vi "Lab Panel V3.5.vi"() -> ()   [LabVIEW 2013]
uses:
  <vilib>/Platform/TimedLoop/XDataNode/timing_clust.ctl
  <vilib>/Platform/TimedLoop/XDataNode/nitl_modes.ctl
  <vilib>/Platform/TimedLoop/XDataNode/wakeup.ctl
  Global 1.vi
  <vilib>/platform/TimedLoop/XDataNode/XDataNode.xnode
  <vilib>/Platform/TimedLoop/XDataNode/XDNodeRunTimeDep.lvlib
panel:
  out "TEMP update":bool
  out "AI update":bool
  in  "stop":bool
  in  "Tab Control 2":T1(tab)
  out "SIG LAB05-2":T2 {"PF" format="%.2f"; "AMPS" format="%.1f"}
  out "SIG LAB05-1":T2 {"PF" format="%.2f"; "AMPS" format="%.1f"}
  out "SIG LAB04-2":T2 {"PF" format="%.2f"; "AMPS" format="%.1f"}
  out "SIG LAB04-1":T2 {"PF" format="%.2f"; "AMPS" format="%.1f"}
  out "SIG LAB03-2":T2 {"PF" format="%.2f"; "AMPS" format="%.1f"}
  out "SIG LAB03-1":T2 {"PF" format="%.2f"; "AMPS" format="%.1f"}
  out "SIG LAB02-2":T2 {"PF" format="%.2f"; "AMPS" format="%.1f"}
  in  "RUN LAB01-1":bool
  in  "O/I  LAB05-1":bool
  in  "O/I  LAB05-2":bool
  in  "O/I  LAB04-1":bool
  in  "O/I  LAB04-2":bool
  in  "O/I  LAB02-1":bool
  in  "O/I  LAB02-2":bool
  in  "O/I  LAB01-2":bool
  in  "O/I  LAB01-1":bool
  in  "O/I  LAB03-1":bool
  in  "RUN LAB05-2":bool
  in  "RUN LAB05-1":bool
  in  "RUN LAB04-2":bool
  in  "RUN LAB04-1":bool
  in  "RUN LAB03-2":bool
  in  "RUN LAB03-1":bool
  in  "RUN LAB02-2":bool
  in  "RUN LAB02-1":bool
  in  "RUN LAB01-2":bool
  in  "SELECT LAB05-2":T3(radio)
  in  "SELECT LAB05-1":T3(radio)
  in  "SELECT LAB04-2":T3(radio)
  in  "SELECT LAB04-1":T3(radio)
  in  "SELECT LAB03-2":T3(radio)
  in  "SELECT LAB03-1":T3(radio)
  in  "SELECT LAB02-2":T3(radio)
  in  "SELECT LAB02-1":T3(radio)
  in  "SELECT LAB01-2":T3(radio)
  in  "SELECT LAB01-1":T3(radio)
  in  "O/I  LAB03-2":bool
  out "SIG LAB01-1":T2 {"PF" format="%.2f"; "AMPS" format="%.1f"}
  out "SIG LAB01-2":T2 {"PF" format="%.2f"; "AMPS" format="%.1f"}
  out "SIG LAB02-1":T2 {"PF" format="%.2f"; "AMPS" format="%.1f"}
  out "DISP LAB05-2":T4 {"MINS" format="%.2g"}
  out "DISP LAB05-1":T4 {"MINS" format="%.2g"}
  out "DISP LAB04-2":T4 {"MINS" format="%.2g"}
  out "DISP LAB04-1":T4 {"MINS" format="%.2g"}
  out "DISP LAB03-2":T4 {"MINS" format="%.2g"}
  out "DISP LAB03-1":T4 {"MINS" format="%.2g"}
  in  "SET LAB05-2":T5={"NAME"="", "DESCRIPTION"="", "CYCLES"=5.0, "T-RISE mins"=0.0, "T-RISE deg C"=0.0} {"CYCLES" min=5.0 step=1.0}
  in  "SET LAB05-1":T5={"NAME"="", "DESCRIPTION"="", "CYCLES"=5.0, "T-RISE mins"=0.0, "T-RISE deg C"=0.0} {"CYCLES" min=5.0 step=1.0}
  in  "SET LAB04-2":T5={"NAME"="", "DESCRIPTION"="", "CYCLES"=5.0, "T-RISE mins"=0.0, "T-RISE deg C"=0.0} {"CYCLES" min=5.0 step=1.0}
  in  "SET LAB04-1":T5={"NAME"="", "DESCRIPTION"="", "CYCLES"=5.0, "T-RISE mins"=0.0, "T-RISE deg C"=0.0} {"CYCLES" min=5.0 step=1.0}
  in  "SET LAB03-2":T5={"NAME"="", "DESCRIPTION"="", "CYCLES"=5.0, "T-RISE mins"=0.0, "T-RISE deg C"=0.0} {"CYCLES" min=5.0 step=1.0}
  in  "SET LAB03-1":T5={"NAME"="", "DESCRIPTION"="", "CYCLES"=5.0, "T-RISE mins"=0.0, "T-RISE deg C"=0.0} {"CYCLES" min=5.0 step=1.0}
  out "DISP LAB02-2":T4 {"MINS" format="%.2g"}
  out "DISP LAB02-1":T4 {"MINS" format="%.2g"}
  in  "SET LAB02-2":T5={"NAME"="", "DESCRIPTION"="", "CYCLES"=5.0, "T-RISE mins"=0.0, "T-RISE deg C"=0.0} {"CYCLES" min=5.0 step=1.0}
  in  "SET LAB02-1":T5={"NAME"="", "DESCRIPTION"="", "CYCLES"=5.0, "T-RISE mins"=0.0, "T-RISE deg C"=0.0} {"CYCLES" min=5.0 step=1.0}
  out "RESULT LAB05-2":bool
  out "RESULT LAB05-1":bool
  out "RESULT LAB04-2":bool
  out "RESULT LAB04-1":bool
  out "RESULT LAB03-2":bool
  out "RESULT LAB03-1":bool
  out "RESULT LAB02-2":bool
  out "RESULT LAB02-1":bool
  out "RESULT LAB01-2":bool
  out "RESULT LAB01-1":bool
  in  "SET LAB01-1":T5={"NAME"="", "DESCRIPTION"="", "CYCLES"=5.0, "T-RISE mins"=0.0, "T-RISE deg C"=0.0} {"CYCLES" min=5.0 step=1.0}
  in  "SET LAB01-2":T5={"NAME"="", "DESCRIPTION"="", "CYCLES"=5.0, "T-RISE mins"=0.0, "T-RISE deg C"=0.0} {"CYCLES" min=5.0 step=1.0}
  out "DISP LAB01-1":T4 {"MINS" format="%.2g"}
  out "DISP LAB01-2":T4 {"MINS" format="%.2f"}
  out "TEMP RISE LAB05-2":cluster{"TL":dbl, "TN":dbl}
  out "TEMP RISE LAB05-1":cluster{"TL":dbl, "TN":dbl}
  out "TEMP RISE LAB04-2":cluster{"TL":dbl, "TN":dbl}
  out "TEMP RISE LAB04-1":cluster{"TL":dbl, "TN":dbl}
  out "TEMP RISE LAB03-2":cluster{"TL":dbl, "TN":dbl}
  out "TEMP RISE LAB03-1":cluster{"TL":dbl, "TN":dbl}
  out "TEMP RISE LAB02-2":cluster{"TL":dbl, "TN":dbl}
  out "TEMP RISE LAB02-1":cluster{"TL":dbl, "TN":dbl}
  out "TEMP RISE LAB01-2":cluster{"TL":dbl, "TN":dbl}
  out "TEMP RISE LAB01-1":cluster{"TL":dbl, "TN":dbl}
  in  "JIG OFF TIME (S)":dbl=2.0 min=2.0 max=10.0 step=0.5 format="%.1g"
  in  "JIG ON TIME (S)":dbl=1.0 min=1.0 max=10.0 step=0.5 format="%.1g"
  out "JIG LAB05-2":bool
  out "JIG LAB05-1":bool
  out "JIG LAB04-2":bool
  out "JIG LAB04-1":bool
  out "JIG LAB03-2":bool
  out "JIG LAB03-1":bool
  out "JIG LAB02-2":bool
  out "JIG LAB02-1":bool
  out "JIG LAB01-2":bool
  out "JIG LAB01-1":bool
  out "TEMP START LAB01-1":cluster{"TL":dbl, "TN":dbl}
  out "TEMP START LAB02-1":cluster{"TL":dbl, "TN":dbl}
  out "TEMP START LAB03-1":cluster{"TL":dbl, "TN":dbl}
  out "TEMP START LAB04-1":cluster{"TL":dbl, "TN":dbl}
  out "TEMP START LAB01-2":cluster{"TL":dbl, "TN":dbl}
  out "TEMP START LAB02-2":cluster{"TL":dbl, "TN":dbl}
  out "TEMP START LAB03-2":cluster{"TL":dbl, "TN":dbl}
  out "TEMP START LAB04-2":cluster{"TL":dbl, "TN":dbl}
  out "TEMP START LAB05-2":cluster{"TL":dbl, "TN":dbl}
  out "TEMP START LAB05-1":cluster{"TL":dbl, "TN":dbl}
  in  "MAIL SETTINGS":T6
  out "MAIL REPORT":string
  in  "TO (string):":string
  in  "Send Mail Now":bool
  in  "Auto Mail Send":bool
  in  "Network Directory":path
  out "CAL LAB01":T7 {"2 (TN) cal" min=0.0 step=0.01 format="%.2f"; "2 (TL) cal" min=0.0 step=0.01 format="%.2f"; "2 (PF) cal" min=0.0 step=0.01 format="%.2f"; "2 (V) cal" min=0.0 step=0.01 format="%.2f"; "2 (A) cal" min=0.0 step=0.01 format="%.2f"; "1 (TN) cal" min=0.0 step=0.01 format="%.2f"; "1 (TL) cal" min=0.0 step=0.01 format="%.2f"; "1 (PF) cal" min=0.0 step=0.01 format="%.2f"; "1 (V) cal" min=0.0 step=0.01 format="%.2f"; "1  (A) cal" min=0.0 step=0.01 format="%.2f"}
  out "CAL LAB03":T7 {"2 (TN) cal" min=0.0 step=0.01 format="%.2f"; "2 (TL) cal" min=0.0 step=0.01 format="%.2f"; "2 (PF) cal" min=0.0 step=0.01 format="%.2f"; "2 (V) cal" min=0.0 step=0.01 format="%.2f"; "2 (A) cal" min=0.0 step=0.01 format="%.2f"; "1 (TN) cal" min=0.0 step=0.01 format="%.2f"; "1 (TL) cal" min=0.0 step=0.01 format="%.2f"; "1 (PF) cal" min=0.0 step=0.01 format="%.2f"; "1 (V) cal" min=0.0 step=0.01 format="%.2f"; "1  (A) cal" min=0.0 step=0.01 format="%.2f"}
  out "CAL LAB02":T8 {"2 (TN) cal" min=0.0 step=0.01 format="%.2f"; "2 (TL) cal" min=0.0 step=0.01 format="%.2f"; "2 (PF) cal" min=0.0 step=0.01 format="%.2f"; "2 (V) cal" min=0.0 step=0.01 format="%.2f"; "2 (A) cal" min=0.0 step=0.01 format="%.2f"; "1 (TN) cal" min=0.0 step=0.01 format="%.2f"; "1 (TL) cal" min=0.0 step=0.01 format="%.2f"; "1 (PF) cal" min=0.0 step=0.01 format="%.2f"; "1 (V) cal" min=0.0 step=0.01 format="%.2f"; "1 (A) cal" min=0.0 step=0.01 format="%.2f"}
  out "CAL LAB05":T7 {"2 (TN) cal" min=0.0 step=0.01 format="%.2f"; "2 (TL) cal" min=0.0 step=0.01 format="%.2f"; "2 (PF) cal" min=0.0 step=0.01 format="%.2f"; "2 (V) cal" min=0.0 step=0.01 format="%.2f"; "2 (A) cal" min=0.0 step=0.01 format="%.2f"; "1 (TN) cal" min=0.0 step=0.01 format="%.2f"; "1 (TL) cal" min=0.0 step=0.01 format="%.2f"; "1 (PF) cal" min=0.0 step=0.01 format="%.2f"; "1 (V) cal" min=0.0 step=0.01 format="%.2f"; "1  (A) cal" min=0.0 step=0.01 format="%.2f"}
  out "CAL LAB04":T7 {"2 (TN) cal" min=0.0 step=0.01 format="%.2f"; "2 (TL) cal" min=0.0 step=0.01 format="%.2f"; "2 (PF) cal" min=0.0 step=0.01 format="%.2f"; "2 (V) cal" min=0.0 step=0.01 format="%.2f"; "2 (A) cal" min=0.0 step=0.01 format="%.2f"; "1 (TN) cal" min=0.0 step=0.01 format="%.2f"; "1 (TL) cal" min=0.0 step=0.01 format="%.2f"; "1 (PF) cal" min=0.0 step=0.01 format="%.2f"; "1 (V) cal" min=0.0 step=0.01 format="%.2f"; "1  (A) cal" min=0.0 step=0.01 format="%.2f"}
  out "calibration file error out":errorcluster
  in  "CALIBRATE":bool
  in  "SHOW ADMIN PAGE":bool
  out "FAIL LAB05-2":cluster{"LO":dbl, "HI":dbl}
  out "FAIL LAB05-1":cluster{"LO":dbl, "HI":dbl}
  out "FAIL LAB04-2":cluster{"LO":dbl, "HI":dbl}
  out "FAIL LAB04-1":cluster{"LO":dbl, "HI":dbl}
  out "FAIL LAB03-2":cluster{"LO":dbl, "HI":dbl}
  out "FAIL LAB03-1":cluster{"LO":dbl, "HI":dbl}
  out "FAIL LAB02-2":cluster{"LO":dbl, "HI":dbl}
  out "FAIL LAB02-1":cluster{"LO":dbl, "HI":dbl}
  out "FAIL LAB01-2":cluster{"LO":dbl, "HI":dbl}
  out "FAIL LAB01-1":cluster{"LO":dbl, "HI":dbl}
  in  "C drive data root dir":path
  out "run lab05-2":bool
  out "run lab05-1":bool
  out "run lab04-2":bool
  out "run lab04-1":bool
  out "run lab03-2":bool
  out "run lab03-1":bool
  out "run lab02-2":bool
  out "run lab02-1":bool
  out "run lab01-2":bool
  out "run lab01-1":bool
  out "stop2":bool
  in  "Tab Control":T9(tab)
  out "LAB01-2 (GRAPH)":dynamicdata(graph)
  out "LAB01-1 (GRAPH)":dynamicdata(graph)
  out "LAB02-2 (GRAPH)":dynamicdata(graph)
  out "LAB02-1 (GRAPH)":dynamicdata(graph)
  out "LAB03-2 (GRAPH)":dynamicdata(graph)
  out "LAB03-1 (GRAPH)":dynamicdata(graph)
  out "LAB04-2 (GRAPH)":dynamicdata(graph)
  out "LAB04-1 (GRAPH)":dynamicdata(graph)
  out "LAB05-2 (GRAPH)":dynamicdata(graph)
  out "LAB05-1 (GRAPH)":dynamicdata(graph)
  out "LAB05 TEMP":T10
  out "LAB04 TEMP":T10
  out "LAB02 TEMP":T10
  out "LAB01 TEMP":T10
  out "LAB03 TEMP":T10
  out "Analog Error Array":errorcluster[](array[cluster])
  out "AI loop time":dbl format="%.6g"
  out "loops":dbl
  in  "loop  delay(mS)":dbl
  out "on loops":dbl
  out "off loops":dbl
  out "jig cycle":dbl
  out "TDMS LAB01-1":refnum<k34>
  out "data file error":errorcluster
  out "TDMS LAB02-1":refnum<k34>
  out "TDMS LAB01-2":refnum<k34>
  out "TDMS LAB02-2":refnum<k34>
  out "TDMS LAB03-1":refnum<k34>
  out "TDMS LAB03-2":refnum<k34>
  out "TDMS LAB04-1":refnum<k34>
  out "TDMS LAB04-2":refnum<k34>
  out "TDMS LAB05-1":refnum<k34>
  out "TDMS LAB05-2":refnum<k34>
  out "mail control":string
  # "LAB01"
  # "LAB02"
  # "LAB05"
  # "LAB03"
  # "LAB04"
  # "LAB01"
  # "LAB02"
  # "LAB03"
  # "LAB04"
  # "LAB05"
  # "JIG SET"
  # "(Enter recipients address seperated by comma)"
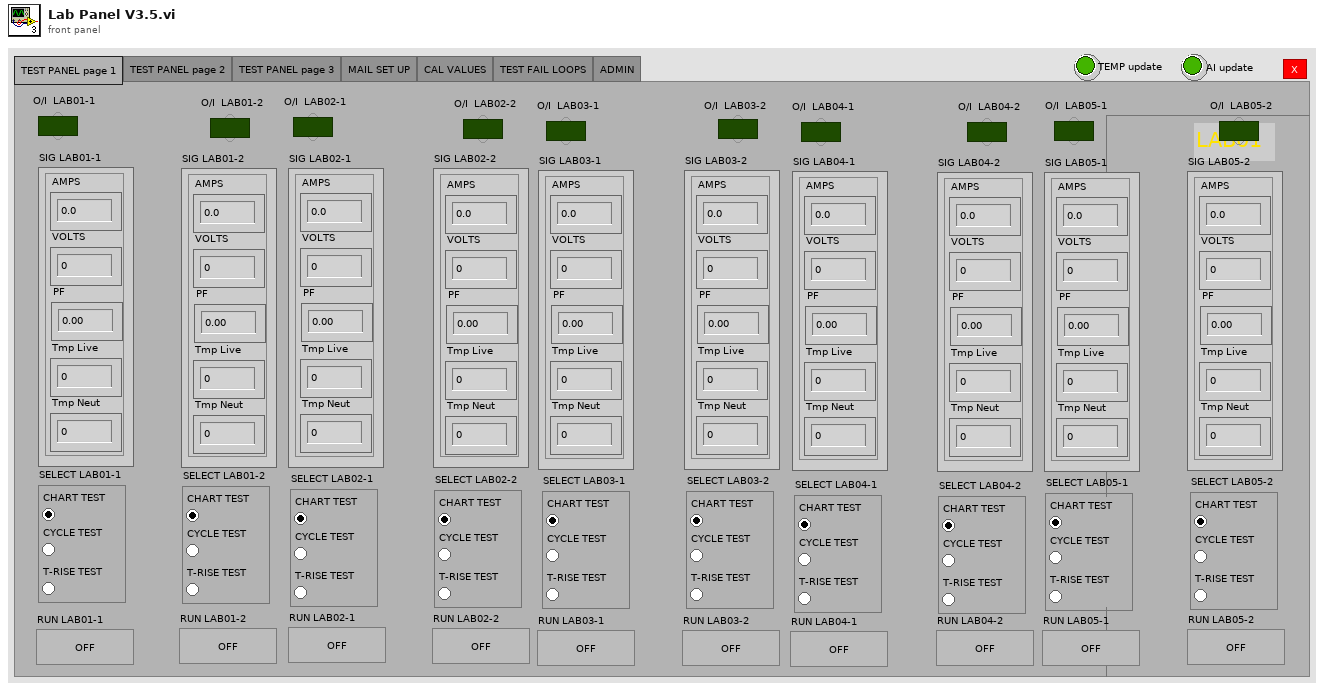
[diagram p1: front panel]
types:
  T1 = enum32{"TEST PANEL page 1", "TEST PANEL page 2", "TEST PANEL page 3", "MAIL SET UP", "CAL VALUES", "TEST FAIL LOOPS", "ADMIN"}
  T2 = cluster{"AMPS":dbl, "VOLTS":dbl, "PF":dbl, "Tmp Live":dbl, "Tmp Neut":dbl}
  T3 = enum32{"CHART TEST", "CYCLE TEST", "T-RISE TEST"}
  T4 = cluster{"CYCLE":dbl, "MINS":dbl, "STATUS":string}
  T5 = cluster{"NAME":string, "DESCRIPTION":string, "CYCLES":dbl, "T-RISE mins":dbl, "T-RISE deg C":dbl}
  T6 = cluster{"OUT SERVER ADDRESS":string, "FROM ACCOUNT":string, "USER NAME":string, "PASSWORD":string, "TEST MAIL":bool, "TEST MAIL STATUS":string, "mail error":errorcluster}
  T7 = cluster{"1  (A) cal":dbl, "1 (V) cal":dbl, "1 (PF) cal":dbl, "1 (TL) cal":dbl, "1 (TN) cal":dbl, "2 (A) cal":dbl, "2 (V) cal":dbl, "2 (PF) cal":dbl, "2 (TL) cal":dbl, "2 (TN) cal":dbl}
  T8 = cluster{"1 (A) cal":dbl, "1 (V) cal":dbl, "1 (PF) cal":dbl, "1 (TL) cal":dbl, "1 (TN) cal":dbl, "2 (A) cal":dbl, "2 (V) cal":dbl, "2 (PF) cal":dbl, "2 (TL) cal":dbl, "2 (TN) cal":dbl}
  T9 = enum32{"LAB01", "LAB02", "LAB03", "LAB04", "LAB05", "TEMPERATURE", "ERROR"}
  T10 = cluster{"T1 Live":dbl, "T1 Neut":dbl, "T2 Live":dbl, "T2 Neut":dbl, "ID":dbl, "ER":dbl}
  T11 = enum8{"Enabled", "Disabled", "Disabled and Grayed Out"}
  T12 = typedef "XDNodeRunTimeDep.lvlib/timing_clust.ctl" = cluster{"Expected End [f-1]":u64, "Actual End [f-1]":u64, "Finished Late? [f-1]":bool, "Expected End [i-1]":u64, "Actual End [i-1]":u64, "Finished Late? [i-1]":bool, "Expected Start [i]":u64, "Actual Start [i]":u64, "Expected Start [f]":u64, "Actual Start [f]":u64, "Source Name":string, "Structure Name":string, "Period":i64, "Deadline":i64, "Offset":i64, "Start":i64, "Priority":i32, "Timeout":i32, "Mode":T13, "Wakeup Reason":T14, "Error":errorcluster, "Source Type":string, "Secondary Source Type":string, "Global End Time":u64, "Global Start Time":u64, "Frame Duration":u64, "Iteration Duration":u64, "Assigned CPU":i32, "I/O Scan Engine Mode":u32}
  T13 = typedef "XDNodeRunTimeDep.lvlib/nitl_modes.ctl" = enum32{"No Change", "Process missed periods, maintain original phase", "Discard missed periods, maintain original phase", "Process missed periods, ignore original phase", "Discard missed periods, ignore original phase"}
  T14 = typedef "XDNodeRunTimeDep.lvlib/wakeup.ctl" = enum32{"Normal", "Aborted", "Asynchronous wakeup", "Timing source error", "Timed loop error", "Timeout"}
  T15 = enum16{"open", "open or create", "create or replace", "create", "open (read-only)"}
  T16 = enum16{"open", "replace", "create", "open or create", "replace or create", "replace or create with confirmation"}
  T17 = cluster{"SET LAB01-1":cluster{"NAME":string, "DESCRIPTION":string, "CYCLES":dbl, "T-RISE mins":dbl, "T-RISE deg C":dbl}, "SET LAB01-2":cluster{"NAME":string, "DESCRIPTION":string, "CYCLES":dbl, "T-RISE mins":dbl, "T-RISE deg C":dbl}, "SET LAB02-1":cluster{"NAME":string, "DESCRIPTION":string, "CYCLES":dbl, "T-RISE mins":dbl, "T-RISE deg C":dbl}, "SET LAB02-2":cluster{"NAME":string, "DESCRIPTION":string, "CYCLES":dbl, "T-RISE mins":dbl, "T-RISE deg C":dbl}, "SET LAB03-1":cluster{"NAME":string, "DESCRIPTION":string, "CYCLES":dbl, "T-RISE mins":dbl, "T-RISE deg C":dbl}, "SET LAB03-2":cluster{"NAME":string, "DESCRIPTION":string, "CYCLES":dbl, "T-RISE mins":dbl, "T-RISE deg C":dbl}, "SET LAB04-1":cluster{"NAME":string, "DESCRIPTION":string, "CYCLES":dbl, "T-RISE mins":dbl, "T-RISE deg C":dbl}, "SET LAB04-2":cluster{"NAME":string, "DESCRIPTION":string, "CYCLES":dbl, "T-RISE mins":dbl, "T-RISE deg C":dbl}, "SET LAB05-1":cluster{"NAME":string, "DESCRIPTION":string, "CYCLES":dbl, "T-RISE mins":dbl, "T-RISE deg C":dbl}, "SET LAB05-2":cluster{"NAME":string, "DESCRIPTION":string, "CYCLES":dbl, "T-RISE mins":dbl, "T-RISE deg C":dbl}, "Network Directory":path, "C drive data root dir":path}
  T18 = cluster{"MAIL SETTINGS":cluster{"OUT SERVER ADDRESS":string, "FROM ACCOUNT":string, "USER NAME":string, "PASSWORD":string, "TEST MAIL":bool, "TEST MAIL STATUS":string, "mail error":errorcluster}, "Auto Mail Send":bool, string}
  T19 = cluster{"T1":dbl, "T2":dbl, "T3":dbl, "T4":dbl, "ID":dbl, "ER":dbl}
  T20 = cluster{"LAB01-1 (A)":dbl, "LAB01-1 (V)":dbl, "LAB01-1 (PF)":dbl, "LAB01-2 (A)":dbl, "LAB01-2 (V)":dbl, "LAB01-2 (PF)":dbl}
  T21 = cluster{"LAB02-1 (A)":dbl, "LAB02-1 (V)":dbl, "LAB02-1 (PF)":dbl, "LAB02-2 (A)":dbl, "LAB02-2 (V)":dbl, "LAB02-2 (PF)":dbl}
  T22 = cluster{"LAB03-1 (A)":dbl, "LAB03-1 (V)":dbl, "LAB03-1 (PF)":dbl, "LAB03-2 (A)":dbl, "LAB03-2 (V)":dbl, "LAB03-2 (PF)":dbl}
  T23 = cluster{"LAB04-1 (A)":dbl, "LAB04-1 (V)":dbl, "LAB04-1 (PF)":dbl, "LAB04-2 (A)":dbl, "LAB04-2 (V)":dbl, "LAB04-2 (PF)":dbl}
  T24 = cluster{"LAB05-1 (A)":dbl, "LAB05-1 (V)":dbl, "LAB05-1 (PF)":dbl, "LAB05-2 (A)":dbl, "LAB05-2 (V)":dbl, "LAB05-2 (PF)":dbl}
  T25 = cluster{"FAIL LAB01-1":cluster{"LO":dbl, "HI":dbl}, "SIG LAB01-1":cluster{"AMPS":dbl, "VOLTS":dbl, "PF":dbl, "Tmp Live":dbl, "Tmp Neut":dbl}, "TEMP START LAB01-1":cluster{"TL":dbl, "TN":dbl}, "DISP LAB01-1":cluster{"CYCLE":dbl, "MINS":dbl, "STATUS":string}, "SET LAB01-1":cluster{"NAME":string, "DESCRIPTION":string, "CYCLES":dbl, "T-RISE mins":dbl, "T-RISE deg C":dbl}, "TDMS LAB01-1":refnum<k34>}
  T26 = cluster{"FAIL LAB01-2":cluster{"LO":dbl, "HI":dbl}, "SIG LAB01-2":cluster{"AMPS":dbl, "VOLTS":dbl, "PF":dbl, "Tmp Live":dbl, "Tmp Neut":dbl}, "TEMP START LAB01-2":cluster{"TL":dbl, "TN":dbl}, "DISP LAB01-2":cluster{"CYCLE":dbl, "MINS":dbl, "STATUS":string}, "SET LAB01-2":cluster{"NAME":string, "DESCRIPTION":string, "CYCLES":dbl, "T-RISE mins":dbl, "T-RISE deg C":dbl}, "TDMS LAB01-2":refnum<k34>}
  T27 = cluster{"FAIL LAB02-1":cluster{"LO":dbl, "HI":dbl}, "SIG LAB02-1":cluster{"AMPS":dbl, "VOLTS":dbl, "PF":dbl, "Tmp Live":dbl, "Tmp Neut":dbl}, "TEMP START LAB02-1":cluster{"TL":dbl, "TN":dbl}, "DISP LAB02-1":cluster{"CYCLE":dbl, "MINS":dbl, "STATUS":string}, "SET LAB02-1":cluster{"NAME":string, "DESCRIPTION":string, "CYCLES":dbl, "T-RISE mins":dbl, "T-RISE deg C":dbl}, "TDMS LAB02-1":refnum<k34>}
  T28 = cluster{"FAIL LAB02-2":cluster{"LO":dbl, "HI":dbl}, "SIG LAB02-2":cluster{"AMPS":dbl, "VOLTS":dbl, "PF":dbl, "Tmp Live":dbl, "Tmp Neut":dbl}, "TEMP START LAB02-2":cluster{"TL":dbl, "TN":dbl}, "DISP LAB02-2":cluster{"CYCLE":dbl, "MINS":dbl, "STATUS":string}, "SET LAB02-2":cluster{"NAME":string, "DESCRIPTION":string, "CYCLES":dbl, "T-RISE mins":dbl, "T-RISE deg C":dbl}, "TDMS LAB02-2":refnum<k34>}
  T29 = cluster{"FAIL LAB03-1":cluster{"LO":dbl, "HI":dbl}, "SIG LAB03-1":cluster{"AMPS":dbl, "VOLTS":dbl, "PF":dbl, "Tmp Live":dbl, "Tmp Neut":dbl}, "TEMP START LAB03-1":cluster{"TL":dbl, "TN":dbl}, "DISP LAB03-1":cluster{"CYCLE":dbl, "MINS":dbl, "STATUS":string}, "SET LAB03-1":cluster{"NAME":string, "DESCRIPTION":string, "CYCLES":dbl, "T-RISE mins":dbl, "T-RISE deg C":dbl}, "TDMS LAB03-1":refnum<k34>}
  T30 = cluster{"FAIL LAB03-2":cluster{"LO":dbl, "HI":dbl}, "SIG LAB03-2":cluster{"AMPS":dbl, "VOLTS":dbl, "PF":dbl, "Tmp Live":dbl, "Tmp Neut":dbl}, "TEMP START LAB03-2":cluster{"TL":dbl, "TN":dbl}, "DISP LAB03-2":cluster{"CYCLE":dbl, "MINS":dbl, "STATUS":string}, "SET LAB03-2":cluster{"NAME":string, "DESCRIPTION":string, "CYCLES":dbl, "T-RISE mins":dbl, "T-RISE deg C":dbl}, "TDMS LAB03-2":refnum<k34>}
  T31 = cluster{"FAIL LAB04-1":cluster{"LO":dbl, "HI":dbl}, "SIG LAB04-1":cluster{"AMPS":dbl, "VOLTS":dbl, "PF":dbl, "Tmp Live":dbl, "Tmp Neut":dbl}, "TEMP START LAB04-1":cluster{"TL":dbl, "TN":dbl}, "DISP LAB04-1":cluster{"CYCLE":dbl, "MINS":dbl, "STATUS":string}, "SET LAB04-1":cluster{"NAME":string, "DESCRIPTION":string, "CYCLES":dbl, "T-RISE mins":dbl, "T-RISE deg C":dbl}, "TDMS LAB04-1":refnum<k34>}
  T32 = cluster{"FAIL LAB04-2":cluster{"LO":dbl, "HI":dbl}, "SIG LAB04-2":cluster{"AMPS":dbl, "VOLTS":dbl, "PF":dbl, "Tmp Live":dbl, "Tmp Neut":dbl}, "TEMP START LAB04-2":cluster{"TL":dbl, "TN":dbl}, "DISP LAB04-2":cluster{"CYCLE":dbl, "MINS":dbl, "STATUS":string}, "SET LAB04-2":cluster{"NAME":string, "DESCRIPTION":string, "CYCLES":dbl, "T-RISE mins":dbl, "T-RISE deg C":dbl}, "TDMS LAB04-2":refnum<k34>}
  T33 = cluster{"FAIL LAB05-1":cluster{"LO":dbl, "HI":dbl}, "SIG LAB05-1":cluster{"AMPS":dbl, "VOLTS":dbl, "PF":dbl, "Tmp Live":dbl, "Tmp Neut":dbl}, "TEMP START LAB05-1":cluster{"TL":dbl, "TN":dbl}, "DISP LAB05-1":cluster{"CYCLE":dbl, "MINS":dbl, "STATUS":string}, "SET LAB05-1":cluster{"NAME":string, "DESCRIPTION":string, "CYCLES":dbl, "T-RISE mins":dbl, "T-RISE deg C":dbl}, "TDMS LAB05-1":refnum<k34>}
  T34 = cluster{"FAIL LAB05-2":cluster{"LO":dbl, "HI":dbl}, "SIG LAB05-2":cluster{"AMPS":dbl, "VOLTS":dbl, "PF":dbl, "Tmp Live":dbl, "Tmp Neut":dbl}, "TEMP START LAB05-2":cluster{"TL":dbl, "TN":dbl}, "DISP LAB05-2":cluster{"CYCLE":dbl, "MINS":dbl, "STATUS":string}, "SET LAB05-2":cluster{"NAME":string, "DESCRIPTION":string, "CYCLES":dbl, "T-RISE mins":dbl, "T-RISE deg C":dbl}, "TDMS LAB05-2":refnum<k34>}
  T35 = cluster{"MAIL SETTINGS":cluster{"OUT SERVER ADDRESS":string, "FROM ACCOUNT":string, "USER NAME":string, "PASSWORD":string, "TEST MAIL":bool, "TEST MAIL STATUS":string, "mail error":errorcluster}, "Auto Mail Send":bool, "TO (string):":string}
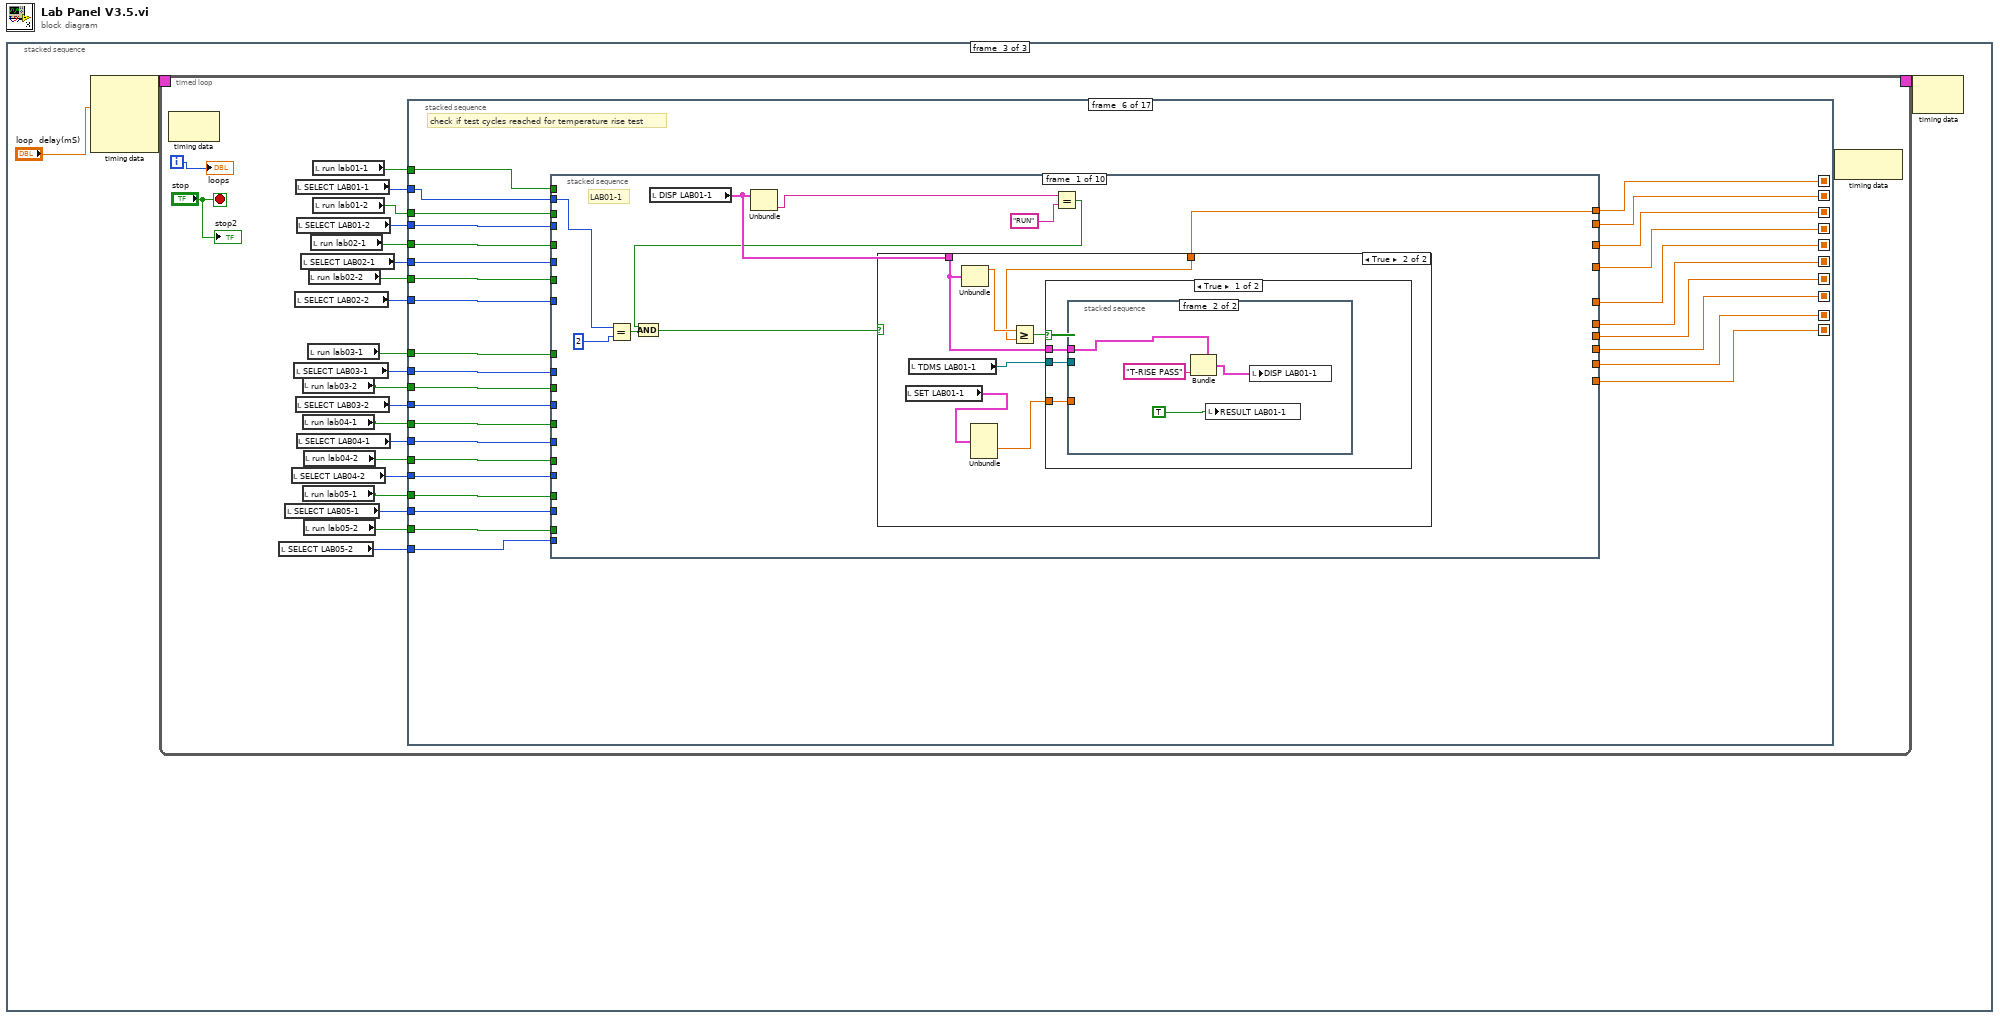
[diagram p0: block diagram]
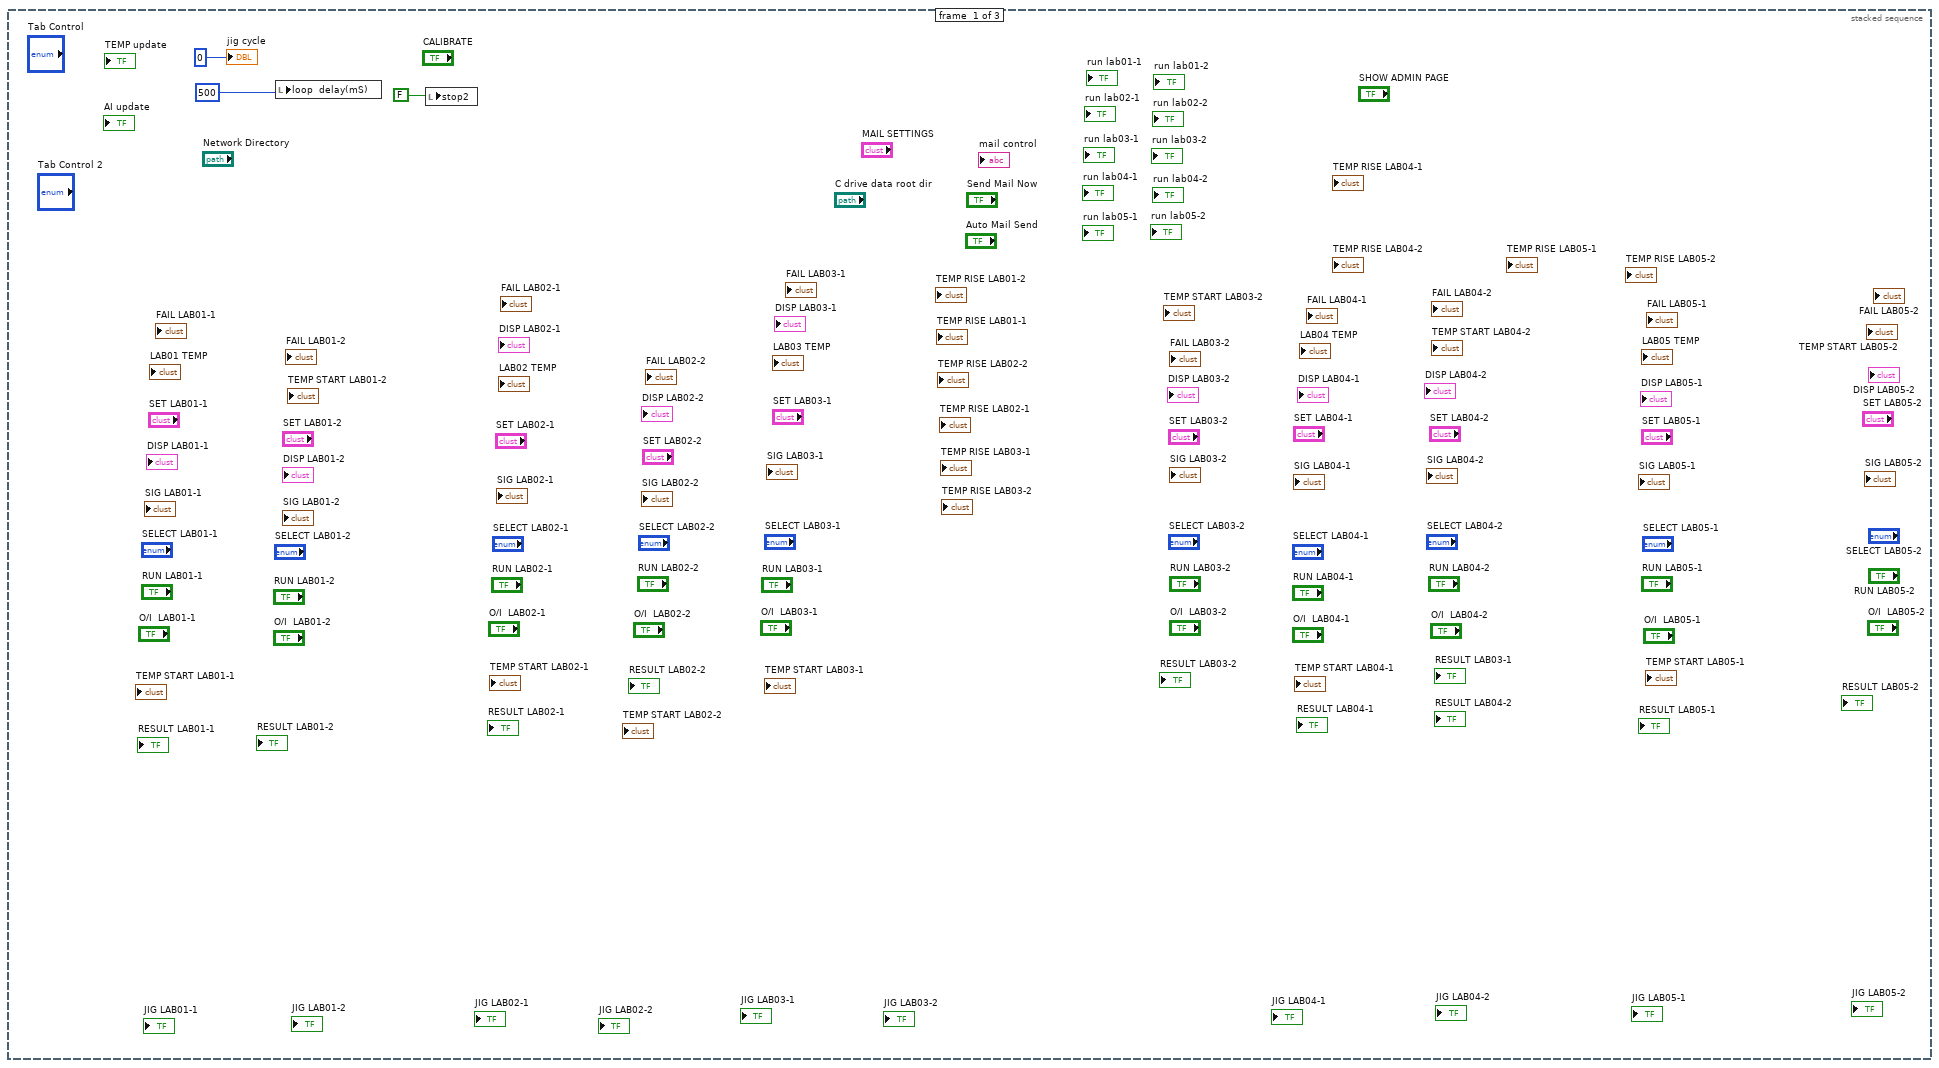
[diagram p2: hidden frame]
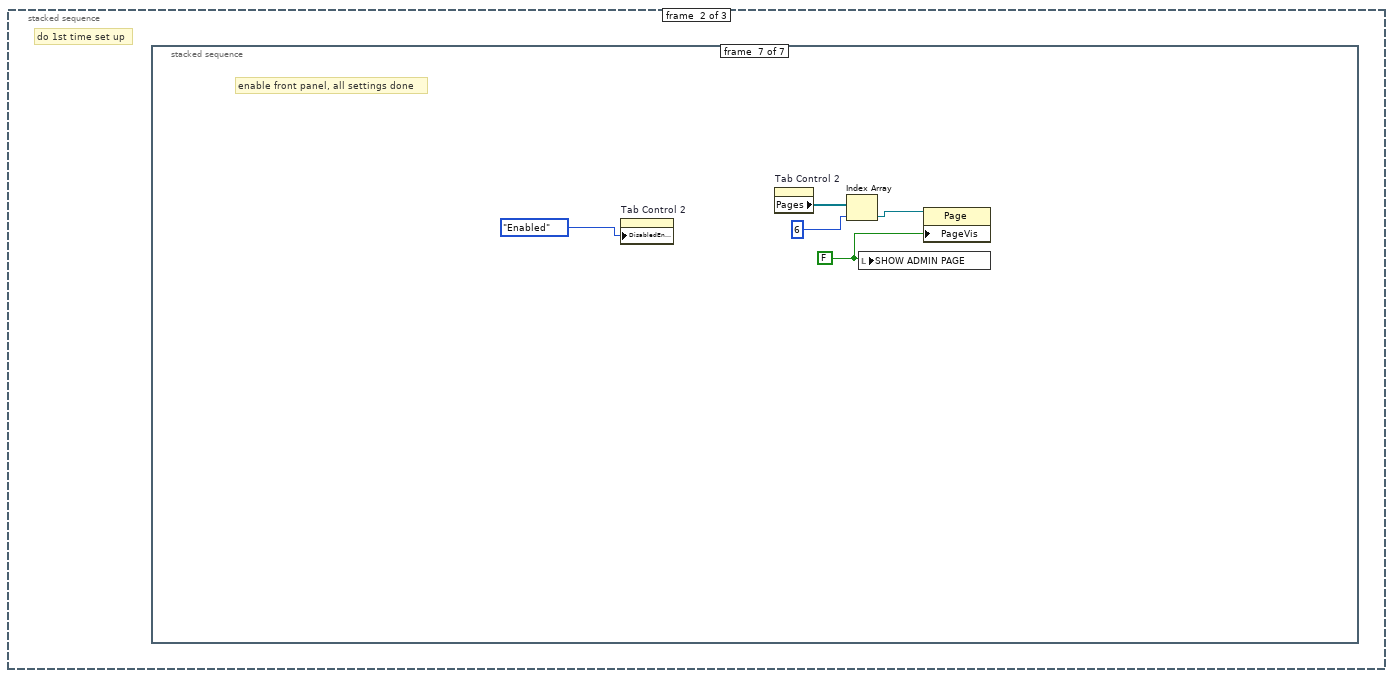
[diagram p3: hidden frame]
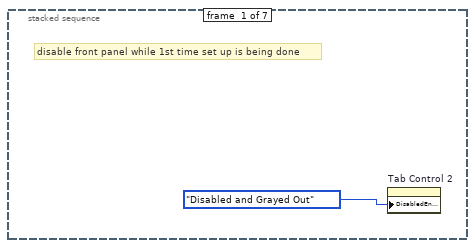
[diagram p4: hidden frame]
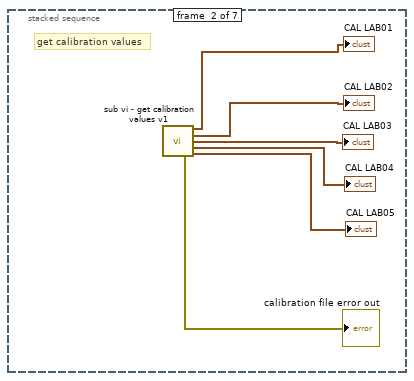
[diagram p5: hidden frame]
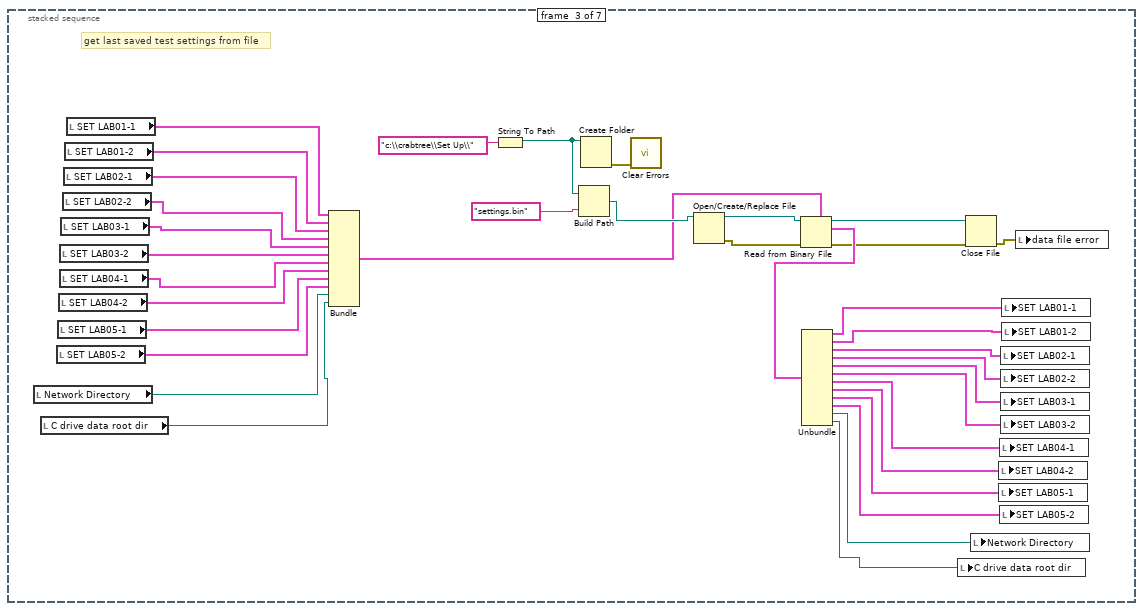
[diagram p6: hidden frame]
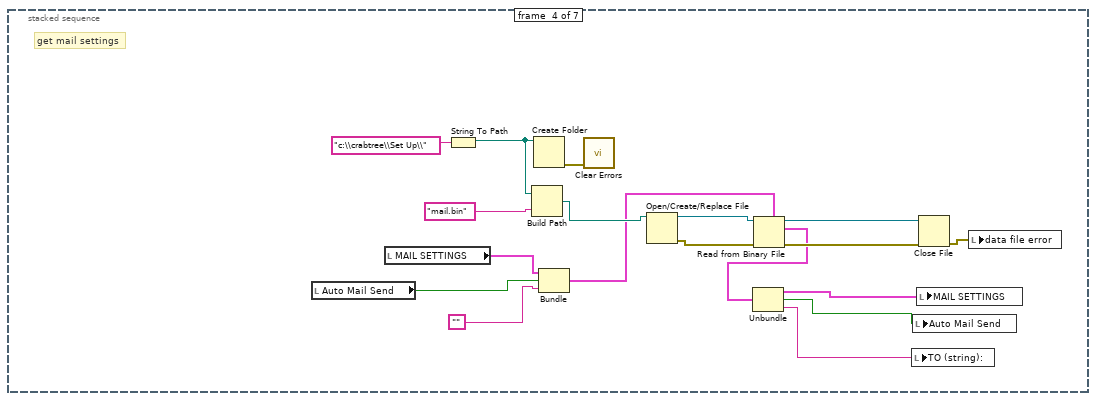
[diagram p7: hidden frame]
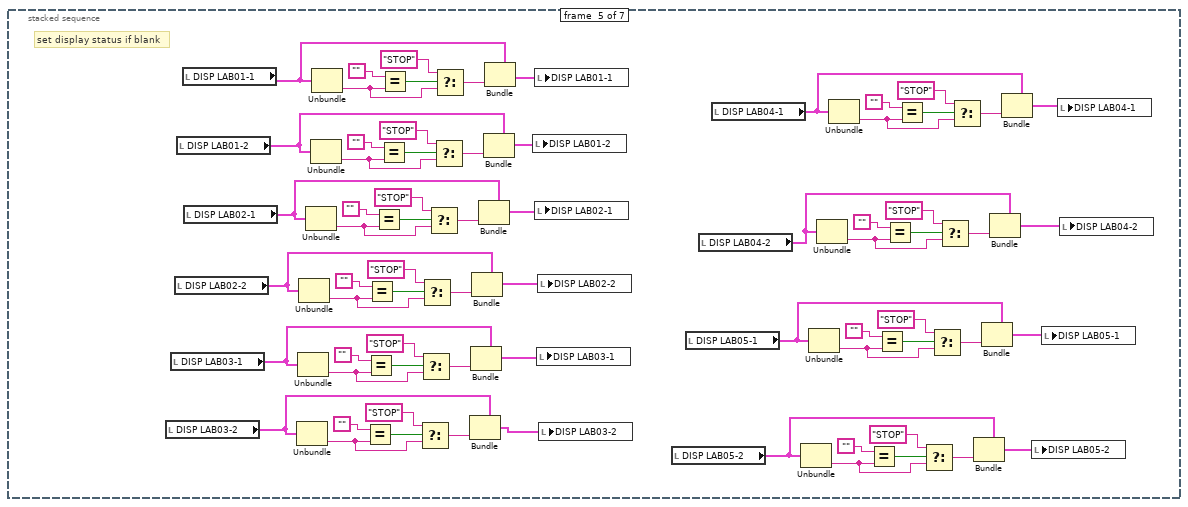
[diagram p8: hidden frame]
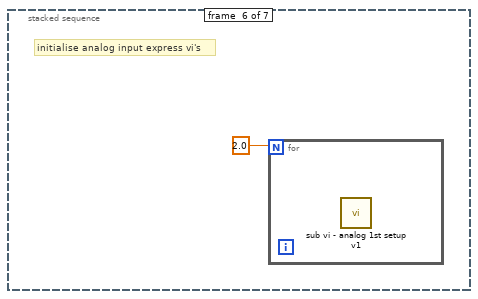
[diagram p9: hidden frame]
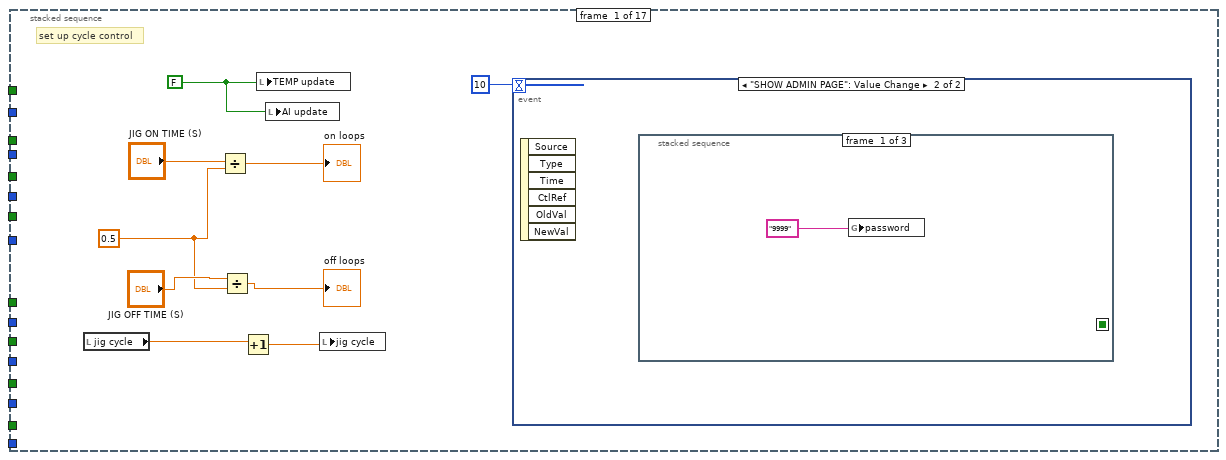
[diagram p10: hidden frame]
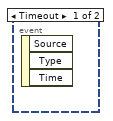
[diagram p11: hidden frame]
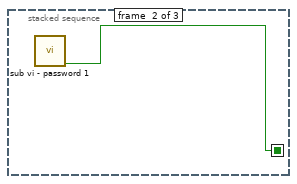
[diagram p12: hidden frame]
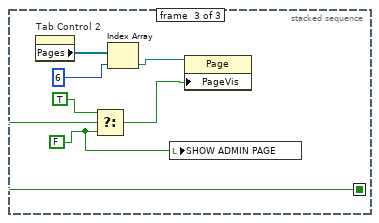
[diagram p13: hidden frame]
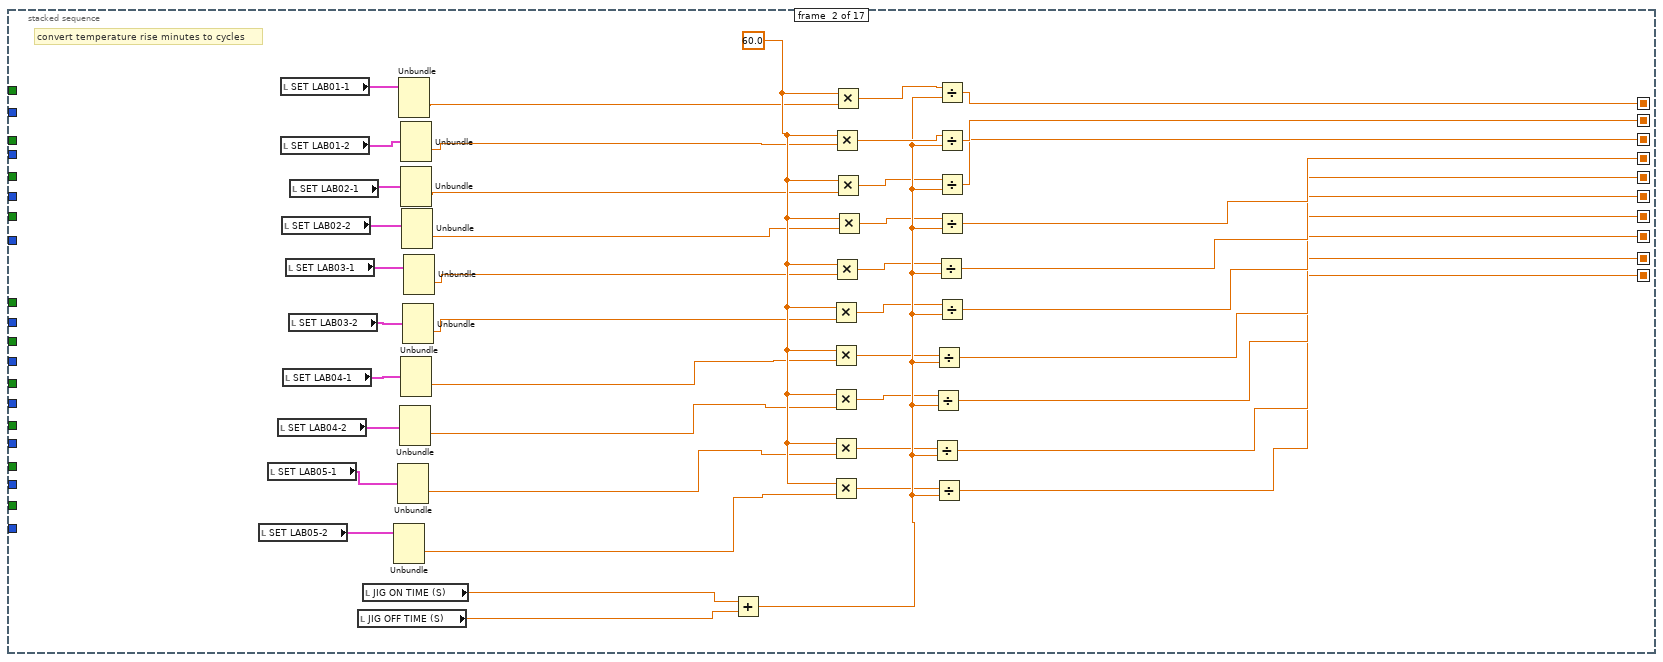
[diagram p14: hidden frame]
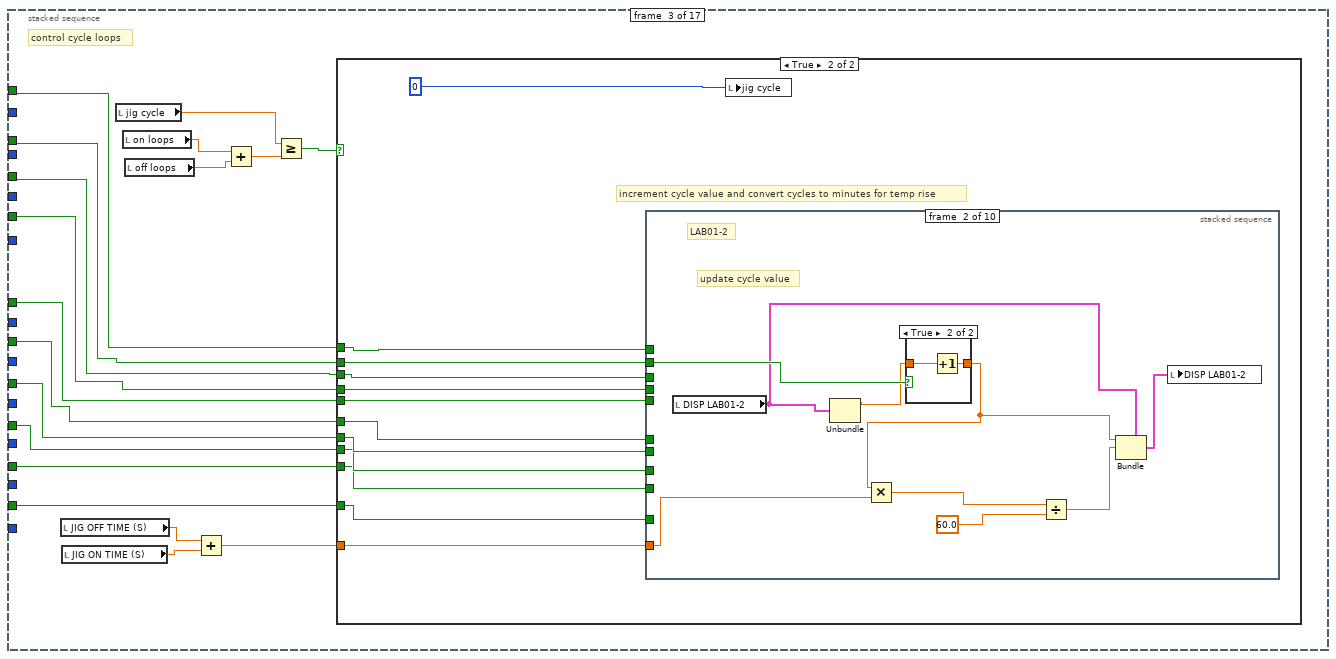
[diagram p15: hidden frame]
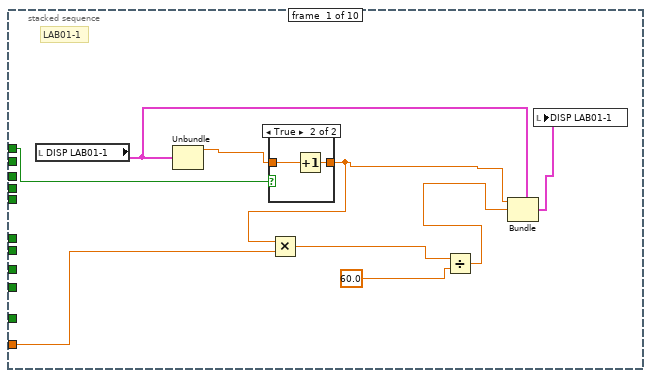
[diagram p17: hidden frame]
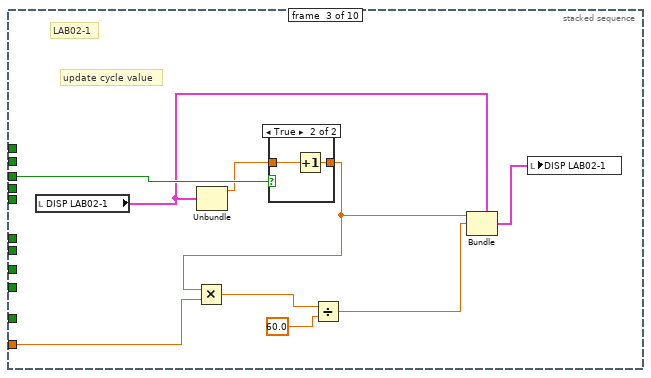
[diagram p20: hidden frame]
diagram:
  n1 = stacked-sequence {
    frame #0 {
      n2 = local write "loop  delay(mS)"(500) -> ()
      n3 = local write "stop2"(FALSE) -> ()
      "jig cycle" <- 0
    }
    frame #1 {
      # "do 1st time set up"
      n4 = stacked-sequence {
        frame #0 {
          # "disable front panel while 1st time set up is being done"
          n5 = property on="Tab Control 2" class="TabCtl (strict)"("DisabledEnum"=T11."Disabled and Grayed Out" ("Disabled")) -> ()  [unwired: 2 in, 2 out]
        }
        frame #1 {
          # "get calibration values"
          n6 = call "sub vi - get calibration values v1.vi"() -> ("LAB01 (CAL)"=→"CAL LAB01":T7, "LAB02 (CAL)"=→"CAL LAB02":T8, "LAB03 (CAL)"=→"CAL LAB03":T7, "LAB04 (CAL)"=→"CAL LAB04":T7, "calibration file error out"=→"calibration file error out":errorcluster, "LAB05 (CAL)"=→"CAL LAB05":T7)  [unwired: 10 in]
        }
        frame #2 {
          # "get last saved test settings from file"
          n7 = local read "Network Directory"() -> (w13:path)
          n8 = local read "C drive data root dir"() -> (w11:path)
          n9 = local read "SET LAB05-2"() -> (w43:T5)
          n10 = local read "SET LAB05-1"() -> (w44:T5)
          n11 = local read "SET LAB04-2"() -> (w45:T5)
          n12 = local read "SET LAB03-2"() -> (w42:T5)
          n13 = local read "SET LAB04-1"() -> (w46:T5)
          n14 = local read "SET LAB03-1"() -> (w41:T5)
          n15 = local read "SET LAB02-2"() -> (w40:T5)
          n16 = local read "SET LAB02-1"() -> (w39:T5)
          n17 = local read "SET LAB01-2"() -> (w38:T5)
          n18 = local read "SET LAB01-1"() -> (w37:T5)
          n19 = Bundle("SET LAB01-1"=w37, "SET LAB01-2"=w38, "SET LAB02-1"=w39, "SET LAB02-2"=w40, "SET LAB03-1"=w41, "SET LAB03-2"=w42, "SET LAB04-1"=w46, "SET LAB04-2"=w45, "SET LAB05-1"=w44, "SET LAB05-2"=w43, "Network Directory"=w13, "C drive data root dir"=w11) -> (w30:T17)  [unwired: 1 in]
          n20 = String To Path(string="c:\\crabtree\\Set Up\\") -> (path=w34:path)
          n21 = Build Path(base path=w34, name or relative path="settings.bin") -> (appended path=w32:path)
          n22 = Create Folder(path (use dialog)=w34) -> (error out=w36:errorcluster)  [unwired: 2 in, 2 out]
          n23 = call <vilib>:"Clear Errors.vi"("error in (no error)"=w36) -> ()  [unwired: 6 in, 1 out]
          n24 = Open/Create/Replace File(file path (use dialog)=w32) -> (refnum out=w29:refnum<file>, error out=w31:errorcluster)  [unwired: 5 in, 1 out]
          n25 = Read from Binary File(5:w30, 8:w31, 11:w29) -> (0:w26:errorcluster, 2:w28:T17, 3:w27:refnum<file>)  [unwired: 3 in, 1 out]
          n26 = Unbundle(w28) -> ("SET LAB01-1"=w24:T5, "SET LAB01-2"=w23:T5, "SET LAB02-1"=w22:T5, "SET LAB02-2"=w21:T5, "SET LAB03-1"=w20:T5, "SET LAB03-2"=w19:T5, "SET LAB04-1"=w18:T5, "SET LAB04-2"=w17:T5, "SET LAB05-1"=w16:T5, "SET LAB05-2"=w15:T5, "Network Directory"=w14:path, "C drive data root dir"=w12:path)
          n27 = local write "C drive data root dir"(w12) -> ()
          n28 = Close File(refnum=w27, error in=w26) -> (error out=w25:errorcluster)  [unwired: 1 out]
          n29 = local write "Network Directory"(w14) -> ()
          n30 = local write "SET LAB04-2"(w17) -> ()
          n31 = local write "SET LAB05-1"(w16) -> ()
          n32 = local write "SET LAB04-1"(w18) -> ()
          n33 = local write "SET LAB05-2"(w15) -> ()
          n34 = local write "SET LAB02-1"(w22) -> ()
          n35 = local write "SET LAB02-2"(w21) -> ()
          n36 = local write "SET LAB03-1"(w20) -> ()
          n37 = local write "SET LAB03-2"(w19) -> ()
          n38 = local write "SET LAB01-1"(w24) -> ()
          n39 = local write "SET LAB01-2"(w23) -> ()
          n40 = local write "data file error"(w25) -> ()
        }
        frame #3 {
          # "get mail settings"
          n41 = local read "Auto Mail Send"() -> (w50:bool)
          n42 = local read "MAIL SETTINGS"() -> (w54:T6)
          n43 = String To Path(string="c:\\crabtree\\Set Up\\") -> (path=w62:path)
          n44 = Build Path(base path=w62, name or relative path="mail.bin") -> (appended path=w60:path)
          n45 = Create Folder(path (use dialog)=w62) -> (error out=w64:errorcluster)  [unwired: 2 in, 2 out]
          n46 = Bundle("MAIL SETTINGS"=w54, "Auto Mail Send"=w50, "") -> (w53:T18)  [unwired: 1 in]
          n47 = call <vilib>:"Clear Errors.vi"("error in (no error)"=w64) -> ()  [unwired: 6 in, 1 out]
          n48 = Open/Create/Replace File(file path (use dialog)=w60) -> (refnum out=w58:refnum<file>, error out=w59:errorcluster)  [unwired: 5 in, 1 out]
          n49 = Read from Binary File(5:w53, 8:w59, 11:w58) -> (0:w56:errorcluster, 2:w52:T18, 3:w57:refnum<file>)  [unwired: 3 in, 1 out]
          n50 = Unbundle(w52) -> ("MAIL SETTINGS"=w51:T6, "Auto Mail Send"=w49:bool, w48:string)
          n51 = local write "TO (string):"(w48) -> ()
          n52 = local write "Auto Mail Send"(w49) -> ()
          n53 = local write "MAIL SETTINGS"(w51) -> ()
          n54 = Close File(refnum=w57, error in=w56) -> (error out=w55:errorcluster)  [unwired: 1 out]
          n55 = local write "data file error"(w55) -> ()
        }
        frame #4 {
          # "set display status if blank"
          n56 = local read "DISP LAB03-2"() -> (w94:T4)
          n57 = local read "DISP LAB03-1"() -> (w101:T4)
          n58 = local read "DISP LAB02-2"() -> (w108:T4)
          n59 = local read "DISP LAB01-2"() -> (w121:T4)
          n60 = local read "DISP LAB01-1"() -> (w130:T4)
          n61 = local read "DISP LAB02-1"() -> (w115:T4)
          n62 = Unbundle(w94) -> ("STATUS"=w96:string)  [unwired: 2 out]
          n63 = Unbundle(w101) -> ("STATUS"=w103:string)  [unwired: 2 out]
          n64 = Unbundle(w108) -> ("STATUS"=w110:string)  [unwired: 2 out]
          n65 = Unbundle(w115) -> ("STATUS"=w117:string)  [unwired: 2 out]
          n66 = Unbundle(w121) -> ("STATUS"=w124:string)  [unwired: 2 out]
          n67 = Unbundle(w130) -> ("STATUS"=w131:string)  [unwired: 2 out]
          n68 = Equal?(x="", y=w96) -> (x = y?=w98:bool)
          n69 = Equal?(x="", y=w103) -> (x = y?=w105:bool)
          n70 = Equal?(x="", y=w110) -> (x = y?=w112:bool)
          n71 = Equal?(x="", y=w117) -> (x = y?=w119:bool)
          n72 = Equal?(x="", y=w124) -> (x = y?=w126:bool)
          n73 = Equal?(x="", y=w131) -> (x = y?=w133:bool)
          n74 = Select(t="STOP", s=w98, f=w96) -> (s? t:f=w95:string)
          n75 = Select(t="STOP", s=w105, f=w103) -> (s? t:f=w102:string)
          n76 = Select(t="STOP", s=w112, f=w110) -> (s? t:f=w109:string)
          n77 = Select(t="STOP", s=w119, f=w117) -> (s? t:f=w116:string)
          n78 = Select(t="STOP", s=w126, f=w124) -> (s? t:f=w123:string)
          n79 = Select(t="STOP", s=w133, f=w131) -> (s? t:f=w129:string)
          n80 = Bundle(cluster=w94, "STATUS"=w95) -> (w93:T4)  [unwired: 2 in]
          n81 = Bundle(cluster=w101, "STATUS"=w102) -> (w100:T4)  [unwired: 2 in]
          n82 = Bundle(cluster=w108, "STATUS"=w109) -> (w107:T4)  [unwired: 2 in]
          n83 = Bundle(cluster=w115, "STATUS"=w116) -> (w114:T4)  [unwired: 2 in]
          n84 = Bundle(cluster=w121, "STATUS"=w123) -> (w122:T4)  [unwired: 2 in]
          n85 = Bundle(cluster=w130, "STATUS"=w129) -> (w128:T4)  [unwired: 2 in]
          n86 = local write "DISP LAB01-2"(w122) -> ()
          n87 = local write "DISP LAB01-1"(w128) -> ()
          n88 = local write "DISP LAB02-1"(w114) -> ()
          n89 = local write "DISP LAB03-1"(w100) -> ()
          n90 = local write "DISP LAB02-2"(w107) -> ()
          n91 = local write "DISP LAB03-2"(w93) -> ()
          n92 = local read "DISP LAB05-2"() -> (w66:T4)
          n93 = local read "DISP LAB05-1"() -> (w73:T4)
          n94 = local read "DISP LAB04-2"() -> (w75:T4)
          n95 = local read "DISP LAB04-1"() -> (w77:T4)
          n96 = Unbundle(w66) -> ("STATUS"=w68:string)  [unwired: 2 out]
          n97 = Unbundle(w73) -> ("STATUS"=w79:string)  [unwired: 2 out]
          n98 = Unbundle(w75) -> ("STATUS"=w84:string)  [unwired: 2 out]
          n99 = Unbundle(w77) -> ("STATUS"=w89:string)  [unwired: 2 out]
          n100 = Equal?(x="", y=w68) -> (x = y?=w70:bool)
          n101 = Equal?(x="", y=w79) -> (x = y?=w81:bool)
          n102 = Equal?(x="", y=w84) -> (x = y?=w86:bool)
          n103 = Equal?(x="", y=w89) -> (x = y?=w91:bool)
          n104 = Select(t="STOP", s=w70, f=w68) -> (s? t:f=w67:string)
          n105 = Select(t="STOP", s=w81, f=w79) -> (s? t:f=w78:string)
          n106 = Select(t="STOP", s=w86, f=w84) -> (s? t:f=w83:string)
          n107 = Select(t="STOP", s=w91, f=w89) -> (s? t:f=w88:string)
          n108 = Bundle(cluster=w66, "STATUS"=w67) -> (w65:T4)  [unwired: 2 in]
          n109 = Bundle(cluster=w73, "STATUS"=w78) -> (w72:T4)  [unwired: 2 in]
          n110 = Bundle(cluster=w75, "STATUS"=w83) -> (w74:T4)  [unwired: 2 in]
          n111 = Bundle(cluster=w77, "STATUS"=w88) -> (w76:T4)  [unwired: 2 in]
          n112 = local write "DISP LAB05-2"(w65) -> ()
          n113 = local write "DISP LAB05-1"(w72) -> ()
          n114 = local write "DISP LAB04-1"(w76) -> ()
          n115 = local write "DISP LAB04-2"(w74) -> ()
        }
        frame #5 {
          # "initialise analog input express vi's"
          n116 = for {
            N: 2.0 -> [_]
            n117 = call "sub vi - analog 1st setup v1.vi"() -> ()  [unwired: 11 in, 5 out]
          }
        }
        frame #6 {
          w136 = FALSE
          # "enable front panel, all settings done"
          n118 = property on="Tab Control 2" class="TabCtl (strict)"("DisabledEnum"=T11."Enabled" ("Disabled")) -> ()  [unwired: 2 in, 2 out]
          n119 = property on="Tab Control 2" class="TabCtl (strict)"() -> ("Pages"=w137:refnum<vi>[])  [unwired: 2 in, 2 out]
          n120 = Index Array(array=w137, index=6) -> (element=w139:refnum<vi>)
          n121 = local write "SHOW ADMIN PAGE"(w136) -> ()
          n122 = property class="Page"(reference=w139, "PageVis"=w136) -> ()  [unwired: 1 in, 2 out]
        }
      }
    }
    frame #2 {
      n123 = node-c288("loop  delay(mS)") -> (w143:T12)  [unwired: 3 in]
      n124 = timed-loop {
        timing: w143 -> [_]
        timing-out: [_] -> w142
        i -> [w165]
        stop <- "stop" stop-if-true
        n125 = node-c288() -> ()  [unwired: 1 in, 1 out]
        n126 = local read "SELECT LAB05-2"() -> (w145:T3)
        n127 = local read "SELECT LAB05-1"() -> (w146:T3)
        n128 = local read "SELECT LAB04-2"() -> (w147:T3)
        n129 = local read "SELECT LAB03-1"() -> (w150:T3)
        n130 = local read "SELECT LAB02-2"() -> (w151:T3)
        n131 = local read "SELECT LAB01-1"() -> (w154:T3)
        n132 = local read "SELECT LAB03-2"() -> (w149:T3)
        n133 = local read "SELECT LAB01-2"() -> (w153:T3)
        n134 = local read "SELECT LAB04-1"() -> (w148:T3)
        n135 = local read "SELECT LAB02-1"() -> (w152:T3)
        n136 = local read "run lab03-2"() -> (w159:bool)
        n137 = local read "run lab04-1"() -> (w158:bool)
        n138 = local read "run lab05-1"() -> (w156:bool)
        n139 = local read "run lab04-2"() -> (w157:bool)
        n140 = local read "run lab05-2"() -> (w155:bool)
        n141 = local read "run lab03-1"() -> (w160:bool)
        n142 = local read "run lab02-2"() -> (w161:bool)
        n143 = local read "run lab02-1"() -> (w162:bool)
        n144 = local read "run lab01-1"() -> (w164:bool)
        n145 = local read "run lab01-2"() -> (w163:bool)
        n146 = stacked-sequence {
          seq-local: [_ w227 _ _ _ _ _ _ _ _ _ _ _ _ _ _ _] -> [_ _ _ _ _ w1752 _ _ _ _ _ _ _ _ _ _ _]
          seq-local: [_ w226 _ _ _ _ _ _ _ _ _ _ _ _ _ _ _] -> [_ _ _ _ _ w1751 _ _ _ _ _ _ _ _ _ _ _]
          seq-local: [_ w213 _ _ _ _ _ _ _ _ _ _ _ _ _ _ _] -> [_ _ _ _ _ w1750 _ _ _ _ _ _ _ _ _ _ _]
          seq-local: [_ w212 _ _ _ _ _ _ _ _ _ _ _ _ _ _ _] -> [_ _ _ _ _ w1749 _ _ _ _ _ _ _ _ _ _ _]
          seq-local: [_ w211 _ _ _ _ _ _ _ _ _ _ _ _ _ _ _] -> [_ _ _ _ _ w1748 _ _ _ _ _ _ _ _ _ _ _]
          seq-local: [_ w210 _ _ _ _ _ _ _ _ _ _ _ _ _ _ _] -> [_ _ _ _ _ w1747 _ _ _ _ _ _ _ _ _ _ _]
          seq-local: [_ w209 _ _ _ _ _ _ _ _ _ _ _ _ _ _ _] -> [_ _ _ _ _ w1746 _ _ _ _ _ _ _ _ _ _ _]
          seq-local: [_ w208 _ _ _ _ _ _ _ _ _ _ _ _ _ _ _] -> [_ _ _ _ _ w1745 _ _ _ _ _ _ _ _ _ _ _]
          seq-local: [_ w207 _ _ _ _ _ _ _ _ _ _ _ _ _ _ _] -> [_ _ _ _ _ w1744 _ _ _ _ _ _ _ _ _ _ _]
          seq-local: [_ w206 _ _ _ _ _ _ _ _ _ _ _ _ _ _ _] -> [_ _ _ _ _ w1743 _ _ _ _ _ _ _ _ _ _ _]
          tunnel: w164 -> [_ _ w243 w408 w1352 w1772 w2082 w2327 _ _ _ _ w2772 w3260 _ _ w3535]
          tunnel: w163 -> [_ _ w242 w406 w1351 w1771 w2083 w2326 _ _ _ _ w2771 w3258 _ _ w3534]
          tunnel: w162 -> [_ _ w241 w404 w1350 w1770 w2081 w2325 _ _ _ _ w2770 w3256 _ _ w3533]
          tunnel: w161 -> [_ _ w240 w402 w1349 w1769 w2080 w2324 _ _ _ _ w2769 w3254 _ _ w3532]
          tunnel: w160 -> [_ _ w239 w400 w1348 w1768 w2079 w2323 _ _ _ _ w2768 w3252 _ _ w3531]
          tunnel: w159 -> [_ _ w238 w398 w1347 w1767 w2078 w2322 _ _ _ _ w2767 w3250 _ _ w3530]
          tunnel: w158 -> [_ _ w237 w396 w1346 w1766 w2077 w2321 _ _ _ _ w2766 w3248 _ _ w3529]
          tunnel: w157 -> [_ _ w236 w394 w1345 w1765 w2076 w2320 _ _ _ _ w2765 w3246 _ _ w3528]
          tunnel: w156 -> [_ _ w235 w392 w1344 w1764 w2075 w2319 _ _ _ _ w2764 w3244 _ _ w3527]
          tunnel: w155 -> [_ _ w234 w390 w1343 w1763 w2074 w2318 _ _ _ _ w2763 w3242 _ _ w3526]
          tunnel: w154 -> [_ _ _ w407 w1342 w1762 _ _ _ _ _ _ _ w3262 _ _ _]
          tunnel: w153 -> [_ _ _ w405 w1341 w1761 _ _ _ _ _ _ _ w3257 _ _ _]
          tunnel: w152 -> [_ _ _ w403 w1340 w1760 _ _ _ _ _ _ _ w3255 _ _ _]
          tunnel: w151 -> [_ _ _ w401 w1339 w1759 _ _ _ _ _ _ _ w3253 _ _ _]
          tunnel: w150 -> [_ _ _ w399 w1338 w1758 _ _ _ _ _ _ _ w3251 _ _ _]
          tunnel: w149 -> [_ _ _ w397 w1337 w1757 _ _ _ _ _ _ _ w3249 _ _ _]
          tunnel: w148 -> [_ _ _ w395 w1336 w1756 _ _ _ _ _ _ _ w3247 _ _ _]
          tunnel: w147 -> [_ _ _ w393 w1335 w1755 _ _ _ _ _ _ _ w3245 _ _ _]
          tunnel: w146 -> [_ _ _ w391 w1334 w1754 _ _ _ _ _ _ _ w3243 _ _ _]
          tunnel: w145 -> [_ _ _ w389 w1333 w1753 _ _ _ _ _ _ _ w3241 _ _ _]
          frame #0 {
            w169 = FALSE
            w174 = 0.5
            # "set up cycle control"
            n147 = local read "jig cycle"() -> (w173:dbl)
            n148 = Divide(x="JIG ON TIME (S)", y=w174) -> (x/y=→"on loops":dbl)
            n149 = Divide(x="JIG OFF TIME (S)", y=w174) -> (x/y=→"off loops":dbl)
            n150 = Increment(x=w173) -> (x+1=w172:dbl)
            n151 = local write "TEMP update"(w169) -> ()
            n152 = local write "AI update"(w169) -> ()
            n153 = local write "jig cycle"(w172) -> ()
            n154 = event shown="[1] \"SHOW ADMIN PAGE\": Value Change" {
              selector: _ -> [_ _]
              dyn-events: _ -> [_ _]
              timeout: 10 -> [_ _]
              event Timeout {
                n155 = event-data() -> ()  [unwired: 1 in, 3 out]
              }
              event "SHOW ADMIN PAGE": Value Change {
                n156 = event-data() -> ()  [unwired: 1 in, 6 out]
                n157 = stacked-sequence {
                  seq-local: [_ w178 _] -> [_ _ w179]
                  frame #0 {
                    n158 = global write "Global 1.vi" "password"("9999") -> ()
                  }
                  frame #1 {
                    n159 = call "sub vi - password 1.vi"() -> ("RESULT"=w178:bool)  [unwired: 11 in]
                  }
                  frame #2 {
                    w181 = FALSE
                    n160 = property on="Tab Control 2" class="TabCtl (strict)"() -> ("Pages"=w185:refnum<vi>[])  [unwired: 2 in, 2 out]
                    n161 = Select(t=TRUE, s=w179, f=w181) -> (s? t:f=w180:bool)
                    n162 = Index Array(array=w185, index=6) -> (element=w183:refnum<vi>)
                    n163 = local write "SHOW ADMIN PAGE"(w181) -> ()
                    n164 = property class="Page"(reference=w183, "PageVis"=w180) -> ()  [unwired: 1 in, 2 out]
                  }
                }
              }
            }
          }
          frame #1 {
            w223 = 60.0
            # "convert temperature rise minutes to cycles"
            n165 = local read "SET LAB05-2"() -> (w187:T5)
            n166 = local read "SET LAB05-1"() -> (w189:T5)
            n167 = local read "SET LAB04-2"() -> (w191:T5)
            n168 = local read "SET LAB01-1"() -> (w205:T5)
            n169 = local read "SET LAB01-2"() -> (w203:T5)
            n170 = local read "SET LAB02-2"() -> (w199:T5)
            n171 = local read "SET LAB04-1"() -> (w193:T5)
            n172 = local read "SET LAB03-1"() -> (w197:T5)
            n173 = local read "SET LAB03-2"() -> (w195:T5)
            n174 = local read "SET LAB02-1"() -> (w201:T5)
            n175 = local read "JIG OFF TIME (S)"() -> (w228:dbl)
            n176 = local read "JIG ON TIME (S)"() -> (w229:dbl)
            n177 = Unbundle(w187) -> ("T-RISE mins"=w186:dbl)  [unwired: 4 out]
            n178 = Unbundle(w189) -> ("T-RISE mins"=w188:dbl)  [unwired: 4 out]
            n179 = Unbundle(w205) -> ("T-RISE mins"=w204:dbl)  [unwired: 4 out]
            n180 = Unbundle(w191) -> ("T-RISE mins"=w190:dbl)  [unwired: 4 out]
            n181 = Unbundle(w203) -> ("T-RISE mins"=w202:dbl)  [unwired: 4 out]
            n182 = Unbundle(w201) -> ("T-RISE mins"=w200:dbl)  [unwired: 4 out]
            n183 = Unbundle(w193) -> ("T-RISE mins"=w192:dbl)  [unwired: 4 out]
            n184 = Unbundle(w199) -> ("T-RISE mins"=w198:dbl)  [unwired: 4 out]
            n185 = Unbundle(w195) -> ("T-RISE mins"=w194:dbl)  [unwired: 4 out]
            n186 = Unbundle(w197) -> ("T-RISE mins"=w196:dbl)  [unwired: 4 out]
            n187 = Add(x=w229, y=w228) -> (x+y=w222:dbl)
            n188 = Multiply(x=w223, y=w194) -> (x*y=w218:dbl)
            n189 = Multiply(x=w223, y=w192) -> (x*y=w217:dbl)
            n190 = Multiply(x=w223, y=w190) -> (x*y=w216:dbl)
            n191 = Multiply(x=w223, y=w188) -> (x*y=w215:dbl)
            n192 = Multiply(x=w223, y=w186) -> (x*y=w214:dbl)
            n193 = Multiply(x=w223, y=w202) -> (x*y=w224:dbl)
            n194 = Multiply(x=w223, y=w196) -> (x*y=w219:dbl)
            n195 = Multiply(x=w223, y=w204) -> (x*y=w225:dbl)
            n196 = Multiply(x=w223, y=w200) -> (x*y=w221:dbl)
            n197 = Multiply(x=w223, y=w198) -> (x*y=w220:dbl)
            n198 = Divide(x=w215, y=w222) -> (x/y=w207:dbl)
            n199 = Divide(x=w216, y=w222) -> (x/y=w208:dbl)
            n200 = Divide(x=w217, y=w222) -> (x/y=w209:dbl)
            n201 = Divide(x=w214, y=w222) -> (x/y=w206:dbl)
            n202 = Divide(x=w219, y=w222) -> (x/y=w211:dbl)
            n203 = Divide(x=w225, y=w222) -> (x/y=w227:dbl)
            n204 = Divide(x=w224, y=w222) -> (x/y=w226:dbl)
            n205 = Divide(x=w221, y=w222) -> (x/y=w213:dbl)
            n206 = Divide(x=w220, y=w222) -> (x/y=w212:dbl)
            n207 = Divide(x=w218, y=w222) -> (x/y=w210:dbl)
          }
          frame #2 {
            # "control cycle loops"
            n208 = local read "JIG OFF TIME (S)"() -> (w232:dbl)
            n209 = local read "JIG ON TIME (S)"() -> (w231:dbl)
            n210 = local read "jig cycle"() -> (w245:dbl)
            n211 = local read "on loops"() -> (w247:dbl)
            n212 = local read "off loops"() -> (w246:dbl)
            n213 = Add(x=w232, y=w231) -> (x+y=w230:dbl)
            n214 = Add(x=w247, y=w246) -> (x+y=w233:dbl)
            n215 = Greater Or Equal?(x=w245, y=w233) -> (x >= y?=w244:bool)
            n216 = case shown="True" w244 {
              tunnel: w243 -> [_ w258]
              tunnel: w242 -> [_ w257]
              tunnel: w241 -> [_ w256]
              tunnel: w240 -> [_ w255]
              tunnel: w239 -> [_ w254]
              tunnel: w238 -> [_ w253]
              tunnel: w237 -> [_ w252]
              tunnel: w236 -> [_ w251]
              tunnel: w235 -> [_ w250]
              tunnel: w234 -> [_ w249]
              tunnel: w230 -> [_ w248]
              frame False {
              }
              frame True {
                # "increment cycle value and convert cycles to minutes for temp rise"
                n217 = stacked-sequence {
                  tunnel: w258 -> [w268 _ _ _ _ _ _ _ _ _]
                  tunnel: w257 -> [_ w280 _ _ _ _ _ _ _ _]
                  tunnel: w256 -> [_ _ w292 _ _ _ _ _ _ _]
                  tunnel: w255 -> [_ _ _ w304 _ _ _ _ _ _]
                  tunnel: w254 -> [_ _ _ _ w316 _ _ _ _ _]
                  tunnel: w253 -> [_ _ _ _ _ w328 _ _ _ _]
                  tunnel: w252 -> [_ _ _ _ _ _ w340 _ _ _]
                  tunnel: w251 -> [_ _ _ _ _ _ _ w352 _ _]
                  tunnel: w250 -> [_ _ _ _ _ _ _ _ w364 _]
                  tunnel: w249 -> [_ _ _ _ _ _ _ _ _ w376]
                  tunnel: w248 -> [w265 w277 w289 w301 w313 w325 w337 w349 w361 w373]
                  frame #0 {
                    # "LAB01-1"
                    n218 = local read "DISP LAB01-1"() -> (w263:T4)
                    n219 = Unbundle(w263) -> ("CYCLE"=w264:dbl)  [unwired: 2 out]
                    n220 = case shown="True" w268 {
                      tunnel: w264 -> [w269 w271]
                      tunnel: [w269 w270] -> w262
                      frame False {
                      }
                      frame True {
                        n221 = Increment(x=w271) -> (x+1=w270:dbl)
                      }
                    }
                    n222 = Multiply(x=w262, y=w265) -> (x*y=w266:dbl)
                    n223 = Divide(x=w266, y=60.0) -> (x/y=w261:dbl)
                    n224 = Bundle(cluster=w263, "CYCLE"=w262, "MINS"=w261) -> (w260:T4)  [unwired: 1 in]
                    n225 = local write "DISP LAB01-1"(w260) -> ()
                  }
                  frame #1 {
                    # "update cycle value"
                    # "LAB01-2"
                    n226 = local read "DISP LAB01-2"() -> (w275:T4)
                    n227 = Unbundle(w275) -> ("CYCLE"=w276:dbl)  [unwired: 2 out]
                    n228 = case shown="True" w280 {
                      tunnel: w276 -> [w281 w283]
                      tunnel: [w281 w282] -> w273
                      frame False {
                      }
                      frame True {
                        n229 = Increment(x=w283) -> (x+1=w282:dbl)
                      }
                    }
                    n230 = Multiply(x=w273, y=w277) -> (x*y=w278:dbl)
                    n231 = Divide(x=w278, y=60.0) -> (x/y=w272:dbl)
                    n232 = Bundle(cluster=w275, "CYCLE"=w273, "MINS"=w272) -> (w274:T4)  [unwired: 1 in]
                    n233 = local write "DISP LAB01-2"(w274) -> ()
                  }
                  frame #2 {
                    # "update cycle value"
                    # "LAB02-1"
                    n234 = local read "DISP LAB02-1"() -> (w287:T4)
                    n235 = Unbundle(w287) -> ("CYCLE"=w288:dbl)  [unwired: 2 out]
                    n236 = case shown="True" w292 {
                      tunnel: [w293 w295] -> w285
                      tunnel: w288 -> [w293 w294]
                      frame False {
                      }
                      frame True {
                        n237 = Increment(x=w294) -> (x+1=w295:dbl)
                      }
                    }
                    n238 = Multiply(x=w285, y=w289) -> (x*y=w290:dbl)
                    n239 = Divide(x=w290, y=60.0) -> (x/y=w284:dbl)
                    n240 = Bundle(cluster=w287, "CYCLE"=w285, "MINS"=w284) -> (w286:T4)  [unwired: 1 in]
                    n241 = local write "DISP LAB02-1"(w286) -> ()
                  }
                  frame #3 {
                    # "update cycle value"
                    # "LAB02-2"
                    n242 = local read "DISP LAB02-2"() -> (w299:T4)
                    n243 = Unbundle(w299) -> ("CYCLE"=w300:dbl)  [unwired: 2 out]
                    n244 = case shown="True" w304 {
                      tunnel: [w305 w307] -> w298
                      tunnel: w300 -> [w305 w306]
                      frame False {
                      }
                      frame True {
                        n245 = Increment(x=w306) -> (x+1=w307:dbl)
                      }
                    }
                    n246 = Multiply(x=w298, y=w301) -> (x*y=w302:dbl)
                    n247 = Divide(x=w302, y=60.0) -> (x/y=w297:dbl)
                    n248 = Bundle(cluster=w299, "CYCLE"=w298, "MINS"=w297) -> (w296:T4)  [unwired: 1 in]
                    n249 = local write "DISP LAB02-2"(w296) -> ()
                  }
                  frame #4 {
                    # "update cycle value"
                    # "LAB03-1"
                    n250 = local read "DISP LAB03-1"() -> (w311:T4)
                    n251 = Unbundle(w311) -> ("CYCLE"=w312:dbl)  [unwired: 2 out]
                    n252 = case shown="True" w316 {
                      tunnel: [w317 w319] -> w308
                      tunnel: w312 -> [w317 w318]
                      frame False {
                      }
                      frame True {
                        n253 = Increment(x=w318) -> (x+1=w319:dbl)
                      }
                    }
                    n254 = Multiply(x=w308, y=w313) -> (x*y=w314:dbl)
                    n255 = Divide(x=w314, y=60.0) -> (x/y=w309:dbl)
                    n256 = Bundle(cluster=w311, "CYCLE"=w308, "MINS"=w309) -> (w310:T4)  [unwired: 1 in]
                    n257 = local write "DISP LAB03-1"(w310) -> ()
                  }
                  frame #5 {
                    # "update cycle value"
                    # "LAB03-2"
                    n258 = local read "DISP LAB03-2"() -> (w323:T4)
                    n259 = Unbundle(w323) -> ("CYCLE"=w324:dbl)  [unwired: 2 out]
                    n260 = case shown="False" w328 {
                      tunnel: [w329 w331] -> w322
                      tunnel: w324 -> [w329 w330]
                      frame False {
                      }
                      frame True {
                        n261 = Increment(x=w330) -> (x+1=w331:dbl)
                      }
                    }
                    n262 = Multiply(x=w322, y=w325) -> (x*y=w326:dbl)
                    n263 = Divide(x=w326, y=60.0) -> (x/y=w321:dbl)
                    n264 = Bundle(cluster=w323, "CYCLE"=w322, "MINS"=w321) -> (w320:T4)  [unwired: 1 in]
                    n265 = local write "DISP LAB03-2"(w320) -> ()
                  }
                  frame #6 {
                    # "update cycle value"
                    # "LAB04-1"
                    n266 = local read "DISP LAB04-1"() -> (w335:T4)
                    n267 = Unbundle(w335) -> ("CYCLE"=w336:dbl)  [unwired: 2 out]
                    n268 = case shown="True" w340 {
                      tunnel: [w341 w343] -> w333
                      tunnel: w336 -> [w341 w342]
                      frame False {
                      }
                      frame True {
                        n269 = Increment(x=w342) -> (x+1=w343:dbl)
                      }
                    }
                    n270 = Multiply(x=w333, y=w337) -> (x*y=w338:dbl)
                    n271 = Divide(x=w338, y=60.0) -> (x/y=w332:dbl)
                    n272 = Bundle(cluster=w335, "CYCLE"=w333, "MINS"=w332) -> (w334:T4)  [unwired: 1 in]
                    n273 = local write "DISP LAB04-1"(w334) -> ()
                  }
                  frame #7 {
                    # "update cycle value"
                    # "LAB04-2"
                    n274 = local read "DISP LAB04-2"() -> (w347:T4)
                    n275 = Unbundle(w347) -> ("CYCLE"=w348:dbl)  [unwired: 2 out]
                    n276 = case shown="True" w352 {
                      tunnel: [w353 w355] -> w345
                      tunnel: w348 -> [w353 w354]
                      frame False {
                      }
                      frame True {
                        n277 = Increment(x=w354) -> (x+1=w355:dbl)
                      }
                    }
                    n278 = Multiply(x=w345, y=w349) -> (x*y=w351:dbl)
                    n279 = Divide(x=w351, y=60.0) -> (x/y=w344:dbl)
                    n280 = Bundle(cluster=w347, "CYCLE"=w345, "MINS"=w344) -> (w346:T4)  [unwired: 1 in]
                    n281 = local write "DISP LAB04-2"(w346) -> ()
                  }
                  frame #8 {
                    # "update cycle value"
                    # "LAB05-1"
                    n282 = local read "DISP LAB05-1"() -> (w359:T4)
                    n283 = Unbundle(w359) -> ("CYCLE"=w360:dbl)  [unwired: 2 out]
                    n284 = case shown="True" w364 {
                      tunnel: [w365 w367] -> w357
                      tunnel: w360 -> [w365 w366]
                      frame False {
                      }
                      frame True {
                        n285 = Increment(x=w366) -> (x+1=w367:dbl)
                      }
                    }
                    n286 = Multiply(x=w357, y=w361) -> (x*y=w362:dbl)
                    n287 = Divide(x=w362, y=60.0) -> (x/y=w356:dbl)
                    n288 = Bundle(cluster=w359, "CYCLE"=w357, "MINS"=w356) -> (w358:T4)  [unwired: 1 in]
                    n289 = local write "DISP LAB05-1"(w358) -> ()
                  }
                  frame #9 {
                    # "update cycle value"
                    # "LAB05-2"
                    n290 = local read "DISP LAB05-2"() -> (w372:T4)
                    n291 = Unbundle(w372) -> ("CYCLE"=w371:dbl)  [unwired: 2 out]
                    n292 = case shown="True" w376 {
                      tunnel: [w377 w379] -> w370
                      tunnel: w371 -> [w377 w378]
                      frame False {
                      }
                      frame True {
                        n293 = Increment(x=w378) -> (x+1=w379:dbl)
                      }
                    }
                    n294 = Multiply(x=w370, y=w373) -> (x*y=w374:dbl)
                    n295 = Divide(x=w374, y=60.0) -> (x/y=w369:dbl)
                    n296 = Bundle(cluster=w372, "CYCLE"=w370, "MINS"=w369) -> (w368:T4)  [unwired: 1 in]
                    n297 = local write "DISP LAB05-2"(w368) -> ()
                  }
                }
                n298 = local write "jig cycle"(0) -> ()
              }
            }
          }
          frame #3 {
            (unwired) "c:\\BAT\\labdatav2\\"
            # "START & STOP test RUN switch change, start test if true and stop test if false"
            n299 = Get Date/Time In Seconds() -> (seconds since 1Jan1904=w387:timestamp)
            n300 = local read "C drive data root dir"() -> (w380:path)
            n301 = Format Date/Time String(time format string (%c)="%b%d", seconds (now)=w387) -> (date/time string=w411:string)  [unwired: 1 in]
            n302 = Format Date/Time String(time format string (%c)="%H%M", seconds (now)=w387) -> (date/time string=w409:string)  [unwired: 1 in]
            n303 = Format Date/Time String(time format string (%c)="%Y", seconds (now)=w387) -> (date/time string=w386:string)  [unwired: 1 in]
            n304 = Path To String(path=w380) -> (string=w383:string)
            n305 = global write "Global 1.vi" "C drive root path"(w380) -> ()
            n306 = Concatenate Strings(w383, "\\") -> (w381:string)
            n307 = event shown="[1] \"RUN LAB01-1\": Value Change" {
              selector: _ -> [_ _ _ _ _ _ _ _ _ _ _]
              dyn-events: _ -> [_ _ _ _ _ _ _ _ _ _ _]
              timeout: 10 -> [_ _ _ _ _ _ _ _ _ _ _]
              tunnel: w381 -> [_ w419 w511 w603 w695 w787 w879 w971 w1063 w1155 w1247]
              tunnel: w411 -> [_ w418 w510 w602 w694 w786 w878 w970 w1062 w1154 w1246]
              tunnel: w409 -> [_ w416 w509 w601 w693 w785 w877 w969 w1061 w1153 w1245]
              tunnel: w407 -> [_ w417 _ _ _ _ _ _ _ _ _]
              tunnel: w408 -> [_ _ _ _ _ _ _ _ _ _ _]
              tunnel: w406 -> [_ _ _ _ _ _ _ _ _ _ _]
              tunnel: w405 -> [_ _ w508 _ _ _ _ _ _ _ _]
              tunnel: w404 -> [_ _ _ _ _ _ _ _ _ _ _]
              tunnel: w403 -> [_ _ _ w600 _ _ _ _ _ _ _]
              tunnel: w402 -> [_ _ _ _ _ _ _ _ _ _ _]
              tunnel: w401 -> [_ _ _ _ w692 _ _ _ _ _ _]
              tunnel: w400 -> [_ _ _ _ _ _ _ _ _ _ _]
              tunnel: w399 -> [_ _ _ _ _ w784 _ _ _ _ _]
              tunnel: w398 -> [_ _ _ _ _ _ _ _ _ _ _]
              tunnel: w397 -> [_ _ _ _ _ _ w876 _ _ _ _]
              tunnel: w396 -> [_ _ _ _ _ _ _ _ _ _ _]
              tunnel: w395 -> [_ _ _ _ _ _ _ w968 _ _ _]
              tunnel: w394 -> [_ _ _ _ _ _ _ _ _ _ _]
              tunnel: w393 -> [_ _ _ _ _ _ _ _ w1060 _ _]
              tunnel: w392 -> [_ _ _ _ _ _ _ _ _ _ _]
              tunnel: w391 -> [_ _ _ _ _ _ _ _ _ w1152 _]
              tunnel: w390 -> [_ _ _ _ _ _ _ _ _ _ _]
              tunnel: w389 -> [_ _ _ _ _ _ _ _ _ _ w1244]
              tunnel: w386 -> [_ w415 w507 w599 w691 w783 w875 w967 w1059 w1151 w1243]
              tunnel: [_ w414 w506 w598 w690 w782 w874 w966 w1058 w1150 w1242] -> w384
              event Timeout {
                n308 = event-data() -> ()  [unwired: 1 in, 3 out]
              }
              event "RUN LAB01-1": Value Change {
                n309 = event-data() -> ("NewVal"=w413:bool)  [unwired: 1 in, 5 out]
                n310 = local write "run lab01-1"(w413) -> ()
                n311 = case shown="False" w413 {
                  tunnel: w419 -> [_ w452]
                  tunnel: w418 -> [_ w451]
                  tunnel: w417 -> [w421 w450]
                  tunnel: w416 -> [_ w449]
                  tunnel: w415 -> [_ w448]
                  tunnel: [w420 w447] -> w414
                  frame False {
                    # "stop test"
                    n312 = stacked-sequence {
                      tunnel: w421 -> [_ w433 _ _]
                      tunnel: [_ w425 _ _] -> w420
                      frame #0 {
                        n313 = local read "DISP LAB01-1"() -> (w424:T4)
                        n314 = Bundle(cluster=w424, "STATUS"="STOP") -> (w422:T4)  [unwired: 2 in]
                        n315 = local write "DISP LAB01-1"(w422) -> ()
                      }
                      frame #1 {
                        n316 = local read "DISP LAB01-1"() -> (w432:T4)
                        n317 = Unbundle(w432) -> ("CYCLE"=w430:dbl, "MINS"=w431:dbl)  [unwired: 1 out]
                        n318 = case shown="\"CYCLE TEST\"" w433 {
                          tunnel: w431 -> [_ _ w440]
                          tunnel: w430 -> [w438 w439 _]
                          tunnel: [w438 w439 w440] -> w429
                          frame "CHART TEST", Default {
                          }
                          frame "CYCLE TEST" {
                          }
                          frame "T-RISE TEST" {
                          }
                        }
                        n319 = local read "TDMS LAB01-1"() -> (w437:refnum<k34>)
                        n320 = Build Array("STOPPED") -> (w434:string[])
                        n321 = Build Array(w429) -> (w428:dbl[])
                        n322 = TDMS Write(0:w437, 5:"TEST RESULT", 7:w434, 9:w428) -> (4:w426:refnum<k34>, 15:w427:errorcluster)  [unwired: 2 in, 2 out]
                        n323 = TDMS Close(8:w427, 11:w426) -> (0:w425:errorcluster)  [unwired: 1 out]
                      }
                      frame #2 {
                        n324 = stacked-sequence {
                          tunnel: "LAB01-1" -> [w443 w446]
                          frame #0 {
                            n325 = call "Save data file to network drive v1.vi"("panel id"=w443) -> ("network file save error"=w442:errorcluster)  [unwired: 9 in, 1 out]
                            n326 = local write "RESULT LAB01-1"(FALSE) -> ()
                            n327 = local write "data file error"(w442) -> ()
                          }
                          frame #1 {
                            n328 = call "sub vi - defrag tdms v1.vi"("panel id"=w446) -> ("error out"=w445:errorcluster)  [unwired: 10 in]
                            n329 = local write "data file error"(w445) -> ()
                          }
                        }
                      }
                      frame #3 {
                      }
                    }
                  }
                  frame True {
                    # "start new test and create test file"
                    n330 = stacked-sequence {
                      seq-local: [w453 _ _ _ _] -> [_ w474 _ _ _]
                      tunnel: w452 -> [w458 _ _ _ _]
                      tunnel: w451 -> [w454 _ _ _ _]
                      tunnel: w450 -> [w468 _ _ _ _]
                      tunnel: w449 -> [w461 _ _ _ _]
                      tunnel: w448 -> [w456 _ _ _ _]
                      tunnel: [_ w475 _ _ _] -> w447
                      frame #0 {
                        w455 = "\\"
                        n331 = local read "SET LAB01-1"() -> (w463:T5)
                        n332 = case shown="\"CHART TEST\", Default" w468 {
                          tunnel: ["CHART TEST-" "CYCLE TEST-" "T-RISE TEST-"] -> w464
                          frame "CHART TEST", Default {
                          }
                          frame "CYCLE TEST" {
                          }
                          frame "T-RISE TEST" {
                          }
                        }
                        n333 = Unbundle(w463) -> ("DESCRIPTION"=w462:string)  [unwired: 4 out]
                        n334 = Concatenate Strings(w458, "LAB01-1\\", w456, w455, w454, w455) -> (w465:string)
                        n335 = String To Path(string=w465) -> (path=w467:path)
                        n336 = Concatenate Strings(w465, w464, w462, "-", w461, ".tdms") -> (w453:string)
                        n337 = Create Folder(path (use dialog)=w467) -> (error out=w466:errorcluster)  [unwired: 2 in, 2 out]
                        n338 = call <vilib>:"Clear Errors.vi"("error in (no error)"=w466) -> ()  [unwired: 6 in, 1 out]
                        n339 = global write "Global 1.vi" "LAB01-1 FILE"(w453) -> ()
                      }
                      frame #1 {
                        n340 = String To Path(string=w474) -> (path=w472:path)
                        n341 = TDMS Open(5:FALSE, 6:FALSE, 10:T15."create or replace" ("operation (0:open)"), 11:w472) -> (0:w475:errorcluster, 3:→"TDMS LAB01-1":refnum<k34>)  [unwired: 3 in]
                      }
                      frame #2 {
                        n342 = local read "SET LAB01-1"() -> (w484:T5)
                        n343 = local read "TDMS LAB01-1"() -> (w495:refnum<k34>)
                        n344 = Build Array("Testers Name", "Description", "Set Test Cycles", "T-Rise minutes", "T-Rise Deg C") -> (w485:string[])
                        n345 = Unbundle(w484) -> ("NAME"=w483:string, "DESCRIPTION"=w482:string, "CYCLES"=w481:dbl, "T-RISE mins"=w480:dbl, "T-RISE deg C"=w479:dbl)
                        n346 = Number To Decimal String(number=w481) -> (decimal integer string=w494:string)  [unwired: 1 in]
                        n347 = Number To Decimal String(number=w480) -> (decimal integer string=w493:string)  [unwired: 1 in]
                        n348 = Number To Decimal String(number=w479) -> (decimal integer string=w492:string)  [unwired: 1 in]
                        n349 = Build Array(w483, w482, w494, w493, w492) -> (w491:string[])
                        n350 = TDMS Set Properties(5:w491, 7:w485, 11:w495) -> ()  [unwired: 3 in, 4 out]
                      }
                      frame #3 {
                        w496 = 0.0
                        n351 = local read "DISP LAB01-1"() -> (w499:T4)
                        n352 = Bundle(cluster=w499, "CYCLE"=w496, "MINS"=w496, "STATUS"="RUN") -> (w498:T4)
                        n353 = local write "DISP LAB01-1"(w498) -> ()
                      }
                      frame #4 {
                        n354 = local read "SIG LAB01-1"() -> (w502:T2)
                        n355 = local read "TEMP START LAB01-1"() -> (w504:cluster{"TL":dbl, "TN":dbl})
                        n356 = Unbundle(w502) -> ("Tmp Live"=w501:dbl, "Tmp Neut"=w500:dbl)  [unwired: 3 out]
                        n357 = Bundle(cluster=w504, "TL"=w501, "TN"=w500) -> (w503:cluster{"TL":dbl, "TN":dbl})
                        n358 = local write "TEMP START LAB01-1"(w503) -> ()
                      }
                    }
                  }
                }
              }
              event "RUN LAB01-2": Value Change {
                n359 = event-data() -> ("NewVal"=w505:bool)  [unwired: 1 in, 5 out]
                n360 = local write "run lab01-2"(w505) -> ()
                n361 = case shown="False" w505 {
                  tunnel: w511 -> [_ w544]
                  tunnel: w510 -> [_ w543]
                  tunnel: w508 -> [w513 w542]
                  tunnel: w509 -> [_ w541]
                  tunnel: w507 -> [_ w540]
                  tunnel: [w512 w539] -> w506
                  frame False {
                    # "stop test"
                    n362 = stacked-sequence {
                      tunnel: w513 -> [w522 _]
                      tunnel: [w514 _] -> w512
                      frame #0 {
                        n363 = local read "DISP LAB01-2"() -> (w521:T4)
                        n364 = Unbundle(w521) -> ("CYCLE"=w519:dbl, "MINS"=w520:dbl)  [unwired: 1 out]
                        n365 = case shown="\"CHART TEST\", Default" w522 {
                          tunnel: w520 -> [_ _ w529]
                          tunnel: w519 -> [w527 w528 _]
                          tunnel: [w527 w528 w529] -> w518
                          frame "CHART TEST", Default {
                          }
                          frame "CYCLE TEST" {
                          }
                          frame "T-RISE TEST" {
                          }
                        }
                        n366 = local read "TDMS LAB01-2"() -> (w526:refnum<k34>)
                        n367 = Build Array("STOPPED") -> (w523:string[])
                        n368 = Build Array(w518) -> (w517:dbl[])
                        n369 = TDMS Write(0:w526, 5:"TEST RESULT", 7:w523, 9:w517) -> (4:w515:refnum<k34>, 15:w516:errorcluster)  [unwired: 2 in, 2 out]
                        n370 = TDMS Close(8:w516, 11:w515) -> (0:w514:errorcluster)  [unwired: 1 out]
                      }
                      frame #1 {
                        n371 = local read "DISP LAB01-2"() -> (w533:T4)
                        n372 = stacked-sequence {
                          tunnel: "LAB01-2" -> [w535 w538]
                          frame #0 {
                            n373 = call "Save data file to network drive v1.vi"("panel id"=w535) -> ("network file save error"=w534:errorcluster)  [unwired: 9 in, 1 out]
                            n374 = local write "RESULT LAB01-2"(FALSE) -> ()
                            n375 = local write "data file error"(w534) -> ()
                          }
                          frame #1 {
                            n376 = call "sub vi - defrag tdms v1.vi"("panel id"=w538) -> ("error out"=w537:errorcluster)  [unwired: 10 in]
                            n377 = local write "data file error"(w537) -> ()
                          }
                        }
                        n378 = Bundle(cluster=w533, "STATUS"="STOP") -> (w531:T4)  [unwired: 2 in]
                        n379 = local write "DISP LAB01-2"(w531) -> ()
                      }
                    }
                  }
                  frame True {
                    # "start new test and create test file"
                    n380 = stacked-sequence {
                      seq-local: [w545 _ _ _ _] -> [_ w570 _ _ _]
                      tunnel: w544 -> [w550 _ _ _ _]
                      tunnel: w543 -> [w547 _ _ _ _]
                      tunnel: w542 -> [w560 _ _ _ _]
                      tunnel: w541 -> [w553 _ _ _ _]
                      tunnel: w540 -> [w548 _ _ _ _]
                      tunnel: [_ w564 _ _ _] -> w539
                      frame #0 {
                        w546 = "\\"
                        n381 = local read "SET LAB01-2"() -> (w555:T5)
                        n382 = case shown="\"CHART TEST\", Default" w560 {
                          tunnel: ["CHART TEST-" "CYCLE TEST-" "T-RISE TEST-"] -> w556
                          frame "CHART TEST", Default {
                          }
                          frame "CYCLE TEST" {
                          }
                          frame "T-RISE TEST" {
                          }
                        }
                        n383 = Unbundle(w555) -> ("DESCRIPTION"=w554:string)  [unwired: 4 out]
                        n384 = Concatenate Strings(w550, "LAB01-2\\", w548, w546, w547, w546) -> (w557:string)
                        n385 = String To Path(string=w557) -> (path=w559:path)
                        n386 = Concatenate Strings(w557, w556, w554, "-", w553, ".tdms") -> (w545:string)
                        n387 = Create Folder(path (use dialog)=w559) -> (error out=w558:errorcluster)  [unwired: 2 in, 2 out]
                        n388 = global write "Global 1.vi" "LAB01-2 FILE"(w545) -> ()
                        n389 = call <vilib>:"Clear Errors.vi"("error in (no error)"=w558) -> ()  [unwired: 6 in, 1 out]
                      }
                      frame #1 {
                        n390 = String To Path(string=w570) -> (path=w565:path)
                        n391 = TDMS Open(5:FALSE, 6:FALSE, 10:T15."create or replace" ("operation (0:open)"), 11:w565) -> (0:w564:errorcluster, 3:→"TDMS LAB01-2":refnum<k34>)  [unwired: 3 in]
                      }
                      frame #2 {
                        n392 = local read "SET LAB01-2"() -> (w576:T5)
                        n393 = local read "TDMS LAB01-2"() -> (w587:refnum<k34>)
                        n394 = Build Array("Testers Name", "Description", "Set Test Cycles", "T-Rise minutes", "T-Rise Deg C") -> (w577:string[])
                        n395 = Unbundle(w576) -> ("NAME"=w575:string, "DESCRIPTION"=w574:string, "CYCLES"=w573:dbl, "T-RISE mins"=w572:dbl, "T-RISE deg C"=w571:dbl)
                        n396 = Number To Decimal String(number=w573) -> (decimal integer string=w586:string)  [unwired: 1 in]
                        n397 = Number To Decimal String(number=w572) -> (decimal integer string=w585:string)  [unwired: 1 in]
                        n398 = Number To Decimal String(number=w571) -> (decimal integer string=w584:string)  [unwired: 1 in]
                        n399 = Build Array(w575, w574, w586, w585, w584) -> (w583:string[])
                        n400 = TDMS Set Properties(5:w583, 7:w577, 11:w587) -> ()  [unwired: 3 in, 4 out]
                      }
                      frame #3 {
                        w589 = 0.0
                        n401 = local read "DISP LAB01-2"() -> (w591:T4)
                        n402 = Bundle(cluster=w591, "CYCLE"=w589, "MINS"=w589, "STATUS"="RUN") -> (w590:T4)
                        n403 = local write "DISP LAB01-2"(w590) -> ()
                      }
                      frame #4 {
                        n404 = local read "SIG LAB01-2"() -> (w594:T2)
                        n405 = local read "TEMP START LAB01-2"() -> (w596:cluster{"TL":dbl, "TN":dbl})
                        n406 = Unbundle(w594) -> ("Tmp Live"=w593:dbl, "Tmp Neut"=w592:dbl)  [unwired: 3 out]
                        n407 = Bundle(cluster=w596, "TL"=w593, "TN"=w592) -> (w595:cluster{"TL":dbl, "TN":dbl})
                        n408 = local write "TEMP START LAB01-2"(w595) -> ()
                      }
                    }
                  }
                }
              }
              event "RUN LAB02-1": Value Change {
                n409 = event-data() -> ("NewVal"=w597:bool)  [unwired: 1 in, 5 out]
                n410 = local write "run lab02-1"(w597) -> ()
                n411 = case shown="False" w597 {
                  tunnel: w603 -> [_ w636]
                  tunnel: w602 -> [_ w635]
                  tunnel: w600 -> [w605 w634]
                  tunnel: w601 -> [_ w633]
                  tunnel: w599 -> [_ w632]
                  tunnel: [w604 w631] -> w598
                  frame False {
                    # "stop test"
                    n412 = stacked-sequence {
                      tunnel: w605 -> [w614 _]
                      tunnel: [w606 _] -> w604
                      frame #0 {
                        n413 = local read "DISP LAB02-1"() -> (w613:T4)
                        n414 = Unbundle(w613) -> ("CYCLE"=w611:dbl, "MINS"=w612:dbl)  [unwired: 1 out]
                        n415 = case shown="\"CYCLE TEST\"" w614 {
                          tunnel: w612 -> [_ _ w621]
                          tunnel: w611 -> [w619 w620 _]
                          tunnel: [w619 w620 w621] -> w610
                          frame "CHART TEST", Default {
                          }
                          frame "CYCLE TEST" {
                          }
                          frame "T-RISE TEST" {
                          }
                        }
                        n416 = local read "TDMS LAB02-1"() -> (w618:refnum<k34>)
                        n417 = Build Array("STOPPED") -> (w615:string[])
                        n418 = Build Array(w610) -> (w609:dbl[])
                        n419 = TDMS Write(0:w618, 5:"TEST RESULT", 7:w615, 9:w609) -> (4:w607:refnum<k34>, 15:w608:errorcluster)  [unwired: 2 in, 2 out]
                        n420 = TDMS Close(8:w608, 11:w607) -> (0:w606:errorcluster)  [unwired: 1 out]
                      }
                      frame #1 {
                        n421 = local read "DISP LAB02-1"() -> (w625:T4)
                        n422 = stacked-sequence {
                          tunnel: "LAB02-1" -> [w627 w629]
                          frame #0 {
                            n423 = call "sub vi - defrag tdms v1.vi"("panel id"=w627) -> ("error out"=w626:errorcluster)  [unwired: 10 in]
                            n424 = local write "data file error"(w626) -> ()
                          }
                          frame #1 {
                            n425 = local write "RESULT LAB02-1"(FALSE) -> ()
                            n426 = call "Save data file to network drive v1.vi"("panel id"=w629) -> ("network file save error"=w628:errorcluster)  [unwired: 9 in, 1 out]
                            n427 = local write "data file error"(w628) -> ()
                          }
                        }
                        n428 = Bundle(cluster=w625, "STATUS"="STOP") -> (w623:T4)  [unwired: 2 in]
                        n429 = local write "DISP LAB02-1"(w623) -> ()
                      }
                    }
                  }
                  frame True {
                    # "start new test and create test file"
                    n430 = stacked-sequence {
                      seq-local: [w637 _ _ _ _] -> [_ w662 _ _ _]
                      tunnel: w636 -> [w642 _ _ _ _]
                      tunnel: w635 -> [w639 _ _ _ _]
                      tunnel: w634 -> [w652 _ _ _ _]
                      tunnel: w633 -> [w645 _ _ _ _]
                      tunnel: w632 -> [w640 _ _ _ _]
                      tunnel: [_ w656 _ _ _] -> w631
                      frame #0 {
                        w638 = "\\"
                        n431 = local read "SET LAB02-1"() -> (w647:T5)
                        n432 = case shown="\"CHART TEST\", Default" w652 {
                          tunnel: ["CHART TEST-" "CYCLE TEST-" "T-RISE TEST-"] -> w648
                          frame "CHART TEST", Default {
                          }
                          frame "CYCLE TEST" {
                          }
                          frame "T-RISE TEST" {
                          }
                        }
                        n433 = Unbundle(w647) -> ("DESCRIPTION"=w646:string)  [unwired: 4 out]
                        n434 = Concatenate Strings(w642, "LAB02-1\\", w640, w638, w639, w638) -> (w649:string)
                        n435 = String To Path(string=w649) -> (path=w651:path)
                        n436 = Concatenate Strings(w649, w648, w646, "-", w645, ".tdms") -> (w637:string)
                        n437 = Create Folder(path (use dialog)=w651) -> (error out=w650:errorcluster)  [unwired: 2 in, 2 out]
                        n438 = global write "Global 1.vi" "LAB02-1 FILE"(w637) -> ()
                        n439 = call <vilib>:"Clear Errors.vi"("error in (no error)"=w650) -> ()  [unwired: 6 in, 1 out]
                      }
                      frame #1 {
                        n440 = String To Path(string=w662) -> (path=w657:path)
                        n441 = TDMS Open(5:FALSE, 6:FALSE, 10:T15."create or replace" ("operation (0:open)"), 11:w657) -> (0:w656:errorcluster, 3:→"TDMS LAB02-1":refnum<k34>)  [unwired: 3 in]
                      }
                      frame #2 {
                        n442 = local read "SET LAB02-1"() -> (w668:T5)
                        n443 = local read "TDMS LAB02-1"() -> (w679:refnum<k34>)
                        n444 = Build Array("Testers Name", "Description", "Set Test Cycles", "T-Rise minutes", "T-Rise Deg C") -> (w669:string[])
                        n445 = Unbundle(w668) -> ("NAME"=w667:string, "DESCRIPTION"=w666:string, "CYCLES"=w665:dbl, "T-RISE mins"=w664:dbl, "T-RISE deg C"=w663:dbl)
                        n446 = Number To Decimal String(number=w665) -> (decimal integer string=w678:string)  [unwired: 1 in]
                        n447 = Number To Decimal String(number=w664) -> (decimal integer string=w677:string)  [unwired: 1 in]
                        n448 = Number To Decimal String(number=w663) -> (decimal integer string=w676:string)  [unwired: 1 in]
                        n449 = Build Array(w667, w666, w678, w677, w676) -> (w675:string[])
                        n450 = TDMS Set Properties(5:w675, 7:w669, 11:w679) -> ()  [unwired: 3 in, 4 out]
                      }
                      frame #3 {
                        w681 = 0.0
                        n451 = local read "DISP LAB02-1"() -> (w683:T4)
                        n452 = Bundle(cluster=w683, "CYCLE"=w681, "MINS"=w681, "STATUS"="RUN") -> (w682:T4)
                        n453 = local write "DISP LAB02-1"(w682) -> ()
                      }
                      frame #4 {
                        n454 = local read "SIG LAB02-1"() -> (w686:T2)
                        n455 = local read "TEMP START LAB02-1"() -> (w688:cluster{"TL":dbl, "TN":dbl})
                        n456 = Unbundle(w686) -> ("Tmp Live"=w685:dbl, "Tmp Neut"=w684:dbl)  [unwired: 3 out]
                        n457 = Bundle(cluster=w688, "TL"=w685, "TN"=w684) -> (w687:cluster{"TL":dbl, "TN":dbl})
                        n458 = local write "TEMP START LAB02-1"(w687) -> ()
                      }
                    }
                  }
                }
              }
              event "RUN LAB02-2": Value Change {
                n459 = event-data() -> ("NewVal"=w689:bool)  [unwired: 1 in, 5 out]
                n460 = local write "run lab02-2"(w689) -> ()
                n461 = case shown="False" w689 {
                  tunnel: w695 -> [_ w728]
                  tunnel: w694 -> [_ w727]
                  tunnel: w692 -> [w697 w726]
                  tunnel: w693 -> [_ w725]
                  tunnel: w691 -> [_ w724]
                  tunnel: [w696 w723] -> w690
                  frame False {
                    # "stop test"
                    n462 = stacked-sequence {
                      tunnel: w697 -> [w706 _]
                      tunnel: [w698 _] -> w696
                      frame #0 {
                        n463 = local read "DISP LAB02-2"() -> (w705:T4)
                        n464 = Unbundle(w705) -> ("CYCLE"=w703:dbl, "MINS"=w704:dbl)  [unwired: 1 out]
                        n465 = case shown="\"CYCLE TEST\"" w706 {
                          tunnel: w704 -> [_ _ w713]
                          tunnel: w703 -> [w711 w712 _]
                          tunnel: [w711 w712 w713] -> w702
                          frame "CHART TEST", Default {
                          }
                          frame "CYCLE TEST" {
                          }
                          frame "T-RISE TEST" {
                          }
                        }
                        n466 = local read "TDMS LAB02-2"() -> (w710:refnum<k34>)
                        n467 = Build Array("STOPPED") -> (w707:string[])
                        n468 = Build Array(w702) -> (w701:dbl[])
                        n469 = TDMS Write(0:w710, 5:"TEST RESULT", 7:w707, 9:w701) -> (4:w699:refnum<k34>, 15:w700:errorcluster)  [unwired: 2 in, 2 out]
                        n470 = TDMS Close(8:w700, 11:w699) -> (0:w698:errorcluster)  [unwired: 1 out]
                      }
                      frame #1 {
                        n471 = local read "DISP LAB02-2"() -> (w717:T4)
                        n472 = stacked-sequence {
                          tunnel: "LAB02-2" -> [w719 w721]
                          frame #0 {
                            n473 = call "sub vi - defrag tdms v1.vi"("panel id"=w719) -> ("error out"=w718:errorcluster)  [unwired: 10 in]
                            n474 = local write "data file error"(w718) -> ()
                          }
                          frame #1 {
                            n475 = call "Save data file to network drive v1.vi"("panel id"=w721) -> ("network file save error"=w720:errorcluster)  [unwired: 9 in, 1 out]
                            n476 = local write "RESULT LAB02-2"(FALSE) -> ()
                            n477 = local write "data file error"(w720) -> ()
                          }
                        }
                        n478 = Bundle(cluster=w717, "STATUS"="STOP") -> (w715:T4)  [unwired: 2 in]
                        n479 = local write "DISP LAB02-2"(w715) -> ()
                      }
                    }
                  }
                  frame True {
                    # "start new test and create test file"
                    n480 = stacked-sequence {
                      seq-local: [w729 _ _ _ _] -> [_ w754 _ _ _]
                      tunnel: w728 -> [w734 _ _ _ _]
                      tunnel: w727 -> [w731 _ _ _ _]
                      tunnel: w726 -> [w744 _ _ _ _]
                      tunnel: w725 -> [w737 _ _ _ _]
                      tunnel: w724 -> [w732 _ _ _ _]
                      tunnel: [_ w748 _ _ _] -> w723
                      frame #0 {
                        w730 = "\\"
                        n481 = local read "SET LAB02-2"() -> (w739:T5)
                        n482 = case shown="\"CHART TEST\", Default" w744 {
                          tunnel: ["CHART TEST-" "CYCLE TEST-" "T-RISE TEST-"] -> w740
                          frame "CHART TEST", Default {
                          }
                          frame "CYCLE TEST" {
                          }
                          frame "T-RISE TEST" {
                          }
                        }
                        n483 = Unbundle(w739) -> ("DESCRIPTION"=w738:string)  [unwired: 4 out]
                        n484 = Concatenate Strings(w734, "LAB02-2\\", w732, w730, w731, w730) -> (w741:string)
                        n485 = String To Path(string=w741) -> (path=w743:path)
                        n486 = Concatenate Strings(w741, w740, w738, "-", w737, ".tdms") -> (w729:string)
                        n487 = Create Folder(path (use dialog)=w743) -> (error out=w742:errorcluster)  [unwired: 2 in, 2 out]
                        n488 = global write "Global 1.vi" "LAB02-2 FILE"(w729) -> ()
                        n489 = call <vilib>:"Clear Errors.vi"("error in (no error)"=w742) -> ()  [unwired: 6 in, 1 out]
                      }
                      frame #1 {
                        n490 = String To Path(string=w754) -> (path=w749:path)
                        n491 = TDMS Open(5:FALSE, 6:FALSE, 10:T15."create or replace" ("operation (0:open)"), 11:w749) -> (0:w748:errorcluster, 3:→"TDMS LAB02-2":refnum<k34>)  [unwired: 3 in]
                      }
                      frame #2 {
                        n492 = local read "SET LAB02-2"() -> (w760:T5)
                        n493 = local read "TDMS LAB02-2"() -> (w771:refnum<k34>)
                        n494 = Build Array("Testers Name", "Description", "Set Test Cycles", "T-Rise minutes", "T-Rise Deg C") -> (w761:string[])
                        n495 = Unbundle(w760) -> ("NAME"=w759:string, "DESCRIPTION"=w758:string, "CYCLES"=w757:dbl, "T-RISE mins"=w756:dbl, "T-RISE deg C"=w755:dbl)
                        n496 = Number To Decimal String(number=w757) -> (decimal integer string=w770:string)  [unwired: 1 in]
                        n497 = Number To Decimal String(number=w756) -> (decimal integer string=w769:string)  [unwired: 1 in]
                        n498 = Number To Decimal String(number=w755) -> (decimal integer string=w768:string)  [unwired: 1 in]
                        n499 = Build Array(w759, w758, w770, w769, w768) -> (w767:string[])
                        n500 = TDMS Set Properties(5:w767, 7:w761, 11:w771) -> ()  [unwired: 3 in, 4 out]
                      }
                      frame #3 {
                        w773 = 0.0
                        n501 = local read "DISP LAB02-2"() -> (w775:T4)
                        n502 = Bundle(cluster=w775, "CYCLE"=w773, "MINS"=w773, "STATUS"="RUN") -> (w774:T4)
                        n503 = local write "DISP LAB02-2"(w774) -> ()
                      }
                      frame #4 {
                        n504 = local read "SIG LAB02-2"() -> (w778:T2)
                        n505 = local read "TEMP START LAB02-2"() -> (w780:cluster{"TL":dbl, "TN":dbl})
                        n506 = Unbundle(w778) -> ("Tmp Live"=w777:dbl, "Tmp Neut"=w776:dbl)  [unwired: 3 out]
                        n507 = Bundle(cluster=w780, "TL"=w777, "TN"=w776) -> (w779:cluster{"TL":dbl, "TN":dbl})
                        n508 = local write "TEMP START LAB02-2"(w779) -> ()
                      }
                    }
                  }
                }
              }
              event "RUN LAB03-1": Value Change {
                n509 = event-data() -> ("NewVal"=w781:bool)  [unwired: 1 in, 5 out]
                n510 = local write "run lab03-1"(w781) -> ()
                n511 = case shown="False" w781 {
                  tunnel: w787 -> [_ w820]
                  tunnel: w786 -> [_ w819]
                  tunnel: w784 -> [w789 w818]
                  tunnel: w785 -> [_ w817]
                  tunnel: w783 -> [_ w816]
                  tunnel: [w788 w815] -> w782
                  frame False {
                    # "stop test"
                    n512 = stacked-sequence {
                      tunnel: w789 -> [w798 _]
                      tunnel: [w790 _] -> w788
                      frame #0 {
                        n513 = local read "DISP LAB03-1"() -> (w797:T4)
                        n514 = Unbundle(w797) -> ("CYCLE"=w795:dbl, "MINS"=w796:dbl)  [unwired: 1 out]
                        n515 = case shown="\"CYCLE TEST\"" w798 {
                          tunnel: w796 -> [_ _ w805]
                          tunnel: w795 -> [w803 w804 _]
                          tunnel: [w803 w804 w805] -> w794
                          frame "CHART TEST", Default {
                          }
                          frame "CYCLE TEST" {
                          }
                          frame "T-RISE TEST" {
                          }
                        }
                        n516 = local read "TDMS LAB03-1"() -> (w802:refnum<k34>)
                        n517 = Build Array("STOPPED") -> (w799:string[])
                        n518 = Build Array(w794) -> (w793:dbl[])
                        n519 = TDMS Write(0:w802, 5:"TEST RESULT", 7:w799, 9:w793) -> (4:w791:refnum<k34>, 15:w792:errorcluster)  [unwired: 2 in, 2 out]
                        n520 = TDMS Close(8:w792, 11:w791) -> (0:w790:errorcluster)  [unwired: 1 out]
                      }
                      frame #1 {
                        n521 = local read "DISP LAB03-1"() -> (w809:T4)
                        n522 = stacked-sequence {
                          tunnel: "LAB03-1" -> [w811 w813]
                          frame #0 {
                            n523 = call "sub vi - defrag tdms v1.vi"("panel id"=w811) -> ("error out"=w810:errorcluster)  [unwired: 10 in]
                            n524 = local write "data file error"(w810) -> ()
                          }
                          frame #1 {
                            n525 = call "Save data file to network drive v1.vi"("panel id"=w813) -> ("network file save error"=w812:errorcluster)  [unwired: 9 in, 1 out]
                            n526 = local write "RESULT LAB03-1"(FALSE) -> ()
                            n527 = local write "data file error"(w812) -> ()
                          }
                        }
                        n528 = Bundle(cluster=w809, "STATUS"="STOP") -> (w807:T4)  [unwired: 2 in]
                        n529 = local write "DISP LAB03-1"(w807) -> ()
                      }
                    }
                  }
                  frame True {
                    # "start new test and create test file"
                    n530 = stacked-sequence {
                      seq-local: [w821 _ _ _ _] -> [_ w846 _ _ _]
                      tunnel: w820 -> [w826 _ _ _ _]
                      tunnel: w819 -> [w823 _ _ _ _]
                      tunnel: w818 -> [w836 _ _ _ _]
                      tunnel: w817 -> [w829 _ _ _ _]
                      tunnel: w816 -> [w824 _ _ _ _]
                      tunnel: [_ w840 _ _ _] -> w815
                      frame #0 {
                        w822 = "\\"
                        n531 = local read "SET LAB03-1"() -> (w831:T5)
                        n532 = case shown="\"CHART TEST\", Default" w836 {
                          tunnel: ["CHART TEST-" "CYCLE TEST-" "T-RISE TEST-"] -> w832
                          frame "CHART TEST", Default {
                          }
                          frame "CYCLE TEST" {
                          }
                          frame "T-RISE TEST" {
                          }
                        }
                        n533 = Unbundle(w831) -> ("DESCRIPTION"=w830:string)  [unwired: 4 out]
                        n534 = Concatenate Strings(w826, "LAB03-1\\", w824, w822, w823, w822) -> (w833:string)
                        n535 = String To Path(string=w833) -> (path=w835:path)
                        n536 = Concatenate Strings(w833, w832, w830, "-", w829, ".tdms") -> (w821:string)
                        n537 = Create Folder(path (use dialog)=w835) -> (error out=w834:errorcluster)  [unwired: 2 in, 2 out]
                        n538 = global write "Global 1.vi" "LAB03-1 FILE"(w821) -> ()
                        n539 = call <vilib>:"Clear Errors.vi"("error in (no error)"=w834) -> ()  [unwired: 6 in, 1 out]
                      }
                      frame #1 {
                        n540 = String To Path(string=w846) -> (path=w841:path)
                        n541 = TDMS Open(5:FALSE, 6:FALSE, 10:T15."create or replace" ("operation (0:open)"), 11:w841) -> (0:w840:errorcluster, 3:→"TDMS LAB03-1":refnum<k34>)  [unwired: 3 in]
                      }
                      frame #2 {
                        n542 = local read "SET LAB03-1"() -> (w852:T5)
                        n543 = local read "TDMS LAB03-1"() -> (w863:refnum<k34>)
                        n544 = Build Array("Testers Name", "Description", "Set Test Cycles", "T-Rise minutes", "T-Rise Deg C") -> (w853:string[])
                        n545 = Unbundle(w852) -> ("NAME"=w851:string, "DESCRIPTION"=w850:string, "CYCLES"=w849:dbl, "T-RISE mins"=w848:dbl, "T-RISE deg C"=w847:dbl)
                        n546 = Number To Decimal String(number=w849) -> (decimal integer string=w862:string)  [unwired: 1 in]
                        n547 = Number To Decimal String(number=w848) -> (decimal integer string=w861:string)  [unwired: 1 in]
                        n548 = Number To Decimal String(number=w847) -> (decimal integer string=w860:string)  [unwired: 1 in]
                        n549 = Build Array(w851, w850, w862, w861, w860) -> (w859:string[])
                        n550 = TDMS Set Properties(5:w859, 7:w853, 11:w863) -> ()  [unwired: 3 in, 4 out]
                      }
                      frame #3 {
                        w865 = 0.0
                        n551 = local read "DISP LAB03-1"() -> (w867:T4)
                        n552 = Bundle(cluster=w867, "CYCLE"=w865, "MINS"=w865, "STATUS"="RUN") -> (w866:T4)
                        n553 = local write "DISP LAB03-1"(w866) -> ()
                      }
                      frame #4 {
                        n554 = local read "SIG LAB03-1"() -> (w870:T2)
                        n555 = local read "TEMP START LAB03-1"() -> (w872:cluster{"TL":dbl, "TN":dbl})
                        n556 = Unbundle(w870) -> ("Tmp Live"=w869:dbl, "Tmp Neut"=w868:dbl)  [unwired: 3 out]
                        n557 = Bundle(cluster=w872, "TL"=w869, "TN"=w868) -> (w871:cluster{"TL":dbl, "TN":dbl})
                        n558 = local write "TEMP START LAB03-1"(w871) -> ()
                      }
                    }
                  }
                }
              }
              event "RUN LAB03-2": Value Change {
                n559 = event-data() -> ("NewVal"=w873:bool)  [unwired: 1 in, 5 out]
                n560 = local write "run lab03-2"(w873) -> ()
                n561 = case shown="False" w873 {
                  tunnel: w879 -> [_ w912]
                  tunnel: w878 -> [_ w911]
                  tunnel: w876 -> [w881 w910]
                  tunnel: w877 -> [_ w909]
                  tunnel: w875 -> [_ w908]
                  tunnel: [w880 w907] -> w874
                  frame False {
                    # "stop test"
                    n562 = stacked-sequence {
                      tunnel: w881 -> [w890 _]
                      tunnel: [w882 _] -> w880
                      frame #0 {
                        n563 = local read "DISP LAB03-2"() -> (w889:T4)
                        n564 = Unbundle(w889) -> ("CYCLE"=w887:dbl, "MINS"=w888:dbl)  [unwired: 1 out]
                        n565 = case shown="\"CYCLE TEST\"" w890 {
                          tunnel: w888 -> [_ _ w897]
                          tunnel: w887 -> [w895 w896 _]
                          tunnel: [w895 w896 w897] -> w886
                          frame "CHART TEST", Default {
                          }
                          frame "CYCLE TEST" {
                          }
                          frame "T-RISE TEST" {
                          }
                        }
                        n566 = local read "TDMS LAB03-2"() -> (w894:refnum<k34>)
                        n567 = Build Array("STOPPED") -> (w891:string[])
                        n568 = Build Array(w886) -> (w885:dbl[])
                        n569 = TDMS Write(0:w894, 5:"TEST RESULT", 7:w891, 9:w885) -> (4:w883:refnum<k34>, 15:w884:errorcluster)  [unwired: 2 in, 2 out]
                        n570 = TDMS Close(8:w884, 11:w883) -> (0:w882:errorcluster)  [unwired: 1 out]
                      }
                      frame #1 {
                        n571 = local read "DISP LAB03-2"() -> (w901:T4)
                        n572 = stacked-sequence {
                          tunnel: "LAB03-2" -> [w903 w905]
                          frame #0 {
                            n573 = call "sub vi - defrag tdms v1.vi"("panel id"=w903) -> ("error out"=w902:errorcluster)  [unwired: 10 in]
                            n574 = local write "data file error"(w902) -> ()
                          }
                          frame #1 {
                            n575 = call "Save data file to network drive v1.vi"("panel id"=w905) -> ("network file save error"=w904:errorcluster)  [unwired: 9 in, 1 out]
                            n576 = local write "RESULT LAB03-2"(FALSE) -> ()
                            n577 = local write "data file error"(w904) -> ()
                          }
                        }
                        n578 = Bundle(cluster=w901, "STATUS"="STOP") -> (w899:T4)  [unwired: 2 in]
                        n579 = local write "DISP LAB03-2"(w899) -> ()
                      }
                    }
                  }
                  frame True {
                    # "start new test and create test file"
                    n580 = stacked-sequence {
                      seq-local: [w913 _ _ _ _] -> [_ w938 _ _ _]
                      tunnel: w912 -> [w918 _ _ _ _]
                      tunnel: w911 -> [w915 _ _ _ _]
                      tunnel: w910 -> [w928 _ _ _ _]
                      tunnel: w909 -> [w921 _ _ _ _]
                      tunnel: w908 -> [w916 _ _ _ _]
                      tunnel: [_ w932 _ _ _] -> w907
                      frame #0 {
                        w914 = "\\"
                        n581 = local read "SET LAB03-2"() -> (w923:T5)
                        n582 = case shown="\"CHART TEST\", Default" w928 {
                          tunnel: ["CHART TEST-" "CYCLE TEST-" "T-RISE TEST-"] -> w924
                          frame "CHART TEST", Default {
                          }
                          frame "CYCLE TEST" {
                          }
                          frame "T-RISE TEST" {
                          }
                        }
                        n583 = Unbundle(w923) -> ("DESCRIPTION"=w922:string)  [unwired: 4 out]
                        n584 = Concatenate Strings(w918, "LAB03-2\\", w916, w914, w915, w914) -> (w925:string)
                        n585 = String To Path(string=w925) -> (path=w927:path)
                        n586 = Concatenate Strings(w925, w924, w922, "-", w921, ".tdms") -> (w913:string)
                        n587 = Create Folder(path (use dialog)=w927) -> (error out=w926:errorcluster)  [unwired: 2 in, 2 out]
                        n588 = global write "Global 1.vi" "LAB03-2 FILE"(w913) -> ()
                        n589 = call <vilib>:"Clear Errors.vi"("error in (no error)"=w926) -> ()  [unwired: 6 in, 1 out]
                      }
                      frame #1 {
                        n590 = String To Path(string=w938) -> (path=w933:path)
                        n591 = TDMS Open(5:FALSE, 6:FALSE, 10:T15."create or replace" ("operation (0:open)"), 11:w933) -> (0:w932:errorcluster, 3:→"TDMS LAB03-2":refnum<k34>)  [unwired: 3 in]
                      }
                      frame #2 {
                        n592 = local read "SET LAB03-2"() -> (w944:T5)
                        n593 = local read "TDMS LAB03-2"() -> (w955:refnum<k34>)
                        n594 = Build Array("Testers Name", "Description", "Set Test Cycles", "T-Rise minutes", "T-Rise Deg C") -> (w945:string[])
                        n595 = Unbundle(w944) -> ("NAME"=w943:string, "DESCRIPTION"=w942:string, "CYCLES"=w941:dbl, "T-RISE mins"=w940:dbl, "T-RISE deg C"=w939:dbl)
                        n596 = Number To Decimal String(number=w941) -> (decimal integer string=w954:string)  [unwired: 1 in]
                        n597 = Number To Decimal String(number=w940) -> (decimal integer string=w953:string)  [unwired: 1 in]
                        n598 = Number To Decimal String(number=w939) -> (decimal integer string=w952:string)  [unwired: 1 in]
                        n599 = Build Array(w943, w942, w954, w953, w952) -> (w951:string[])
                        n600 = TDMS Set Properties(5:w951, 7:w945, 11:w955) -> ()  [unwired: 3 in, 4 out]
                      }
                      frame #3 {
                        w957 = 0.0
                        n601 = local read "DISP LAB03-2"() -> (w959:T4)
                        n602 = Bundle(cluster=w959, "CYCLE"=w957, "MINS"=w957, "STATUS"="RUN") -> (w958:T4)
                        n603 = local write "DISP LAB03-2"(w958) -> ()
                      }
                      frame #4 {
                        n604 = local read "SIG LAB03-2"() -> (w962:T2)
                        n605 = local read "TEMP START LAB03-2"() -> (w964:cluster{"TL":dbl, "TN":dbl})
                        n606 = Unbundle(w962) -> ("Tmp Live"=w961:dbl, "Tmp Neut"=w960:dbl)  [unwired: 3 out]
                        n607 = Bundle(cluster=w964, "TL"=w961, "TN"=w960) -> (w963:cluster{"TL":dbl, "TN":dbl})
                        n608 = local write "TEMP START LAB03-2"(w963) -> ()
                      }
                    }
                  }
                }
              }
              event "RUN LAB04-1": Value Change {
                n609 = event-data() -> ("NewVal"=w965:bool)  [unwired: 1 in, 5 out]
                n610 = local write "run lab04-1"(w965) -> ()
                n611 = case shown="False" w965 {
                  tunnel: w971 -> [_ w1004]
                  tunnel: w970 -> [_ w1003]
                  tunnel: w968 -> [w973 w1002]
                  tunnel: w969 -> [_ w1001]
                  tunnel: w967 -> [_ w1000]
                  tunnel: [w972 w999] -> w966
                  frame False {
                    # "stop test"
                    n612 = stacked-sequence {
                      tunnel: w973 -> [w982 _]
                      tunnel: [w974 _] -> w972
                      frame #0 {
                        n613 = local read "DISP LAB04-1"() -> (w981:T4)
                        n614 = Unbundle(w981) -> ("CYCLE"=w979:dbl, "MINS"=w980:dbl)  [unwired: 1 out]
                        n615 = case shown="\"CYCLE TEST\"" w982 {
                          tunnel: w980 -> [_ _ w989]
                          tunnel: w979 -> [w987 w988 _]
                          tunnel: [w987 w988 w989] -> w978
                          frame "CHART TEST", Default {
                          }
                          frame "CYCLE TEST" {
                          }
                          frame "T-RISE TEST" {
                          }
                        }
                        n616 = local read "TDMS LAB04-1"() -> (w986:refnum<k34>)
                        n617 = Build Array("STOPPED") -> (w983:string[])
                        n618 = Build Array(w978) -> (w977:dbl[])
                        n619 = TDMS Write(0:w986, 5:"TEST RESULT", 7:w983, 9:w977) -> (4:w975:refnum<k34>, 15:w976:errorcluster)  [unwired: 2 in, 2 out]
                        n620 = TDMS Close(8:w976, 11:w975) -> (0:w974:errorcluster)  [unwired: 1 out]
                      }
                      frame #1 {
                        n621 = local read "DISP LAB04-1"() -> (w993:T4)
                        n622 = stacked-sequence {
                          tunnel: "LAB04-1" -> [w995 w997]
                          frame #0 {
                            n623 = call "sub vi - defrag tdms v1.vi"("panel id"=w995) -> ("error out"=w994:errorcluster)  [unwired: 10 in]
                            n624 = local write "data file error"(w994) -> ()
                          }
                          frame #1 {
                            n625 = call "Save data file to network drive v1.vi"("panel id"=w997) -> ("network file save error"=w996:errorcluster)  [unwired: 9 in, 1 out]
                            n626 = local write "RESULT LAB04-1"(FALSE) -> ()
                            n627 = local write "data file error"(w996) -> ()
                          }
                        }
                        n628 = Bundle(cluster=w993, "STATUS"="STOP") -> (w991:T4)  [unwired: 2 in]
                        n629 = local write "DISP LAB04-1"(w991) -> ()
                      }
                    }
                  }
                  frame True {
                    # "start new test and create test file"
                    n630 = stacked-sequence {
                      seq-local: [w1005 _ _ _ _] -> [_ w1030 _ _ _]
                      tunnel: w1004 -> [w1010 _ _ _ _]
                      tunnel: w1003 -> [w1006 _ _ _ _]
                      tunnel: w1002 -> [w1020 _ _ _ _]
                      tunnel: w1001 -> [w1013 _ _ _ _]
                      tunnel: w1000 -> [w1008 _ _ _ _]
                      tunnel: [_ w1024 _ _ _] -> w999
                      frame #0 {
                        w1007 = "\\"
                        n631 = local read "SET LAB04-1"() -> (w1015:T5)
                        n632 = case shown="\"CHART TEST\", Default" w1020 {
                          tunnel: ["CHART TEST-" "CYCLE TEST-" "T-RISE TEST-"] -> w1016
                          frame "CHART TEST", Default {
                          }
                          frame "CYCLE TEST" {
                          }
                          frame "T-RISE TEST" {
                          }
                        }
                        n633 = Unbundle(w1015) -> ("DESCRIPTION"=w1014:string)  [unwired: 4 out]
                        n634 = Concatenate Strings(w1010, "LAB04-1\\", w1008, w1007, w1006, w1007) -> (w1017:string)
                        n635 = String To Path(string=w1017) -> (path=w1019:path)
                        n636 = Concatenate Strings(w1017, w1016, w1014, "-", w1013, ".tdms") -> (w1005:string)
                        n637 = Create Folder(path (use dialog)=w1019) -> (error out=w1018:errorcluster)  [unwired: 2 in, 2 out]
                        n638 = global write "Global 1.vi" "LAB04-1 FILE"(w1005) -> ()
                        n639 = call <vilib>:"Clear Errors.vi"("error in (no error)"=w1018) -> ()  [unwired: 6 in, 1 out]
                      }
                      frame #1 {
                        n640 = String To Path(string=w1030) -> (path=w1025:path)
                        n641 = TDMS Open(5:FALSE, 6:FALSE, 10:T15."create or replace" ("operation (0:open)"), 11:w1025) -> (0:w1024:errorcluster, 3:→"TDMS LAB04-1":refnum<k34>)  [unwired: 3 in]
                      }
                      frame #2 {
                        n642 = local read "SET LAB04-1"() -> (w1036:T5)
                        n643 = local read "TDMS LAB04-1"() -> (w1047:refnum<k34>)
                        n644 = Build Array("Testers Name", "Description", "Set Test Cycles", "T-Rise minutes", "T-Rise Deg C") -> (w1037:string[])
                        n645 = Unbundle(w1036) -> ("NAME"=w1035:string, "DESCRIPTION"=w1034:string, "CYCLES"=w1033:dbl, "T-RISE mins"=w1032:dbl, "T-RISE deg C"=w1031:dbl)
                        n646 = Number To Decimal String(number=w1033) -> (decimal integer string=w1046:string)  [unwired: 1 in]
                        n647 = Number To Decimal String(number=w1032) -> (decimal integer string=w1045:string)  [unwired: 1 in]
                        n648 = Number To Decimal String(number=w1031) -> (decimal integer string=w1044:string)  [unwired: 1 in]
                        n649 = Build Array(w1035, w1034, w1046, w1045, w1044) -> (w1043:string[])
                        n650 = TDMS Set Properties(5:w1043, 7:w1037, 11:w1047) -> ()  [unwired: 3 in, 4 out]
                      }
                      frame #3 {
                        w1049 = 0.0
                        n651 = local read "DISP LAB04-1"() -> (w1051:T4)
                        n652 = Bundle(cluster=w1051, "CYCLE"=w1049, "MINS"=w1049, "STATUS"="RUN") -> (w1050:T4)
                        n653 = local write "DISP LAB04-1"(w1050) -> ()
                      }
                      frame #4 {
                        n654 = local read "SIG LAB04-1"() -> (w1054:T2)
                        n655 = local read "TEMP START LAB04-1"() -> (w1056:cluster{"TL":dbl, "TN":dbl})
                        n656 = Unbundle(w1054) -> ("Tmp Live"=w1053:dbl, "Tmp Neut"=w1052:dbl)  [unwired: 3 out]
                        n657 = Bundle(cluster=w1056, "TL"=w1053, "TN"=w1052) -> (w1055:cluster{"TL":dbl, "TN":dbl})
                        n658 = local write "TEMP START LAB04-1"(w1055) -> ()
                      }
                    }
                  }
                }
              }
              event "RUN LAB04-2": Value Change {
                n659 = event-data() -> ("NewVal"=w1057:bool)  [unwired: 1 in, 5 out]
                n660 = local write "run lab04-2"(w1057) -> ()
                n661 = case shown="False" w1057 {
                  tunnel: w1063 -> [_ w1096]
                  tunnel: w1062 -> [_ w1095]
                  tunnel: w1060 -> [w1065 w1094]
                  tunnel: w1061 -> [_ w1093]
                  tunnel: w1059 -> [_ w1092]
                  tunnel: [w1064 w1091] -> w1058
                  frame False {
                    # "stop test"
                    n662 = stacked-sequence {
                      tunnel: w1065 -> [w1074 _]
                      tunnel: [w1066 _] -> w1064
                      frame #0 {
                        n663 = local read "DISP LAB04-2"() -> (w1073:T4)
                        n664 = Unbundle(w1073) -> ("CYCLE"=w1071:dbl, "MINS"=w1072:dbl)  [unwired: 1 out]
                        n665 = case shown="\"CYCLE TEST\"" w1074 {
                          tunnel: w1072 -> [_ _ w1081]
                          tunnel: w1071 -> [w1079 w1080 _]
                          tunnel: [w1079 w1080 w1081] -> w1070
                          frame "CHART TEST", Default {
                          }
                          frame "CYCLE TEST" {
                          }
                          frame "T-RISE TEST" {
                          }
                        }
                        n666 = local read "TDMS LAB04-2"() -> (w1078:refnum<k34>)
                        n667 = Build Array("STOPPED") -> (w1075:string[])
                        n668 = Build Array(w1070) -> (w1069:dbl[])
                        n669 = TDMS Write(0:w1078, 5:"TEST RESULT", 7:w1075, 9:w1069) -> (4:w1067:refnum<k34>, 15:w1068:errorcluster)  [unwired: 2 in, 2 out]
                        n670 = TDMS Close(8:w1068, 11:w1067) -> (0:w1066:errorcluster)  [unwired: 1 out]
                      }
                      frame #1 {
                        n671 = local read "DISP LAB04-2"() -> (w1085:T4)
                        n672 = stacked-sequence {
                          tunnel: "LAB04-2" -> [w1087 w1089]
                          frame #0 {
                            n673 = call "sub vi - defrag tdms v1.vi"("panel id"=w1087) -> ("error out"=w1086:errorcluster)  [unwired: 10 in]
                            n674 = local write "data file error"(w1086) -> ()
                          }
                          frame #1 {
                            n675 = call "Save data file to network drive v1.vi"("panel id"=w1089) -> ("network file save error"=w1088:errorcluster)  [unwired: 9 in, 1 out]
                            n676 = local write "RESULT LAB04-2"(FALSE) -> ()
                            n677 = local write "data file error"(w1088) -> ()
                          }
                        }
                        n678 = Bundle(cluster=w1085, "STATUS"="STOP") -> (w1083:T4)  [unwired: 2 in]
                        n679 = local write "DISP LAB04-2"(w1083) -> ()
                      }
                    }
                  }
                  frame True {
                    # "start new test and create test file"
                    n680 = stacked-sequence {
                      seq-local: [w1097 _ _ _ _] -> [_ w1122 _ _ _]
                      tunnel: w1096 -> [w1102 _ _ _ _]
                      tunnel: w1095 -> [w1098 _ _ _ _]
                      tunnel: w1094 -> [w1112 _ _ _ _]
                      tunnel: w1093 -> [w1105 _ _ _ _]
                      tunnel: w1092 -> [w1100 _ _ _ _]
                      tunnel: [_ w1116 _ _ _] -> w1091
                      frame #0 {
                        w1099 = "\\"
                        n681 = local read "SET LAB04-2"() -> (w1107:T5)
                        n682 = case shown="\"CHART TEST\", Default" w1112 {
                          tunnel: ["CHART TEST-" "CYCLE TEST-" "T-RISE TEST-"] -> w1108
                          frame "CHART TEST", Default {
                          }
                          frame "CYCLE TEST" {
                          }
                          frame "T-RISE TEST" {
                          }
                        }
                        n683 = Unbundle(w1107) -> ("DESCRIPTION"=w1106:string)  [unwired: 4 out]
                        n684 = Concatenate Strings(w1102, "LAB04-2\\", w1100, w1099, w1098, w1099) -> (w1109:string)
                        n685 = String To Path(string=w1109) -> (path=w1111:path)
                        n686 = Concatenate Strings(w1109, w1108, w1106, "-", w1105, ".tdms") -> (w1097:string)
                        n687 = Create Folder(path (use dialog)=w1111) -> (error out=w1110:errorcluster)  [unwired: 2 in, 2 out]
                        n688 = global write "Global 1.vi" "LAB04-2 FILE"(w1097) -> ()
                        n689 = call <vilib>:"Clear Errors.vi"("error in (no error)"=w1110) -> ()  [unwired: 6 in, 1 out]
                      }
                      frame #1 {
                        n690 = String To Path(string=w1122) -> (path=w1117:path)
                        n691 = TDMS Open(5:FALSE, 6:FALSE, 10:T15."create or replace" ("operation (0:open)"), 11:w1117) -> (0:w1116:errorcluster, 3:→"TDMS LAB04-2":refnum<k34>)  [unwired: 3 in]
                      }
                      frame #2 {
                        n692 = local read "SET LAB04-2"() -> (w1128:T5)
                        n693 = local read "TDMS LAB04-2"() -> (w1139:refnum<k34>)
                        n694 = Build Array("Testers Name", "Description", "Set Test Cycles", "T-Rise minutes", "T-Rise Deg C") -> (w1129:string[])
                        n695 = Unbundle(w1128) -> ("NAME"=w1127:string, "DESCRIPTION"=w1126:string, "CYCLES"=w1125:dbl, "T-RISE mins"=w1124:dbl, "T-RISE deg C"=w1123:dbl)
                        n696 = Number To Decimal String(number=w1125) -> (decimal integer string=w1138:string)  [unwired: 1 in]
                        n697 = Number To Decimal String(number=w1124) -> (decimal integer string=w1137:string)  [unwired: 1 in]
                        n698 = Number To Decimal String(number=w1123) -> (decimal integer string=w1136:string)  [unwired: 1 in]
                        n699 = Build Array(w1127, w1126, w1138, w1137, w1136) -> (w1135:string[])
                        n700 = TDMS Set Properties(5:w1135, 7:w1129, 11:w1139) -> ()  [unwired: 3 in, 4 out]
                      }
                      frame #3 {
                        w1141 = 0.0
                        n701 = local read "DISP LAB04-2"() -> (w1143:T4)
                        n702 = Bundle(cluster=w1143, "CYCLE"=w1141, "MINS"=w1141, "STATUS"="RUN") -> (w1142:T4)
                        n703 = local write "DISP LAB04-2"(w1142) -> ()
                      }
                      frame #4 {
                        n704 = local read "SIG LAB04-2"() -> (w1146:T2)
                        n705 = local read "TEMP START LAB04-2"() -> (w1148:cluster{"TL":dbl, "TN":dbl})
                        n706 = Unbundle(w1146) -> ("Tmp Live"=w1145:dbl, "Tmp Neut"=w1144:dbl)  [unwired: 3 out]
                        n707 = Bundle(cluster=w1148, "TL"=w1145, "TN"=w1144) -> (w1147:cluster{"TL":dbl, "TN":dbl})
                        n708 = local write "TEMP START LAB04-2"(w1147) -> ()
                      }
                    }
                  }
                }
              }
              event "RUN LAB05-1": Value Change {
                n709 = event-data() -> ("NewVal"=w1149:bool)  [unwired: 1 in, 5 out]
                n710 = local write "run lab05-1"(w1149) -> ()
                n711 = case shown="False" w1149 {
                  tunnel: w1155 -> [_ w1188]
                  tunnel: w1154 -> [_ w1187]
                  tunnel: w1152 -> [w1157 w1186]
                  tunnel: w1153 -> [_ w1185]
                  tunnel: w1151 -> [_ w1184]
                  tunnel: [w1156 w1183] -> w1150
                  frame False {
                    # "stop test"
                    n712 = stacked-sequence {
                      tunnel: w1157 -> [w1166 _]
                      tunnel: [w1158 _] -> w1156
                      frame #0 {
                        n713 = local read "DISP LAB05-1"() -> (w1165:T4)
                        n714 = Unbundle(w1165) -> ("CYCLE"=w1163:dbl, "MINS"=w1164:dbl)  [unwired: 1 out]
                        n715 = case shown="\"CYCLE TEST\"" w1166 {
                          tunnel: w1164 -> [_ _ w1173]
                          tunnel: w1163 -> [w1171 w1172 _]
                          tunnel: [w1171 w1172 w1173] -> w1162
                          frame "CHART TEST", Default {
                          }
                          frame "CYCLE TEST" {
                          }
                          frame "T-RISE TEST" {
                          }
                        }
                        n716 = local read "TDMS LAB05-1"() -> (w1170:refnum<k34>)
                        n717 = Build Array("STOPPED") -> (w1167:string[])
                        n718 = Build Array(w1162) -> (w1161:dbl[])
                        n719 = TDMS Write(0:w1170, 5:"TEST RESULT", 7:w1167, 9:w1161) -> (4:w1159:refnum<k34>, 15:w1160:errorcluster)  [unwired: 2 in, 2 out]
                        n720 = TDMS Close(8:w1160, 11:w1159) -> (0:w1158:errorcluster)  [unwired: 1 out]
                      }
                      frame #1 {
                        n721 = local read "DISP LAB05-1"() -> (w1177:T4)
                        n722 = stacked-sequence {
                          tunnel: "LAB05-1" -> [w1179 w1181]
                          frame #0 {
                            n723 = call "sub vi - defrag tdms v1.vi"("panel id"=w1179) -> ("error out"=w1178:errorcluster)  [unwired: 10 in]
                            n724 = local write "data file error"(w1178) -> ()
                          }
                          frame #1 {
                            n725 = call "Save data file to network drive v1.vi"("panel id"=w1181) -> ("network file save error"=w1180:errorcluster)  [unwired: 9 in, 1 out]
                            n726 = local write "RESULT LAB05-1"(FALSE) -> ()
                            n727 = local write "data file error"(w1180) -> ()
                          }
                        }
                        n728 = Bundle(cluster=w1177, "STATUS"="STOP") -> (w1175:T4)  [unwired: 2 in]
                        n729 = local write "DISP LAB05-1"(w1175) -> ()
                      }
                    }
                  }
                  frame True {
                    # "start new test and create test file"
                    n730 = stacked-sequence {
                      seq-local: [w1189 _ _ _ _] -> [_ w1214 _ _ _]
                      tunnel: w1188 -> [w1194 _ _ _ _]
                      tunnel: w1187 -> [w1190 _ _ _ _]
                      tunnel: w1186 -> [w1204 _ _ _ _]
                      tunnel: w1185 -> [w1197 _ _ _ _]
                      tunnel: w1184 -> [w1192 _ _ _ _]
                      tunnel: [_ w1208 _ _ _] -> w1183
                      frame #0 {
                        w1191 = "\\"
                        n731 = local read "SET LAB05-1"() -> (w1199:T5)
                        n732 = case shown="\"CHART TEST\", Default" w1204 {
                          tunnel: ["CHART TEST-" "CYCLE TEST-" "T-RISE TEST-"] -> w1200
                          frame "CHART TEST", Default {
                          }
                          frame "CYCLE TEST" {
                          }
                          frame "T-RISE TEST" {
                          }
                        }
                        n733 = Unbundle(w1199) -> ("DESCRIPTION"=w1198:string)  [unwired: 4 out]
                        n734 = Concatenate Strings(w1194, "LAB05-1\\", w1192, w1191, w1190, w1191) -> (w1201:string)
                        n735 = String To Path(string=w1201) -> (path=w1203:path)
                        n736 = Concatenate Strings(w1201, w1200, w1198, "-", w1197, ".tdms") -> (w1189:string)
                        n737 = Create Folder(path (use dialog)=w1203) -> (error out=w1202:errorcluster)  [unwired: 2 in, 2 out]
                        n738 = global write "Global 1.vi" "LAB05-1 FILE"(w1189) -> ()
                        n739 = call <vilib>:"Clear Errors.vi"("error in (no error)"=w1202) -> ()  [unwired: 6 in, 1 out]
                      }
                      frame #1 {
                        n740 = String To Path(string=w1214) -> (path=w1209:path)
                        n741 = TDMS Open(5:FALSE, 6:FALSE, 10:T15."create or replace" ("operation (0:open)"), 11:w1209) -> (0:w1208:errorcluster, 3:→"TDMS LAB05-1":refnum<k34>)  [unwired: 3 in]
                      }
                      frame #2 {
                        n742 = local read "SET LAB05-1"() -> (w1220:T5)
                        n743 = local read "TDMS LAB05-1"() -> (w1231:refnum<k34>)
                        n744 = Build Array("Testers Name", "Description", "Set Test Cycles", "T-Rise minutes", "T-Rise Deg C") -> (w1221:string[])
                        n745 = Unbundle(w1220) -> ("NAME"=w1219:string, "DESCRIPTION"=w1218:string, "CYCLES"=w1217:dbl, "T-RISE mins"=w1216:dbl, "T-RISE deg C"=w1215:dbl)
                        n746 = Number To Decimal String(number=w1217) -> (decimal integer string=w1230:string)  [unwired: 1 in]
                        n747 = Number To Decimal String(number=w1216) -> (decimal integer string=w1229:string)  [unwired: 1 in]
                        n748 = Number To Decimal String(number=w1215) -> (decimal integer string=w1228:string)  [unwired: 1 in]
                        n749 = Build Array(w1219, w1218, w1230, w1229, w1228) -> (w1227:string[])
                        n750 = TDMS Set Properties(5:w1227, 7:w1221, 11:w1231) -> ()  [unwired: 3 in, 4 out]
                      }
                      frame #3 {
                        w1233 = 0.0
                        n751 = local read "DISP LAB05-1"() -> (w1235:T4)
                        n752 = Bundle(cluster=w1235, "CYCLE"=w1233, "MINS"=w1233, "STATUS"="RUN") -> (w1234:T4)
                        n753 = local write "DISP LAB05-1"(w1234) -> ()
                      }
                      frame #4 {
                        n754 = local read "SIG LAB05-1"() -> (w1238:T2)
                        n755 = local read "TEMP START LAB05-1"() -> (w1240:cluster{"TL":dbl, "TN":dbl})
                        n756 = Unbundle(w1238) -> ("Tmp Live"=w1237:dbl, "Tmp Neut"=w1236:dbl)  [unwired: 3 out]
                        n757 = Bundle(cluster=w1240, "TL"=w1237, "TN"=w1236) -> (w1239:cluster{"TL":dbl, "TN":dbl})
                        n758 = local write "TEMP START LAB05-1"(w1239) -> ()
                      }
                    }
                  }
                }
              }
              event "RUN LAB05-2": Value Change {
                n759 = event-data() -> ("NewVal"=w1241:bool)  [unwired: 1 in, 5 out]
                n760 = local write "run lab05-2"(w1241) -> ()
                n761 = case shown="False" w1241 {
                  tunnel: w1247 -> [_ w1280]
                  tunnel: w1246 -> [_ w1279]
                  tunnel: w1244 -> [w1249 w1278]
                  tunnel: w1245 -> [_ w1277]
                  tunnel: w1243 -> [_ w1276]
                  tunnel: [w1248 w1275] -> w1242
                  frame False {
                    # "stop test"
                    n762 = stacked-sequence {
                      tunnel: w1249 -> [w1258 _]
                      tunnel: [w1250 _] -> w1248
                      frame #0 {
                        n763 = local read "DISP LAB05-2"() -> (w1257:T4)
                        n764 = Unbundle(w1257) -> ("CYCLE"=w1255:dbl, "MINS"=w1256:dbl)  [unwired: 1 out]
                        n765 = case shown="\"CYCLE TEST\"" w1258 {
                          tunnel: w1256 -> [_ _ w1265]
                          tunnel: w1255 -> [w1263 w1264 _]
                          tunnel: [w1263 w1264 w1265] -> w1254
                          frame "CHART TEST", Default {
                          }
                          frame "CYCLE TEST" {
                          }
                          frame "T-RISE TEST" {
                          }
                        }
                        n766 = local read "TDMS LAB05-2"() -> (w1262:refnum<k34>)
                        n767 = Build Array("STOPPED") -> (w1259:string[])
                        n768 = Build Array(w1254) -> (w1253:dbl[])
                        n769 = TDMS Write(0:w1262, 5:"TEST RESULT", 7:w1259, 9:w1253) -> (4:w1251:refnum<k34>, 15:w1252:errorcluster)  [unwired: 2 in, 2 out]
                        n770 = TDMS Close(8:w1252, 11:w1251) -> (0:w1250:errorcluster)  [unwired: 1 out]
                      }
                      frame #1 {
                        n771 = local read "DISP LAB05-2"() -> (w1269:T4)
                        n772 = stacked-sequence {
                          tunnel: "LAB05-2" -> [w1271 w1273]
                          frame #0 {
                            n773 = call "sub vi - defrag tdms v1.vi"("panel id"=w1271) -> ("error out"=w1270:errorcluster)  [unwired: 10 in]
                            n774 = local write "data file error"(w1270) -> ()
                          }
                          frame #1 {
                            n775 = local write "RESULT LAB05-2"(FALSE) -> ()
                            n776 = call "Save data file to network drive v1.vi"("panel id"=w1273) -> ("network file save error"=w1272:errorcluster)  [unwired: 9 in, 1 out]
                            n777 = local write "data file error"(w1272) -> ()
                          }
                        }
                        n778 = Bundle(cluster=w1269, "STATUS"="STOP") -> (w1267:T4)  [unwired: 2 in]
                        n779 = local write "DISP LAB05-2"(w1267) -> ()
                      }
                    }
                  }
                  frame True {
                    # "start new test and create test file"
                    n780 = stacked-sequence {
                      seq-local: [w1281 _ _ _ _] -> [_ w1306 _ _ _]
                      tunnel: w1280 -> [w1286 _ _ _ _]
                      tunnel: w1279 -> [w1282 _ _ _ _]
                      tunnel: w1278 -> [w1296 _ _ _ _]
                      tunnel: w1277 -> [w1289 _ _ _ _]
                      tunnel: w1276 -> [w1284 _ _ _ _]
                      tunnel: [_ w1300 _ _ _] -> w1275
                      frame #0 {
                        w1283 = "\\"
                        n781 = local read "SET LAB05-2"() -> (w1291:T5)
                        n782 = case shown="\"CHART TEST\", Default" w1296 {
                          tunnel: ["CHART TEST-" "CYCLE TEST-" "T-RISE TEST-"] -> w1292
                          frame "CHART TEST", Default {
                          }
                          frame "CYCLE TEST" {
                          }
                          frame "T-RISE TEST" {
                          }
                        }
                        n783 = Unbundle(w1291) -> ("DESCRIPTION"=w1290:string)  [unwired: 4 out]
                        n784 = Concatenate Strings(w1286, "LAB05-2\\", w1284, w1283, w1282, w1283) -> (w1293:string)
                        n785 = String To Path(string=w1293) -> (path=w1295:path)
                        n786 = Concatenate Strings(w1293, w1292, w1290, "-", w1289, ".tdms") -> (w1281:string)
                        n787 = Create Folder(path (use dialog)=w1295) -> (error out=w1294:errorcluster)  [unwired: 2 in, 2 out]
                        n788 = global write "Global 1.vi" "LAB05-2 FILE"(w1281) -> ()
                        n789 = call <vilib>:"Clear Errors.vi"("error in (no error)"=w1294) -> ()  [unwired: 6 in, 1 out]
                      }
                      frame #1 {
                        n790 = String To Path(string=w1306) -> (path=w1301:path)
                        n791 = TDMS Open(5:FALSE, 6:FALSE, 10:T15."create or replace" ("operation (0:open)"), 11:w1301) -> (0:w1300:errorcluster, 3:→"TDMS LAB05-2":refnum<k34>)  [unwired: 3 in]
                      }
                      frame #2 {
                        n792 = local read "SET LAB05-2"() -> (w1312:T5)
                        n793 = local read "TDMS LAB05-2"() -> (w1323:refnum<k34>)
                        n794 = Build Array("Testers Name", "Description", "Set Test Cycles", "T-Rise minutes", "T-Rise Deg C") -> (w1313:string[])
                        n795 = Unbundle(w1312) -> ("NAME"=w1311:string, "DESCRIPTION"=w1310:string, "CYCLES"=w1309:dbl, "T-RISE mins"=w1308:dbl, "T-RISE deg C"=w1307:dbl)
                        n796 = Number To Decimal String(number=w1309) -> (decimal integer string=w1322:string)  [unwired: 1 in]
                        n797 = Number To Decimal String(number=w1308) -> (decimal integer string=w1321:string)  [unwired: 1 in]
                        n798 = Number To Decimal String(number=w1307) -> (decimal integer string=w1320:string)  [unwired: 1 in]
                        n799 = Build Array(w1311, w1310, w1322, w1321, w1320) -> (w1319:string[])
                        n800 = TDMS Set Properties(5:w1319, 7:w1313, 11:w1323) -> ()  [unwired: 3 in, 4 out]
                      }
                      frame #3 {
                        w1325 = 0.0
                        n801 = local read "DISP LAB05-2"() -> (w1327:T4)
                        n802 = Bundle(cluster=w1327, "CYCLE"=w1325, "MINS"=w1325, "STATUS"="RUN") -> (w1326:T4)
                        n803 = local write "DISP LAB05-2"(w1326) -> ()
                      }
                      frame #4 {
                        n804 = local read "SIG LAB05-2"() -> (w1330:T2)
                        n805 = local read "TEMP START LAB05-2"() -> (w1332:cluster{"TL":dbl, "TN":dbl})
                        n806 = Unbundle(w1330) -> ("Tmp Live"=w1329:dbl, "Tmp Neut"=w1328:dbl)  [unwired: 3 out]
                        n807 = Bundle(cluster=w1332, "TL"=w1329, "TN"=w1328) -> (w1331:cluster{"TL":dbl, "TN":dbl})
                        n808 = local write "TEMP START LAB05-2"(w1331) -> ()
                      }
                    }
                  }
                }
              }
            }
            n809 = local write "data file error"(w384) -> ()
          }
          frame #4 {
            # "check if test cycles reached for cycle tests, if so then test pass"
            n810 = stacked-sequence {
              tunnel: w1352 -> [_ _ _ _ _ _ _ _ _ _]
              tunnel: w1351 -> [_ _ _ _ _ _ _ _ _ _]
              tunnel: w1350 -> [_ _ _ _ _ _ _ _ _ _]
              tunnel: w1349 -> [_ _ _ _ _ _ _ _ _ _]
              tunnel: w1348 -> [_ _ _ _ _ _ _ _ _ _]
              tunnel: w1347 -> [_ _ _ _ _ _ _ _ _ _]
              tunnel: w1346 -> [_ _ _ _ _ _ _ _ _ _]
              tunnel: w1345 -> [_ _ _ _ _ _ _ _ _ _]
              tunnel: w1344 -> [_ _ _ _ _ _ _ _ _ _]
              tunnel: w1343 -> [_ _ _ _ _ _ _ _ _ _]
              tunnel: w1342 -> [w1357 _ _ _ _ _ _ _ _ _]
              tunnel: w1341 -> [_ w1392 _ _ _ _ _ _ _ _]
              tunnel: w1340 -> [_ _ w1431 _ _ _ _ _ _ _]
              tunnel: w1339 -> [_ _ _ w1470 _ _ _ _ _ _]
              tunnel: w1338 -> [_ _ _ _ w1509 _ _ _ _ _]
              tunnel: w1337 -> [_ _ _ _ _ w1548 _ _ _ _]
              tunnel: w1336 -> [_ _ _ _ _ _ w1587 _ _ _]
              tunnel: w1335 -> [_ _ _ _ _ _ _ w1626 _ _]
              tunnel: w1334 -> [_ _ _ _ _ _ _ _ w1665 _]
              tunnel: w1333 -> [_ _ _ _ _ _ _ _ _ w1704]
              frame #0 {
                # "LAB01-1"
                n811 = Less?(x=w1357, y=2) -> (x < y?=w1355:bool)
                n812 = local read "DISP LAB01-1"() -> (w1358:T4)
                n813 = Unbundle(w1358) -> ("STATUS"=w1359:string)  [unwired: 2 out]
                n814 = Equal?(x=w1359, y="RUN") -> (x = y?=w1354:bool)
                n815 = And(x=w1354, y=w1355) -> (x .and. y?=w1353:bool)
                n816 = case shown="True" w1353 {
                  tunnel: w1358 -> [_ w1362]
                  tunnel: w1357 -> [_ w1367]
                  frame False {
                  }
                  frame True {
                    n817 = local read "SET LAB01-1"() -> (w1369:T5)
                    n818 = local read "TDMS LAB01-1"() -> (w1361:refnum<k34>)
                    n819 = Unbundle(w1362) -> ("CYCLE"=w1368:dbl)  [unwired: 2 out]
                    n820 = Unbundle(w1369) -> ("CYCLES"=w1364:dbl, "T-RISE mins"=w1366:dbl)  [unwired: 3 out]
                    n821 = case shown="\"CYCLE TEST\"" w1367 {
                      tunnel: w1366 -> [_ _ w1376]
                      tunnel: [w1371 w1373 w1376] -> w1365
                      tunnel: w1364 -> [w1371 w1373 _]
                      tunnel: ["CHART PASS" "CYCLE PASS" "T-RISE PASS"] -> w1363
                      frame "CHART TEST", Default {
                      }
                      frame "CYCLE TEST" {
                      }
                      frame "T-RISE TEST" {
                      }
                    }
                    n822 = Greater Or Equal?(x=w1368, y=w1364) -> (x >= y?=w1370:bool)
                    n823 = case shown="True" w1370 {
                      tunnel: w1365 -> [w1380 _]
                      tunnel: w1363 -> [w1379 _]
                      tunnel: w1362 -> [w1378 _]
                      tunnel: w1361 -> [w1377 _]
                      frame True {
                        n824 = stacked-sequence {
                          tunnel: w1380 -> [w1384 _]
                          tunnel: w1379 -> [w1382 w1388]
                          tunnel: w1378 -> [_ w1391]
                          tunnel: w1377 -> [w1381 _]
                          frame #0 {
                            n825 = Build Array(w1382) -> (w1385:string[])
                            n826 = Build Array(w1384) -> (w1383:dbl[])
                            n827 = TDMS Write(0:w1381, 5:"TEST PASS", 7:w1385, 9:w1383) -> (15:w1387:errorcluster)  [unwired: 2 in, 3 out]
                            n828 = local write "data file error"(w1387) -> ()
                          }
                          frame #1 {
                            n829 = Bundle(cluster=w1391, "STATUS"=w1388) -> (w1389:T4)  [unwired: 2 in]
                            n830 = local write "RESULT LAB01-1"(TRUE) -> ()
                            n831 = local write "DISP LAB01-1"(w1389) -> ()
                          }
                        }
                      }
                      frame False {
                      }
                    }
                  }
                }
              }
              frame #1 {
                # "LAB01-2"
                n832 = Less?(x=w1392, y=2) -> (x < y?=w1395:bool)
                n833 = local read "DISP LAB01-2"() -> (w1397:T4)
                n834 = Unbundle(w1397) -> ("STATUS"=w1398:string)  [unwired: 2 out]
                n835 = Equal?(x=w1398, y="RUN") -> (x = y?=w1394:bool)
                n836 = And(x=w1394, y=w1395) -> (x .and. y?=w1393:bool)
                n837 = case shown="True" w1393 {
                  tunnel: w1397 -> [_ w1401]
                  tunnel: w1392 -> [_ w1406]
                  frame False {
                  }
                  frame True {
                    n838 = local read "SET LAB01-2"() -> (w1408:T5)
                    n839 = local read "TDMS LAB01-2"() -> (w1400:refnum<k34>)
                    n840 = Unbundle(w1401) -> ("CYCLE"=w1407:dbl)  [unwired: 2 out]
                    n841 = Unbundle(w1408) -> ("CYCLES"=w1403:dbl, "T-RISE mins"=w1405:dbl)  [unwired: 3 out]
                    n842 = case shown="\"T-RISE TEST\"" w1406 {
                      tunnel: w1405 -> [_ _ w1415]
                      tunnel: [w1410 w1412 w1415] -> w1404
                      tunnel: w1403 -> [w1410 w1412 _]
                      tunnel: ["CHART PASS" "CYCLE PASS" "T-RISE PASS"] -> w1402
                      frame "CHART TEST", Default {
                      }
                      frame "CYCLE TEST" {
                      }
                      frame "T-RISE TEST" {
                      }
                    }
                    n843 = Greater Or Equal?(x=w1407, y=w1403) -> (x >= y?=w1409:bool)
                    n844 = case shown="True" w1409 {
                      tunnel: w1404 -> [w1419 _]
                      tunnel: w1402 -> [w1418 _]
                      tunnel: w1401 -> [w1417 _]
                      tunnel: w1400 -> [w1416 _]
                      frame True {
                        n845 = stacked-sequence {
                          tunnel: w1419 -> [w1423 _]
                          tunnel: w1418 -> [w1421 w1427]
                          tunnel: w1417 -> [_ w1430]
                          tunnel: w1416 -> [w1420 _]
                          frame #0 {
                            n846 = Build Array(w1421) -> (w1424:string[])
                            n847 = Build Array(w1423) -> (w1422:dbl[])
                            n848 = TDMS Write(0:w1420, 5:"TEST PASS", 7:w1424, 9:w1422) -> (15:w1426:errorcluster)  [unwired: 2 in, 3 out]
                            n849 = local write "data file error"(w1426) -> ()
                          }
                          frame #1 {
                            n850 = Bundle(cluster=w1430, "STATUS"=w1427) -> (w1428:T4)  [unwired: 2 in]
                            n851 = local write "RESULT LAB01-2"(TRUE) -> ()
                            n852 = local write "DISP LAB01-2"(w1428) -> ()
                          }
                        }
                      }
                      frame False {
                      }
                    }
                  }
                }
              }
              frame #2 {
                # "LAB02-1"
                n853 = Less?(x=w1431, y=2) -> (x < y?=w1434:bool)
                n854 = local read "DISP LAB02-1"() -> (w1436:T4)
                n855 = Unbundle(w1436) -> ("STATUS"=w1437:string)  [unwired: 2 out]
                n856 = Equal?(x=w1437, y="RUN") -> (x = y?=w1433:bool)
                n857 = And(x=w1433, y=w1434) -> (x .and. y?=w1432:bool)
                n858 = case shown="True" w1432 {
                  tunnel: w1436 -> [_ w1440]
                  tunnel: w1431 -> [_ w1445]
                  frame False {
                  }
                  frame True {
                    n859 = local read "SET LAB02-1"() -> (w1447:T5)
                    n860 = local read "TDMS LAB02-1"() -> (w1439:refnum<k34>)
                    n861 = Unbundle(w1440) -> ("CYCLE"=w1446:dbl)  [unwired: 2 out]
                    n862 = Unbundle(w1447) -> ("CYCLES"=w1442:dbl, "T-RISE mins"=w1444:dbl)  [unwired: 3 out]
                    n863 = case shown="\"T-RISE TEST\"" w1445 {
                      tunnel: w1444 -> [_ _ w1454]
                      tunnel: [w1449 w1451 w1454] -> w1443
                      tunnel: w1442 -> [w1449 w1451 _]
                      tunnel: ["CHART PASS" "CYCLE PASS" "T-RISE PASS"] -> w1441
                      frame "CHART TEST", Default {
                      }
                      frame "CYCLE TEST" {
                      }
                      frame "T-RISE TEST" {
                      }
                    }
                    n864 = Greater Or Equal?(x=w1446, y=w1442) -> (x >= y?=w1448:bool)
                    n865 = case shown="True" w1448 {
                      tunnel: w1443 -> [w1458 _]
                      tunnel: w1441 -> [w1457 _]
                      tunnel: w1440 -> [w1456 _]
                      tunnel: w1439 -> [w1455 _]
                      frame True {
                        n866 = stacked-sequence {
                          tunnel: w1458 -> [w1462 _]
                          tunnel: w1457 -> [w1460 w1466]
                          tunnel: w1456 -> [_ w1469]
                          tunnel: w1455 -> [w1459 _]
                          frame #0 {
                            n867 = Build Array(w1460) -> (w1463:string[])
                            n868 = Build Array(w1462) -> (w1461:dbl[])
                            n869 = TDMS Write(0:w1459, 5:"TEST PASS", 7:w1463, 9:w1461) -> (15:w1465:errorcluster)  [unwired: 2 in, 3 out]
                            n870 = local write "data file error"(w1465) -> ()
                          }
                          frame #1 {
                            n871 = Bundle(cluster=w1469, "STATUS"=w1466) -> (w1467:T4)  [unwired: 2 in]
                            n872 = local write "RESULT LAB02-1"(TRUE) -> ()
                            n873 = local write "DISP LAB02-1"(w1467) -> ()
                          }
                        }
                      }
                      frame False {
                      }
                    }
                  }
                }
              }
              frame #3 {
                # "LAB02-2"
                n874 = Less?(x=w1470, y=2) -> (x < y?=w1473:bool)
                n875 = local read "DISP LAB02-2"() -> (w1475:T4)
                n876 = Unbundle(w1475) -> ("STATUS"=w1476:string)  [unwired: 2 out]
                n877 = Equal?(x=w1476, y="RUN") -> (x = y?=w1472:bool)
                n878 = And(x=w1472, y=w1473) -> (x .and. y?=w1471:bool)
                n879 = case shown="True" w1471 {
                  tunnel: w1475 -> [_ w1479]
                  tunnel: w1470 -> [_ w1484]
                  frame False {
                  }
                  frame True {
                    n880 = local read "SET LAB02-2"() -> (w1486:T5)
                    n881 = local read "TDMS LAB02-2"() -> (w1478:refnum<k34>)
                    n882 = Unbundle(w1479) -> ("CYCLE"=w1485:dbl)  [unwired: 2 out]
                    n883 = Unbundle(w1486) -> ("CYCLES"=w1481:dbl, "T-RISE mins"=w1483:dbl)  [unwired: 3 out]
                    n884 = case shown="\"T-RISE TEST\"" w1484 {
                      tunnel: w1483 -> [_ _ w1493]
                      tunnel: [w1488 w1490 w1493] -> w1482
                      tunnel: w1481 -> [w1488 w1490 _]
                      tunnel: ["CHART PASS" "CYCLE PASS" "T-RISE PASS"] -> w1480
                      frame "CHART TEST", Default {
                      }
                      frame "CYCLE TEST" {
                      }
                      frame "T-RISE TEST" {
                      }
                    }
                    n885 = Greater Or Equal?(x=w1485, y=w1481) -> (x >= y?=w1487:bool)
                    n886 = case shown="True" w1487 {
                      tunnel: w1482 -> [w1497 _]
                      tunnel: w1480 -> [w1496 _]
                      tunnel: w1479 -> [w1495 _]
                      tunnel: w1478 -> [w1494 _]
                      frame True {
                        n887 = stacked-sequence {
                          tunnel: w1497 -> [w1501 _]
                          tunnel: w1496 -> [w1499 w1505]
                          tunnel: w1495 -> [_ w1508]
                          tunnel: w1494 -> [w1498 _]
                          frame #0 {
                            n888 = Build Array(w1499) -> (w1502:string[])
                            n889 = Build Array(w1501) -> (w1500:dbl[])
                            n890 = TDMS Write(0:w1498, 5:"TEST PASS", 7:w1502, 9:w1500) -> (15:w1504:errorcluster)  [unwired: 2 in, 3 out]
                            n891 = local write "data file error"(w1504) -> ()
                          }
                          frame #1 {
                            n892 = Bundle(cluster=w1508, "STATUS"=w1505) -> (w1506:T4)  [unwired: 2 in]
                            n893 = local write "RESULT LAB02-2"(TRUE) -> ()
                            n894 = local write "DISP LAB02-2"(w1506) -> ()
                          }
                        }
                      }
                      frame False {
                      }
                    }
                  }
                }
              }
              frame #4 {
                # "LAB03-1"
                n895 = Less?(x=w1509, y=2) -> (x < y?=w1512:bool)
                n896 = local read "DISP LAB03-1"() -> (w1514:T4)
                n897 = Unbundle(w1514) -> ("STATUS"=w1515:string)  [unwired: 2 out]
                n898 = Equal?(x=w1515, y="RUN") -> (x = y?=w1511:bool)
                n899 = And(x=w1511, y=w1512) -> (x .and. y?=w1510:bool)
                n900 = case shown="True" w1510 {
                  tunnel: w1514 -> [_ w1518]
                  tunnel: w1509 -> [_ w1523]
                  frame False {
                  }
                  frame True {
                    n901 = local read "SET LAB03-1"() -> (w1525:T5)
                    n902 = local read "TDMS LAB03-1"() -> (w1517:refnum<k34>)
                    n903 = Unbundle(w1518) -> ("CYCLE"=w1524:dbl)  [unwired: 2 out]
                    n904 = Unbundle(w1525) -> ("CYCLES"=w1520:dbl, "T-RISE mins"=w1522:dbl)  [unwired: 3 out]
                    n905 = case shown="\"T-RISE TEST\"" w1523 {
                      tunnel: w1522 -> [_ _ w1532]
                      tunnel: [w1527 w1529 w1532] -> w1521
                      tunnel: w1520 -> [w1527 w1529 _]
                      tunnel: ["CHART PASS" "CYCLE PASS" "T-RISE PASS"] -> w1519
                      frame "CHART TEST", Default {
                      }
                      frame "CYCLE TEST" {
                      }
                      frame "T-RISE TEST" {
                      }
                    }
                    n906 = Greater Or Equal?(x=w1524, y=w1520) -> (x >= y?=w1526:bool)
                    n907 = case shown="True" w1526 {
                      tunnel: w1521 -> [w1536 _]
                      tunnel: w1519 -> [w1535 _]
                      tunnel: w1518 -> [w1534 _]
                      tunnel: w1517 -> [w1533 _]
                      frame True {
                        n908 = stacked-sequence {
                          tunnel: w1536 -> [w1540 _]
                          tunnel: w1535 -> [w1538 w1544]
                          tunnel: w1534 -> [_ w1547]
                          tunnel: w1533 -> [w1537 _]
                          frame #0 {
                            n909 = Build Array(w1538) -> (w1541:string[])
                            n910 = Build Array(w1540) -> (w1539:dbl[])
                            n911 = TDMS Write(0:w1537, 5:"TEST PASS", 7:w1541, 9:w1539) -> (15:w1543:errorcluster)  [unwired: 2 in, 3 out]
                            n912 = local write "data file error"(w1543) -> ()
                          }
                          frame #1 {
                            n913 = Bundle(cluster=w1547, "STATUS"=w1544) -> (w1545:T4)  [unwired: 2 in]
                            n914 = local write "RESULT LAB03-1"(TRUE) -> ()
                            n915 = local write "DISP LAB03-1"(w1545) -> ()
                          }
                        }
                      }
                      frame False {
                      }
                    }
                  }
                }
              }
              frame #5 {
                # "LAB03-2"
                n916 = Less?(x=w1548, y=2) -> (x < y?=w1551:bool)
                n917 = local read "DISP LAB03-2"() -> (w1553:T4)
                n918 = Unbundle(w1553) -> ("STATUS"=w1554:string)  [unwired: 2 out]
                n919 = Equal?(x=w1554, y="RUN") -> (x = y?=w1550:bool)
                n920 = And(x=w1550, y=w1551) -> (x .and. y?=w1549:bool)
                n921 = case shown="True" w1549 {
                  tunnel: w1553 -> [_ w1557]
                  tunnel: w1548 -> [_ w1562]
                  frame False {
                  }
                  frame True {
                    n922 = local read "SET LAB03-2"() -> (w1564:T5)
                    n923 = local read "TDMS LAB03-2"() -> (w1556:refnum<k34>)
                    n924 = Unbundle(w1557) -> ("CYCLE"=w1563:dbl)  [unwired: 2 out]
                    n925 = Unbundle(w1564) -> ("CYCLES"=w1559:dbl, "T-RISE mins"=w1561:dbl)  [unwired: 3 out]
                    n926 = case shown="\"T-RISE TEST\"" w1562 {
                      tunnel: w1561 -> [_ _ w1571]
                      tunnel: [w1566 w1568 w1571] -> w1560
                      tunnel: w1559 -> [w1566 w1568 _]
                      tunnel: ["CHART PASS" "CYCLE PASS" "T-RISE PASS"] -> w1558
                      frame "CHART TEST", Default {
                      }
                      frame "CYCLE TEST" {
                      }
                      frame "T-RISE TEST" {
                      }
                    }
                    n927 = Greater Or Equal?(x=w1563, y=w1559) -> (x >= y?=w1565:bool)
                    n928 = case shown="True" w1565 {
                      tunnel: w1560 -> [w1575 _]
                      tunnel: w1558 -> [w1574 _]
                      tunnel: w1557 -> [w1573 _]
                      tunnel: w1556 -> [w1572 _]
                      frame True {
                        n929 = stacked-sequence {
                          tunnel: w1575 -> [w1579 _]
                          tunnel: w1574 -> [w1577 w1583]
                          tunnel: w1573 -> [_ w1586]
                          tunnel: w1572 -> [w1576 _]
                          frame #0 {
                            n930 = Build Array(w1577) -> (w1580:string[])
                            n931 = Build Array(w1579) -> (w1578:dbl[])
                            n932 = TDMS Write(0:w1576, 5:"TEST PASS", 7:w1580, 9:w1578) -> (15:w1582:errorcluster)  [unwired: 2 in, 3 out]
                            n933 = local write "data file error"(w1582) -> ()
                          }
                          frame #1 {
                            n934 = Bundle(cluster=w1586, "STATUS"=w1583) -> (w1584:T4)  [unwired: 2 in]
                            n935 = local write "RESULT LAB03-2"(TRUE) -> ()
                            n936 = local write "DISP LAB03-2"(w1584) -> ()
                          }
                        }
                      }
                      frame False {
                      }
                    }
                  }
                }
              }
              frame #6 {
                # "LAB04-1"
                n937 = Less?(x=w1587, y=2) -> (x < y?=w1590:bool)
                n938 = local read "DISP LAB04-1"() -> (w1592:T4)
                n939 = Unbundle(w1592) -> ("STATUS"=w1593:string)  [unwired: 2 out]
                n940 = Equal?(x=w1593, y="RUN") -> (x = y?=w1589:bool)
                n941 = And(x=w1589, y=w1590) -> (x .and. y?=w1588:bool)
                n942 = case shown="True" w1588 {
                  tunnel: w1592 -> [_ w1596]
                  tunnel: w1587 -> [_ w1601]
                  frame False {
                  }
                  frame True {
                    n943 = local read "SET LAB04-1"() -> (w1603:T5)
                    n944 = local read "TDMS LAB04-1"() -> (w1595:refnum<k34>)
                    n945 = Unbundle(w1596) -> ("CYCLE"=w1602:dbl)  [unwired: 2 out]
                    n946 = Unbundle(w1603) -> ("CYCLES"=w1598:dbl, "T-RISE mins"=w1600:dbl)  [unwired: 3 out]
                    n947 = case shown="\"T-RISE TEST\"" w1601 {
                      tunnel: w1600 -> [_ _ w1610]
                      tunnel: [w1605 w1607 w1610] -> w1599
                      tunnel: w1598 -> [w1605 w1607 _]
                      tunnel: ["CHART PASS" "CYCLE PASS" "T-RISE PASS"] -> w1597
                      frame "CHART TEST", Default {
                      }
                      frame "CYCLE TEST" {
                      }
                      frame "T-RISE TEST" {
                      }
                    }
                    n948 = Greater Or Equal?(x=w1602, y=w1598) -> (x >= y?=w1604:bool)
                    n949 = case shown="True" w1604 {
                      tunnel: w1599 -> [w1614 _]
                      tunnel: w1597 -> [w1613 _]
                      tunnel: w1596 -> [w1612 _]
                      tunnel: w1595 -> [w1611 _]
                      frame True {
                        n950 = stacked-sequence {
                          tunnel: w1614 -> [w1618 _]
                          tunnel: w1613 -> [w1616 w1622]
                          tunnel: w1612 -> [_ w1625]
                          tunnel: w1611 -> [w1615 _]
                          frame #0 {
                            n951 = Build Array(w1616) -> (w1619:string[])
                            n952 = Build Array(w1618) -> (w1617:dbl[])
                            n953 = TDMS Write(0:w1615, 5:"TEST PASS", 7:w1619, 9:w1617) -> (15:w1621:errorcluster)  [unwired: 2 in, 3 out]
                            n954 = local write "data file error"(w1621) -> ()
                          }
                          frame #1 {
                            n955 = Bundle(cluster=w1625, "STATUS"=w1622) -> (w1623:T4)  [unwired: 2 in]
                            n956 = local write "RESULT LAB04-1"(TRUE) -> ()
                            n957 = local write "DISP LAB04-1"(w1623) -> ()
                          }
                        }
                      }
                      frame False {
                      }
                    }
                  }
                }
              }
              frame #7 {
                # "LAB04-2"
                n958 = Less?(x=w1626, y=2) -> (x < y?=w1629:bool)
                n959 = local read "DISP LAB04-2"() -> (w1631:T4)
                n960 = Unbundle(w1631) -> ("STATUS"=w1632:string)  [unwired: 2 out]
                n961 = Equal?(x=w1632, y="RUN") -> (x = y?=w1628:bool)
                n962 = And(x=w1628, y=w1629) -> (x .and. y?=w1627:bool)
                n963 = case shown="True" w1627 {
                  tunnel: w1631 -> [_ w1635]
                  tunnel: w1626 -> [_ w1640]
                  frame False {
                  }
                  frame True {
                    n964 = local read "SET LAB04-2"() -> (w1642:T5)
                    n965 = local read "TDMS LAB04-2"() -> (w1634:refnum<k34>)
                    n966 = Unbundle(w1635) -> ("CYCLE"=w1641:dbl)  [unwired: 2 out]
                    n967 = Unbundle(w1642) -> ("CYCLES"=w1637:dbl, "T-RISE mins"=w1639:dbl)  [unwired: 3 out]
                    n968 = case shown="\"T-RISE TEST\"" w1640 {
                      tunnel: w1639 -> [_ _ w1649]
                      tunnel: [w1644 w1646 w1649] -> w1638
                      tunnel: w1637 -> [w1644 w1646 _]
                      tunnel: ["CHART PASS" "CYCLE PASS" "T-RISE PASS"] -> w1636
                      frame "CHART TEST", Default {
                      }
                      frame "CYCLE TEST" {
                      }
                      frame "T-RISE TEST" {
                      }
                    }
                    n969 = Greater Or Equal?(x=w1641, y=w1637) -> (x >= y?=w1643:bool)
                    n970 = case shown="True" w1643 {
                      tunnel: w1638 -> [w1653 _]
                      tunnel: w1636 -> [w1652 _]
                      tunnel: w1635 -> [w1651 _]
                      tunnel: w1634 -> [w1650 _]
                      frame True {
                        n971 = stacked-sequence {
                          tunnel: w1653 -> [w1657 _]
                          tunnel: w1652 -> [w1655 w1661]
                          tunnel: w1651 -> [_ w1664]
                          tunnel: w1650 -> [w1654 _]
                          frame #0 {
                            n972 = Build Array(w1655) -> (w1658:string[])
                            n973 = Build Array(w1657) -> (w1656:dbl[])
                            n974 = TDMS Write(0:w1654, 5:"TEST PASS", 7:w1658, 9:w1656) -> (15:w1660:errorcluster)  [unwired: 2 in, 3 out]
                            n975 = local write "data file error"(w1660) -> ()
                          }
                          frame #1 {
                            n976 = Bundle(cluster=w1664, "STATUS"=w1661) -> (w1662:T4)  [unwired: 2 in]
                            n977 = local write "RESULT LAB04-2"(TRUE) -> ()
                            n978 = local write "DISP LAB04-2"(w1662) -> ()
                          }
                        }
                      }
                      frame False {
                      }
                    }
                  }
                }
              }
              frame #8 {
                # "LAB05-1"
                n979 = Less?(x=w1665, y=2) -> (x < y?=w1668:bool)
                n980 = local read "DISP LAB05-1"() -> (w1670:T4)
                n981 = Unbundle(w1670) -> ("STATUS"=w1671:string)  [unwired: 2 out]
                n982 = Equal?(x=w1671, y="RUN") -> (x = y?=w1667:bool)
                n983 = And(x=w1667, y=w1668) -> (x .and. y?=w1666:bool)
                n984 = case shown="True" w1666 {
                  tunnel: w1670 -> [_ w1674]
                  tunnel: w1665 -> [_ w1679]
                  frame False {
                  }
                  frame True {
                    n985 = local read "SET LAB05-1"() -> (w1681:T5)
                    n986 = local read "TDMS LAB05-1"() -> (w1673:refnum<k34>)
                    n987 = Unbundle(w1674) -> ("CYCLE"=w1680:dbl)  [unwired: 2 out]
                    n988 = Unbundle(w1681) -> ("CYCLES"=w1676:dbl, "T-RISE mins"=w1678:dbl)  [unwired: 3 out]
                    n989 = case shown="\"T-RISE TEST\"" w1679 {
                      tunnel: w1678 -> [_ _ w1688]
                      tunnel: [w1683 w1685 w1688] -> w1677
                      tunnel: w1676 -> [w1683 w1685 _]
                      tunnel: ["CHART PASS" "CYCLE PASS" "T-RISE PASS"] -> w1675
                      frame "CHART TEST", Default {
                      }
                      frame "CYCLE TEST" {
                      }
                      frame "T-RISE TEST" {
                      }
                    }
                    n990 = Greater Or Equal?(x=w1680, y=w1676) -> (x >= y?=w1682:bool)
                    n991 = case shown="True" w1682 {
                      tunnel: w1677 -> [w1692 _]
                      tunnel: w1675 -> [w1691 _]
                      tunnel: w1674 -> [w1690 _]
                      tunnel: w1673 -> [w1689 _]
                      frame True {
                        n992 = stacked-sequence {
                          tunnel: w1692 -> [w1696 _]
                          tunnel: w1691 -> [w1694 w1700]
                          tunnel: w1690 -> [_ w1703]
                          tunnel: w1689 -> [w1693 _]
                          frame #0 {
                            n993 = Build Array(w1694) -> (w1697:string[])
                            n994 = Build Array(w1696) -> (w1695:dbl[])
                            n995 = TDMS Write(0:w1693, 5:"TEST PASS", 7:w1697, 9:w1695) -> (15:w1699:errorcluster)  [unwired: 2 in, 3 out]
                            n996 = local write "data file error"(w1699) -> ()
                          }
                          frame #1 {
                            n997 = Bundle(cluster=w1703, "STATUS"=w1700) -> (w1701:T4)  [unwired: 2 in]
                            n998 = local write "RESULT LAB05-1"(TRUE) -> ()
                            n999 = local write "DISP LAB05-1"(w1701) -> ()
                          }
                        }
                      }
                      frame False {
                      }
                    }
                  }
                }
              }
              frame #9 {
                # "LAB05-2"
                n1000 = Less?(x=w1704, y=2) -> (x < y?=w1707:bool)
                n1001 = local read "DISP LAB05-2"() -> (w1709:T4)
                n1002 = Unbundle(w1709) -> ("STATUS"=w1710:string)  [unwired: 2 out]
                n1003 = Equal?(x=w1710, y="RUN") -> (x = y?=w1706:bool)
                n1004 = And(x=w1706, y=w1707) -> (x .and. y?=w1705:bool)
                n1005 = case shown="True" w1705 {
                  tunnel: w1709 -> [_ w1713]
                  tunnel: w1704 -> [_ w1718]
                  frame False {
                  }
                  frame True {
                    n1006 = local read "SET LAB05-2"() -> (w1720:T5)
                    n1007 = local read "TDMS LAB05-2"() -> (w1712:refnum<k34>)
                    n1008 = Unbundle(w1713) -> ("CYCLE"=w1719:dbl)  [unwired: 2 out]
                    n1009 = Unbundle(w1720) -> ("CYCLES"=w1715:dbl, "T-RISE mins"=w1717:dbl)  [unwired: 3 out]
                    n1010 = case shown="\"T-RISE TEST\"" w1718 {
                      tunnel: w1717 -> [_ _ w1727]
                      tunnel: [w1722 w1724 w1727] -> w1716
                      tunnel: w1715 -> [w1722 w1724 _]
                      tunnel: ["CHART PASS" "CYCLE PASS" "T-RISE PASS"] -> w1714
                      frame "CHART TEST", Default {
                      }
                      frame "CYCLE TEST" {
                      }
                      frame "T-RISE TEST" {
                      }
                    }
                    n1011 = Greater Or Equal?(x=w1719, y=w1715) -> (x >= y?=w1721:bool)
                    n1012 = case shown="True" w1721 {
                      tunnel: w1716 -> [w1731 _]
                      tunnel: w1714 -> [w1730 _]
                      tunnel: w1713 -> [w1729 _]
                      tunnel: w1712 -> [w1728 _]
                      frame True {
                        n1013 = stacked-sequence {
                          tunnel: w1731 -> [w1735 _]
                          tunnel: w1730 -> [w1733 w1739]
                          tunnel: w1729 -> [_ w1742]
                          tunnel: w1728 -> [w1732 _]
                          frame #0 {
                            n1014 = Build Array(w1733) -> (w1736:string[])
                            n1015 = Build Array(w1735) -> (w1734:dbl[])
                            n1016 = TDMS Write(0:w1732, 5:"TEST PASS", 7:w1736, 9:w1734) -> (15:w1738:errorcluster)  [unwired: 2 in, 3 out]
                            n1017 = local write "data file error"(w1738) -> ()
                          }
                          frame #1 {
                            n1018 = Bundle(cluster=w1742, "STATUS"=w1739) -> (w1740:T4)  [unwired: 2 in]
                            n1019 = local write "RESULT LAB05-2"(TRUE) -> ()
                            n1020 = local write "DISP LAB05-2"(w1740) -> ()
                          }
                        }
                      }
                      frame False {
                      }
                    }
                  }
                }
              }
            }
          }
          frame #5 {
            # "check if test cycles reached for temperature rise test"
            n1021 = stacked-sequence {
              tunnel: w1772 -> [_ _ _ _ _ _ _ _ _ _]
              tunnel: w1771 -> [_ _ _ _ _ _ _ _ _ _]
              tunnel: w1770 -> [_ _ _ _ _ _ _ _ _ _]
              tunnel: w1769 -> [_ _ _ _ _ _ _ _ _ _]
              tunnel: w1768 -> [_ _ _ _ _ _ _ _ _ _]
              tunnel: w1767 -> [_ _ _ _ _ _ _ _ _ _]
              tunnel: w1766 -> [_ _ _ _ _ _ _ _ _ _]
              tunnel: w1765 -> [_ _ _ _ _ _ _ _ _ _]
              tunnel: w1764 -> [_ _ _ _ _ _ _ _ _ _]
              tunnel: w1763 -> [_ _ _ _ _ _ _ _ _ _]
              tunnel: w1762 -> [w1778 _ _ _ _ _ _ _ _ _]
              tunnel: w1752 -> [w1773 _ _ _ _ _ _ _ _ _]
              tunnel: w1761 -> [_ w1804 _ _ _ _ _ _ _ _]
              tunnel: w1760 -> [_ _ w1834 _ _ _ _ _ _ _]
              tunnel: w1759 -> [_ _ _ w1864 _ _ _ _ _ _]
              tunnel: w1758 -> [_ _ _ _ w1894 _ _ _ _ _]
              tunnel: w1757 -> [_ _ _ _ _ w1924 _ _ _ _]
              tunnel: w1756 -> [_ _ _ _ _ _ w1954 _ _ _]
              tunnel: w1755 -> [_ _ _ _ _ _ _ w1984 _ _]
              tunnel: w1754 -> [_ _ _ _ _ _ _ _ w2014 _]
              tunnel: w1753 -> [_ _ _ _ _ _ _ _ _ w2044]
              tunnel: w1751 -> [_ w1803 _ _ _ _ _ _ _ _]
              tunnel: w1750 -> [_ _ w1833 _ _ _ _ _ _ _]
              tunnel: w1749 -> [_ _ _ w1863 _ _ _ _ _ _]
              tunnel: w1748 -> [_ _ _ _ w1893 _ _ _ _ _]
              tunnel: w1747 -> [_ _ _ _ _ w1923 _ _ _ _]
              tunnel: w1746 -> [_ _ _ _ _ _ w1953 _ _ _]
              tunnel: w1745 -> [_ _ _ _ _ _ _ w1983 _ _]
              tunnel: w1744 -> [_ _ _ _ _ _ _ _ w2013 _]
              tunnel: w1743 -> [_ _ _ _ _ _ _ _ _ w2043]
              frame #0 {
                # "LAB01-1"
                n1022 = Equal?(x=w1778, y=2) -> (x = y?=w1776:bool)
                n1023 = local read "DISP LAB01-1"() -> (w1779:T4)
                n1024 = Unbundle(w1779) -> ("STATUS"=w1780:string)  [unwired: 2 out]
                n1025 = Equal?(x=w1780, y="RUN") -> (x = y?=w1775:bool)
                n1026 = And(x=w1775, y=w1776) -> (x .and. y?=w1774:bool)
                n1027 = case shown="True" w1774 {
                  tunnel: w1779 -> [_ w1783]
                  tunnel: w1773 -> [_ w1786]
                  frame False {
                  }
                  frame True {
                    n1028 = local read "SET LAB01-1"() -> (w1785:T5)
                    n1029 = local read "TDMS LAB01-1"() -> (w1782:refnum<k34>)
                    n1030 = Unbundle(w1783) -> ("CYCLE"=w1787:dbl)  [unwired: 2 out]
                    n1031 = Unbundle(w1785) -> ("T-RISE mins"=w1784:dbl)  [unwired: 4 out]
                    n1032 = Greater Or Equal?(x=w1787, y=w1786) -> (x >= y?=w1788:bool)
                    n1033 = case shown="True" w1788 {
                      tunnel: w1784 -> [w1791 _]
                      tunnel: w1783 -> [w1790 _]
                      tunnel: w1782 -> [w1789 _]
                      frame True {
                        n1034 = stacked-sequence {
                          tunnel: w1791 -> [w1794 _]
                          tunnel: w1790 -> [_ w1799]
                          tunnel: w1789 -> [w1792 _]
                          frame #0 {
                            n1035 = Build Array("T-RISE") -> (w1796:string[])
                            n1036 = Build Array(w1794) -> (w1795:dbl[])
                            n1037 = TDMS Write(0:w1792, 5:"TEST PASS", 7:w1796, 9:w1795) -> (15:w1798:errorcluster)  [unwired: 2 in, 3 out]
                            n1038 = local write "data file error"(w1798) -> ()
                          }
                          frame #1 {
                            n1039 = Bundle(cluster=w1799, "STATUS"="T-RISE PASS") -> (w1801:T4)  [unwired: 2 in]
                            n1040 = local write "RESULT LAB01-1"(TRUE) -> ()
                            n1041 = local write "DISP LAB01-1"(w1801) -> ()
                          }
                        }
                      }
                      frame False {
                      }
                    }
                  }
                }
              }
              frame #1 {
                # "LAB01-2"
                n1042 = Equal?(x=w1804, y=2) -> (x = y?=w1807:bool)
                n1043 = local read "DISP LAB01-2"() -> (w1809:T4)
                n1044 = Unbundle(w1809) -> ("STATUS"=w1810:string)  [unwired: 2 out]
                n1045 = Equal?(x=w1810, y="RUN") -> (x = y?=w1806:bool)
                n1046 = And(x=w1806, y=w1807) -> (x .and. y?=w1805:bool)
                n1047 = case shown="True" w1805 {
                  tunnel: w1809 -> [_ w1813]
                  tunnel: w1803 -> [_ w1816]
                  frame False {
                  }
                  frame True {
                    n1048 = local read "SET LAB01-2"() -> (w1815:T5)
                    n1049 = local read "TDMS LAB01-2"() -> (w1812:refnum<k34>)
                    n1050 = Unbundle(w1813) -> ("CYCLE"=w1817:dbl)  [unwired: 2 out]
                    n1051 = Unbundle(w1815) -> ("T-RISE mins"=w1814:dbl)  [unwired: 4 out]
                    n1052 = Greater Or Equal?(x=w1817, y=w1816) -> (x >= y?=w1818:bool)
                    n1053 = case shown="True" w1818 {
                      tunnel: w1814 -> [w1821 _]
                      tunnel: w1813 -> [w1820 _]
                      tunnel: w1812 -> [w1819 _]
                      frame True {
                        n1054 = stacked-sequence {
                          tunnel: w1821 -> [w1824 _]
                          tunnel: w1820 -> [_ w1829]
                          tunnel: w1819 -> [w1822 _]
                          frame #0 {
                            n1055 = Build Array("T-RISE") -> (w1826:string[])
                            n1056 = Build Array(w1824) -> (w1825:dbl[])
                            n1057 = TDMS Write(0:w1822, 5:"TEST PASS", 7:w1826, 9:w1825) -> (15:w1828:errorcluster)  [unwired: 2 in, 3 out]
                            n1058 = local write "data file error"(w1828) -> ()
                          }
                          frame #1 {
                            n1059 = Bundle(cluster=w1829, "STATUS"="T-RISE PASS") -> (w1831:T4)  [unwired: 2 in]
                            n1060 = local write "RESULT LAB01-2"(TRUE) -> ()
                            n1061 = local write "DISP LAB01-2"(w1831) -> ()
                          }
                        }
                      }
                      frame False {
                      }
                    }
                  }
                }
              }
              frame #2 {
                # "LAB02-1"
                n1062 = Equal?(x=w1834, y=2) -> (x = y?=w1837:bool)
                n1063 = local read "DISP LAB02-1"() -> (w1839:T4)
                n1064 = Unbundle(w1839) -> ("STATUS"=w1840:string)  [unwired: 2 out]
                n1065 = Equal?(x=w1840, y="RUN") -> (x = y?=w1836:bool)
                n1066 = And(x=w1836, y=w1837) -> (x .and. y?=w1835:bool)
                n1067 = case shown="True" w1835 {
                  tunnel: w1839 -> [_ w1843]
                  tunnel: w1833 -> [_ w1846]
                  frame False {
                  }
                  frame True {
                    n1068 = local read "SET LAB02-1"() -> (w1845:T5)
                    n1069 = local read "TDMS LAB02-1"() -> (w1842:refnum<k34>)
                    n1070 = Unbundle(w1843) -> ("CYCLE"=w1847:dbl)  [unwired: 2 out]
                    n1071 = Unbundle(w1845) -> ("T-RISE mins"=w1844:dbl)  [unwired: 4 out]
                    n1072 = Greater Or Equal?(x=w1847, y=w1846) -> (x >= y?=w1848:bool)
                    n1073 = case shown="True" w1848 {
                      tunnel: w1844 -> [w1851 _]
                      tunnel: w1843 -> [w1850 _]
                      tunnel: w1842 -> [w1849 _]
                      frame True {
                        n1074 = stacked-sequence {
                          tunnel: w1851 -> [w1854 _]
                          tunnel: w1850 -> [_ w1859]
                          tunnel: w1849 -> [w1852 _]
                          frame #0 {
                            n1075 = Build Array("T-RISE") -> (w1856:string[])
                            n1076 = Build Array(w1854) -> (w1855:dbl[])
                            n1077 = TDMS Write(0:w1852, 5:"TEST PASS", 7:w1856, 9:w1855) -> (15:w1858:errorcluster)  [unwired: 2 in, 3 out]
                            n1078 = local write "data file error"(w1858) -> ()
                          }
                          frame #1 {
                            n1079 = Bundle(cluster=w1859, "STATUS"="T-RISE PASS") -> (w1861:T4)  [unwired: 2 in]
                            n1080 = local write "RESULT LAB02-1"(TRUE) -> ()
                            n1081 = local write "DISP LAB02-1"(w1861) -> ()
                          }
                        }
                      }
                      frame False {
                      }
                    }
                  }
                }
              }
              frame #3 {
                # "LAB02-2"
                n1082 = Equal?(x=w1864, y=2) -> (x = y?=w1867:bool)
                n1083 = local read "DISP LAB02-2"() -> (w1869:T4)
                n1084 = Unbundle(w1869) -> ("STATUS"=w1870:string)  [unwired: 2 out]
                n1085 = Equal?(x=w1870, y="RUN") -> (x = y?=w1866:bool)
                n1086 = And(x=w1866, y=w1867) -> (x .and. y?=w1865:bool)
                n1087 = case shown="True" w1865 {
                  tunnel: w1869 -> [_ w1873]
                  tunnel: w1863 -> [_ w1876]
                  frame False {
                  }
                  frame True {
                    n1088 = local read "SET LAB02-2"() -> (w1875:T5)
                    n1089 = local read "TDMS LAB02-2"() -> (w1872:refnum<k34>)
                    n1090 = Unbundle(w1873) -> ("CYCLE"=w1877:dbl)  [unwired: 2 out]
                    n1091 = Unbundle(w1875) -> ("T-RISE mins"=w1874:dbl)  [unwired: 4 out]
                    n1092 = Greater Or Equal?(x=w1877, y=w1876) -> (x >= y?=w1878:bool)
                    n1093 = case shown="True" w1878 {
                      tunnel: w1874 -> [w1881 _]
                      tunnel: w1873 -> [w1880 _]
                      tunnel: w1872 -> [w1879 _]
                      frame True {
                        n1094 = stacked-sequence {
                          tunnel: w1881 -> [w1884 _]
                          tunnel: w1880 -> [_ w1889]
                          tunnel: w1879 -> [w1882 _]
                          frame #0 {
                            n1095 = Build Array("T-RISE") -> (w1886:string[])
                            n1096 = Build Array(w1884) -> (w1885:dbl[])
                            n1097 = TDMS Write(0:w1882, 5:"TEST PASS", 7:w1886, 9:w1885) -> (15:w1888:errorcluster)  [unwired: 2 in, 3 out]
                            n1098 = local write "data file error"(w1888) -> ()
                          }
                          frame #1 {
                            n1099 = Bundle(cluster=w1889, "STATUS"="T-RISE PASS") -> (w1891:T4)  [unwired: 2 in]
                            n1100 = local write "RESULT LAB02-2"(TRUE) -> ()
                            n1101 = local write "DISP LAB02-2"(w1891) -> ()
                          }
                        }
                      }
                      frame False {
                      }
                    }
                  }
                }
              }
              frame #4 {
                # "LAB03-1"
                n1102 = Equal?(x=w1894, y=2) -> (x = y?=w1897:bool)
                n1103 = local read "DISP LAB03-1"() -> (w1899:T4)
                n1104 = Unbundle(w1899) -> ("STATUS"=w1900:string)  [unwired: 2 out]
                n1105 = Equal?(x=w1900, y="RUN") -> (x = y?=w1896:bool)
                n1106 = And(x=w1896, y=w1897) -> (x .and. y?=w1895:bool)
                n1107 = case shown="True" w1895 {
                  tunnel: w1899 -> [_ w1903]
                  tunnel: w1893 -> [_ w1906]
                  frame False {
                  }
                  frame True {
                    n1108 = local read "SET LAB03-1"() -> (w1905:T5)
                    n1109 = local read "TDMS LAB03-1"() -> (w1902:refnum<k34>)
                    n1110 = Unbundle(w1903) -> ("CYCLE"=w1907:dbl)  [unwired: 2 out]
                    n1111 = Unbundle(w1905) -> ("T-RISE mins"=w1904:dbl)  [unwired: 4 out]
                    n1112 = Greater Or Equal?(x=w1907, y=w1906) -> (x >= y?=w1908:bool)
                    n1113 = case shown="True" w1908 {
                      tunnel: w1904 -> [w1911 _]
                      tunnel: w1903 -> [w1910 _]
                      tunnel: w1902 -> [w1909 _]
                      frame True {
                        n1114 = stacked-sequence {
                          tunnel: w1911 -> [w1914 _]
                          tunnel: w1910 -> [_ w1919]
                          tunnel: w1909 -> [w1912 _]
                          frame #0 {
                            n1115 = Build Array("T-RISE") -> (w1916:string[])
                            n1116 = Build Array(w1914) -> (w1915:dbl[])
                            n1117 = TDMS Write(0:w1912, 5:"TEST PASS", 7:w1916, 9:w1915) -> (15:w1918:errorcluster)  [unwired: 2 in, 3 out]
                            n1118 = local write "data file error"(w1918) -> ()
                          }
                          frame #1 {
                            n1119 = Bundle(cluster=w1919, "STATUS"="T-RISE PASS") -> (w1921:T4)  [unwired: 2 in]
                            n1120 = local write "RESULT LAB03-1"(TRUE) -> ()
                            n1121 = local write "DISP LAB03-1"(w1921) -> ()
                          }
                        }
                      }
                      frame False {
                      }
                    }
                  }
                }
              }
              frame #5 {
                # "LAB03-2"
                n1122 = Equal?(x=w1924, y=2) -> (x = y?=w1927:bool)
                n1123 = local read "DISP LAB03-2"() -> (w1929:T4)
                n1124 = Unbundle(w1929) -> ("STATUS"=w1930:string)  [unwired: 2 out]
                n1125 = Equal?(x=w1930, y="RUN") -> (x = y?=w1926:bool)
                n1126 = And(x=w1926, y=w1927) -> (x .and. y?=w1925:bool)
                n1127 = case shown="True" w1925 {
                  tunnel: w1929 -> [_ w1933]
                  tunnel: w1923 -> [_ w1936]
                  frame False {
                  }
                  frame True {
                    n1128 = local read "SET LAB03-2"() -> (w1935:T5)
                    n1129 = local read "TDMS LAB03-2"() -> (w1932:refnum<k34>)
                    n1130 = Unbundle(w1933) -> ("CYCLE"=w1937:dbl)  [unwired: 2 out]
                    n1131 = Unbundle(w1935) -> ("T-RISE mins"=w1934:dbl)  [unwired: 4 out]
                    n1132 = Greater Or Equal?(x=w1937, y=w1936) -> (x >= y?=w1938:bool)
                    n1133 = case shown="True" w1938 {
                      tunnel: w1934 -> [w1941 _]
                      tunnel: w1933 -> [w1940 _]
                      tunnel: w1932 -> [w1939 _]
                      frame True {
                        n1134 = stacked-sequence {
                          tunnel: w1941 -> [w1944 _]
                          tunnel: w1940 -> [_ w1949]
                          tunnel: w1939 -> [w1942 _]
                          frame #0 {
                            n1135 = Build Array("T-RISE") -> (w1946:string[])
                            n1136 = Build Array(w1944) -> (w1945:dbl[])
                            n1137 = TDMS Write(0:w1942, 5:"TEST PASS", 7:w1946, 9:w1945) -> (15:w1948:errorcluster)  [unwired: 2 in, 3 out]
                            n1138 = local write "data file error"(w1948) -> ()
                          }
                          frame #1 {
                            n1139 = Bundle(cluster=w1949, "STATUS"="T-RISE PASS") -> (w1951:T4)  [unwired: 2 in]
                            n1140 = local write "RESULT LAB03-2"(TRUE) -> ()
                            n1141 = local write "DISP LAB03-2"(w1951) -> ()
                          }
                        }
                      }
                      frame False {
                      }
                    }
                  }
                }
              }
              frame #6 {
                # "LAB04-1"
                n1142 = Equal?(x=w1954, y=2) -> (x = y?=w1957:bool)
                n1143 = local read "DISP LAB04-1"() -> (w1959:T4)
                n1144 = Unbundle(w1959) -> ("STATUS"=w1960:string)  [unwired: 2 out]
                n1145 = Equal?(x=w1960, y="RUN") -> (x = y?=w1956:bool)
                n1146 = And(x=w1956, y=w1957) -> (x .and. y?=w1955:bool)
                n1147 = case shown="True" w1955 {
                  tunnel: w1959 -> [_ w1963]
                  tunnel: w1953 -> [_ w1966]
                  frame False {
                  }
                  frame True {
                    n1148 = local read "SET LAB04-1"() -> (w1965:T5)
                    n1149 = local read "TDMS LAB04-1"() -> (w1962:refnum<k34>)
                    n1150 = Unbundle(w1963) -> ("CYCLE"=w1967:dbl)  [unwired: 2 out]
                    n1151 = Unbundle(w1965) -> ("T-RISE mins"=w1964:dbl)  [unwired: 4 out]
                    n1152 = Greater Or Equal?(x=w1967, y=w1966) -> (x >= y?=w1968:bool)
                    n1153 = case shown="True" w1968 {
                      tunnel: w1964 -> [w1971 _]
                      tunnel: w1963 -> [w1970 _]
                      tunnel: w1962 -> [w1969 _]
                      frame True {
                        n1154 = stacked-sequence {
                          tunnel: w1971 -> [w1974 _]
                          tunnel: w1970 -> [_ w1979]
                          tunnel: w1969 -> [w1972 _]
                          frame #0 {
                            n1155 = Build Array("T-RISE") -> (w1976:string[])
                            n1156 = Build Array(w1974) -> (w1975:dbl[])
                            n1157 = TDMS Write(0:w1972, 5:"TEST PASS", 7:w1976, 9:w1975) -> (15:w1978:errorcluster)  [unwired: 2 in, 3 out]
                            n1158 = local write "data file error"(w1978) -> ()
                          }
                          frame #1 {
                            n1159 = Bundle(cluster=w1979, "STATUS"="T-RISE PASS") -> (w1981:T4)  [unwired: 2 in]
                            n1160 = local write "RESULT LAB04-1"(TRUE) -> ()
                            n1161 = local write "DISP LAB04-1"(w1981) -> ()
                          }
                        }
                      }
                      frame False {
                      }
                    }
                  }
                }
              }
              frame #7 {
                # "LAB04-2"
                n1162 = Equal?(x=w1984, y=2) -> (x = y?=w1987:bool)
                n1163 = local read "DISP LAB04-2"() -> (w1989:T4)
                n1164 = Unbundle(w1989) -> ("STATUS"=w1990:string)  [unwired: 2 out]
                n1165 = Equal?(x=w1990, y="RUN") -> (x = y?=w1986:bool)
                n1166 = And(x=w1986, y=w1987) -> (x .and. y?=w1985:bool)
                n1167 = case shown="True" w1985 {
                  tunnel: w1989 -> [_ w1993]
                  tunnel: w1983 -> [_ w1996]
                  frame False {
                  }
                  frame True {
                    n1168 = local read "SET LAB04-2"() -> (w1995:T5)
                    n1169 = local read "TDMS LAB04-2"() -> (w1992:refnum<k34>)
                    n1170 = Unbundle(w1993) -> ("CYCLE"=w1997:dbl)  [unwired: 2 out]
                    n1171 = Unbundle(w1995) -> ("T-RISE mins"=w1994:dbl)  [unwired: 4 out]
                    n1172 = Greater Or Equal?(x=w1997, y=w1996) -> (x >= y?=w1998:bool)
                    n1173 = case shown="True" w1998 {
                      tunnel: w1994 -> [w2001 _]
                      tunnel: w1993 -> [w2000 _]
                      tunnel: w1992 -> [w1999 _]
                      frame True {
                        n1174 = stacked-sequence {
                          tunnel: w2001 -> [w2004 _]
                          tunnel: w2000 -> [_ w2009]
                          tunnel: w1999 -> [w2002 _]
                          frame #0 {
                            n1175 = Build Array("T-RISE") -> (w2006:string[])
                            n1176 = Build Array(w2004) -> (w2005:dbl[])
                            n1177 = TDMS Write(0:w2002, 5:"TEST PASS", 7:w2006, 9:w2005) -> (15:w2008:errorcluster)  [unwired: 2 in, 3 out]
                            n1178 = local write "data file error"(w2008) -> ()
                          }
                          frame #1 {
                            n1179 = Bundle(cluster=w2009, "STATUS"="T-RISE PASS") -> (w2011:T4)  [unwired: 2 in]
                            n1180 = local write "RESULT LAB04-2"(TRUE) -> ()
                            n1181 = local write "DISP LAB04-2"(w2011) -> ()
                          }
                        }
                      }
                      frame False {
                      }
                    }
                  }
                }
              }
              frame #8 {
                # "LAB05-1"
                n1182 = Equal?(x=w2014, y=2) -> (x = y?=w2017:bool)
                n1183 = local read "DISP LAB05-1"() -> (w2019:T4)
                n1184 = Unbundle(w2019) -> ("STATUS"=w2020:string)  [unwired: 2 out]
                n1185 = Equal?(x=w2020, y="RUN") -> (x = y?=w2016:bool)
                n1186 = And(x=w2016, y=w2017) -> (x .and. y?=w2015:bool)
                n1187 = case shown="True" w2015 {
                  tunnel: w2019 -> [_ w2023]
                  tunnel: w2013 -> [_ w2026]
                  frame False {
                  }
                  frame True {
                    n1188 = local read "SET LAB05-1"() -> (w2025:T5)
                    n1189 = local read "TDMS LAB05-1"() -> (w2022:refnum<k34>)
                    n1190 = Unbundle(w2023) -> ("CYCLE"=w2027:dbl)  [unwired: 2 out]
                    n1191 = Unbundle(w2025) -> ("T-RISE mins"=w2024:dbl)  [unwired: 4 out]
                    n1192 = Greater Or Equal?(x=w2027, y=w2026) -> (x >= y?=w2028:bool)
                    n1193 = case shown="True" w2028 {
                      tunnel: w2024 -> [w2031 _]
                      tunnel: w2023 -> [w2030 _]
                      tunnel: w2022 -> [w2029 _]
                      frame True {
                        n1194 = stacked-sequence {
                          tunnel: w2031 -> [w2034 _]
                          tunnel: w2030 -> [_ w2039]
                          tunnel: w2029 -> [w2032 _]
                          frame #0 {
                            n1195 = Build Array("T-RISE") -> (w2036:string[])
                            n1196 = Build Array(w2034) -> (w2035:dbl[])
                            n1197 = TDMS Write(0:w2032, 5:"TEST PASS", 7:w2036, 9:w2035) -> (15:w2038:errorcluster)  [unwired: 2 in, 3 out]
                            n1198 = local write "data file error"(w2038) -> ()
                          }
                          frame #1 {
                            n1199 = Bundle(cluster=w2039, "STATUS"="T-RISE PASS") -> (w2041:T4)  [unwired: 2 in]
                            n1200 = local write "RESULT LAB05-1"(TRUE) -> ()
                            n1201 = local write "DISP LAB05-1"(w2041) -> ()
                          }
                        }
                      }
                      frame False {
                      }
                    }
                  }
                }
              }
              frame #9 {
                # "LAB05-2"
                n1202 = Equal?(x=w2044, y=2) -> (x = y?=w2047:bool)
                n1203 = local read "DISP LAB05-2"() -> (w2049:T4)
                n1204 = Unbundle(w2049) -> ("STATUS"=w2050:string)  [unwired: 2 out]
                n1205 = Equal?(x=w2050, y="RUN") -> (x = y?=w2046:bool)
                n1206 = And(x=w2046, y=w2047) -> (x .and. y?=w2045:bool)
                n1207 = case shown="True" w2045 {
                  tunnel: w2049 -> [_ w2053]
                  tunnel: w2043 -> [_ w2056]
                  frame False {
                  }
                  frame True {
                    n1208 = local read "SET LAB05-2"() -> (w2055:T5)
                    n1209 = local read "TDMS LAB05-2"() -> (w2052:refnum<k34>)
                    n1210 = Unbundle(w2053) -> ("CYCLE"=w2057:dbl)  [unwired: 2 out]
                    n1211 = Unbundle(w2055) -> ("T-RISE mins"=w2054:dbl)  [unwired: 4 out]
                    n1212 = Greater Or Equal?(x=w2057, y=w2056) -> (x >= y?=w2058:bool)
                    n1213 = case shown="True" w2058 {
                      tunnel: w2054 -> [w2061 _]
                      tunnel: w2053 -> [w2060 _]
                      tunnel: w2052 -> [w2059 _]
                      frame True {
                        n1214 = stacked-sequence {
                          tunnel: w2061 -> [w2064 _]
                          tunnel: w2060 -> [_ w2069]
                          tunnel: w2059 -> [w2062 _]
                          frame #0 {
                            n1215 = Build Array("T-RISE") -> (w2066:string[])
                            n1216 = Build Array(w2064) -> (w2065:dbl[])
                            n1217 = TDMS Write(0:w2062, 5:"TEST PASS", 7:w2066, 9:w2065) -> (15:w2068:errorcluster)  [unwired: 2 in, 3 out]
                            n1218 = local write "data file error"(w2068) -> ()
                          }
                          frame #1 {
                            n1219 = Bundle(cluster=w2069, "STATUS"="T-RISE PASS") -> (w2071:T4)  [unwired: 2 in]
                            n1220 = local write "RESULT LAB05-2"(TRUE) -> ()
                            n1221 = local write "DISP LAB05-2"(w2071) -> ()
                          }
                        }
                      }
                      frame False {
                      }
                    }
                  }
                }
              }
            }
          }
          frame #6 {
            # "end test & close test files"
            n1222 = stacked-sequence {
              tunnel: w2082 -> [_ _ _ _ _ _ _ _ _ _]
              tunnel: w2083 -> [_ _ _ _ _ _ _ _ _ _]
              tunnel: w2081 -> [_ _ _ _ _ _ _ _ _ _]
              tunnel: w2080 -> [_ _ _ _ _ _ _ _ _ _]
              tunnel: w2079 -> [_ _ _ _ _ _ _ _ _ _]
              tunnel: w2078 -> [_ _ _ _ _ _ _ _ _ _]
              tunnel: w2077 -> [_ _ _ _ _ _ _ _ _ _]
              tunnel: w2076 -> [_ _ _ _ _ _ _ _ _ _]
              tunnel: w2075 -> [_ _ _ _ _ _ _ _ _ _]
              tunnel: w2074 -> [_ _ _ _ _ _ _ _ _ _]
              frame #0 {
                # "LAB01-1"
                n1223 = local read "DISP LAB01-1"() -> (w2087:T4)
                n1224 = local read "run lab01-1"() -> (w2084:bool)
                n1225 = local read "TDMS LAB01-1"() -> (w2085:refnum<k34>)
                n1226 = Unbundle(w2087) -> ("CYCLE"=w2088:dbl, "STATUS"=w2086:string)  [unwired: 1 out]
                n1227 = case shown="True" w2084 {
                  tunnel: w2088 -> [_ w2092]
                  tunnel: w2087 -> [_ w2091]
                  tunnel: w2086 -> [_ w2090]
                  tunnel: w2085 -> [_ w2089]
                  frame False {
                  }
                  frame True {
                    n1228 = Not Equal?(x=w2090, y="RUN") -> (x != y?=w2093:bool)
                    n1229 = Greater?(x=w2092, y=2.0) -> (0:w2095:bool)
                    n1230 = And(x=w2095, y=w2093) -> (x .and. y?=w2094:bool)
                    n1231 = case shown="True" w2094 {
                      tunnel: w2091 -> [_ w2099]
                      tunnel: w2089 -> [_ w2098]
                      frame False {
                      }
                      frame True {
                        n1232 = stacked-sequence {
                          tunnel: w2099 -> [w2102 _ _]
                          tunnel: w2098 -> [_ w2104 _]
                          frame #0 {
                            n1233 = local write "mail control"("END") -> ()
                            n1234 = Bundle(cluster=w2102) -> (w2101:T4)  [unwired: 3 in]
                            n1235 = local write "DISP LAB01-1"(w2101) -> ()
                          }
                          frame #1 {
                            n1236 = TDMS Close(11:w2104) -> (0:w2103:errorcluster)  [unwired: 1 in, 1 out]
                            n1237 = local write "data file error"(w2103) -> ()
                          }
                          frame #2 {
                            n1238 = stacked-sequence {
                              tunnel: "LAB01-1" -> [w2107 w2110]
                              frame #0 {
                                n1239 = call "sub vi - defrag tdms v1.vi"("panel id"=w2107) -> ("error out"=w2106:errorcluster)  [unwired: 10 in]
                                n1240 = local write "data file error"(w2106) -> ()
                              }
                              frame #1 {
                                w2108 = FALSE
                                n1241 = local write "O/I  LAB01-1"(w2108) -> ()
                                n1242 = local write "run lab01-1"(w2108) -> ()
                                n1243 = local write "RUN LAB01-1"(w2108) -> ()
                                n1244 = call "Save data file to network drive v1.vi"("panel id"=w2110) -> ("network file save error"=w2109:errorcluster)  [unwired: 9 in, 1 out]
                                n1245 = local write "data file error"(w2109) -> ()
                              }
                            }
                          }
                        }
                      }
                    }
                  }
                }
              }
              frame #1 {
                # "LAB01-2"
                n1246 = local read "run lab01-2"() -> (w2111:bool)
                n1247 = case shown="True" w2111 {
                  frame False {
                  }
                  frame True {
                    n1248 = local read "DISP LAB01-2"() -> (w2118:T4)
                    n1249 = local read "TDMS LAB01-2"() -> (w2117:refnum<k34>)
                    n1250 = Unbundle(w2118) -> ("CYCLE"=w2114:dbl, "STATUS"=w2119:string)  [unwired: 1 out]
                    n1251 = Not Equal?(x=w2119, y="RUN") -> (x != y?=w2113:bool)
                    n1252 = Greater?(x=w2114, y=2.0) -> (0:w2115:bool)
                    n1253 = And(x=w2115, y=w2113) -> (x .and. y?=w2112:bool)
                    n1254 = case shown="True" w2112 {
                      tunnel: w2118 -> [_ w2122]
                      tunnel: w2117 -> [_ w2121]
                      frame False {
                      }
                      frame True {
                        n1255 = stacked-sequence {
                          tunnel: w2122 -> [w2125 _ _]
                          tunnel: w2121 -> [_ w2127 _]
                          frame #0 {
                            w2123 = FALSE
                            n1256 = local write "mail control"("END") -> ()
                            n1257 = Bundle(cluster=w2125) -> (w2126:T4)  [unwired: 3 in]
                            n1258 = local write "RUN LAB01-2"(w2123) -> ()
                            n1259 = local write "run lab01-2"(w2123) -> ()
                            n1260 = local write "O/I  LAB01-2"(w2123) -> ()
                            n1261 = local write "DISP LAB01-2"(w2126) -> ()
                          }
                          frame #1 {
                            n1262 = TDMS Close(11:w2127) -> (0:w2128:errorcluster)  [unwired: 1 in, 1 out]
                            n1263 = local write "data file error"(w2128) -> ()
                          }
                          frame #2 {
                            n1264 = stacked-sequence {
                              tunnel: "LAB01-2" -> [w2131 w2133]
                              frame #0 {
                                n1265 = call "sub vi - defrag tdms v1.vi"("panel id"=w2131) -> ("error out"=w2130:errorcluster)  [unwired: 10 in]
                                n1266 = local write "data file error"(w2130) -> ()
                              }
                              frame #1 {
                                n1267 = call "Save data file to network drive v1.vi"("panel id"=w2133) -> ("network file save error"=w2132:errorcluster)  [unwired: 9 in, 1 out]
                                n1268 = local write "data file error"(w2132) -> ()
                              }
                            }
                          }
                        }
                      }
                    }
                  }
                }
              }
              frame #2 {
                # "LAB02-1"
                n1269 = local read "run lab02-1"() -> (w2134:bool)
                n1270 = case shown="True" w2134 {
                  frame False {
                  }
                  frame True {
                    n1271 = local read "DISP LAB02-1"() -> (w2141:T4)
                    n1272 = Unbundle(w2141) -> ("CYCLE"=w2137:dbl, "STATUS"=w2142:string)  [unwired: 1 out]
                    n1273 = local read "TDMS LAB02-1"() -> (w2140:refnum<k34>)
                    n1274 = Not Equal?(x=w2142, y="RUN") -> (x != y?=w2136:bool)
                    n1275 = Greater?(x=w2137, y=2.0) -> (0:w2138:bool)
                    n1276 = And(x=w2138, y=w2136) -> (x .and. y?=w2135:bool)
                    n1277 = case shown="True" w2135 {
                      tunnel: w2141 -> [_ w2145]
                      tunnel: w2140 -> [_ w2144]
                      frame False {
                      }
                      frame True {
                        n1278 = stacked-sequence {
                          tunnel: w2145 -> [w2148 _ _]
                          tunnel: w2144 -> [_ w2150 _]
                          frame #0 {
                            w2146 = FALSE
                            n1279 = local write "mail control"("END") -> ()
                            n1280 = Bundle(cluster=w2148) -> (w2149:T4)  [unwired: 3 in]
                            n1281 = local write "O/I  LAB02-1"(w2146) -> ()
                            n1282 = local write "RUN LAB02-1"(w2146) -> ()
                            n1283 = local write "run lab02-1"(w2146) -> ()
                            n1284 = local write "DISP LAB02-1"(w2149) -> ()
                          }
                          frame #1 {
                            n1285 = TDMS Close(11:w2150) -> (0:w2151:errorcluster)  [unwired: 1 in, 1 out]
                            n1286 = local write "data file error"(w2151) -> ()
                          }
                          frame #2 {
                            n1287 = stacked-sequence {
                              tunnel: "LAB02-1" -> [w2154 w2156]
                              frame #0 {
                                n1288 = call "sub vi - defrag tdms v1.vi"("panel id"=w2154) -> ("error out"=w2153:errorcluster)  [unwired: 10 in]
                                n1289 = local write "data file error"(w2153) -> ()
                              }
                              frame #1 {
                                n1290 = call "Save data file to network drive v1.vi"("panel id"=w2156) -> ("network file save error"=w2155:errorcluster)  [unwired: 9 in, 1 out]
                                n1291 = local write "data file error"(w2155) -> ()
                              }
                            }
                          }
                        }
                      }
                    }
                  }
                }
              }
              frame #3 {
                # "LAB02-2"
                n1292 = local read "run lab02-2"() -> (w2157:bool)
                n1293 = case shown="True" w2157 {
                  frame False {
                  }
                  frame True {
                    n1294 = local read "DISP LAB02-2"() -> (w2164:T4)
                    n1295 = local read "TDMS LAB02-2"() -> (w2163:refnum<k34>)
                    n1296 = Unbundle(w2164) -> ("CYCLE"=w2160:dbl, "STATUS"=w2165:string)  [unwired: 1 out]
                    n1297 = Not Equal?(x=w2165, y="RUN") -> (x != y?=w2159:bool)
                    n1298 = Greater?(x=w2160, y=2.0) -> (0:w2161:bool)
                    n1299 = And(x=w2161, y=w2159) -> (x .and. y?=w2158:bool)
                    n1300 = case shown="True" w2158 {
                      tunnel: w2164 -> [_ w2168]
                      tunnel: w2163 -> [_ w2167]
                      frame False {
                      }
                      frame True {
                        n1301 = stacked-sequence {
                          tunnel: w2168 -> [w2171 _ _]
                          tunnel: w2167 -> [_ w2173 _]
                          frame #0 {
                            w2169 = FALSE
                            n1302 = local write "mail control"("END") -> ()
                            n1303 = Bundle(cluster=w2171) -> (w2172:T4)  [unwired: 3 in]
                            n1304 = local write "run lab02-2"(w2169) -> ()
                            n1305 = local write "RUN LAB02-2"(w2169) -> ()
                            n1306 = local write "DISP LAB02-2"(w2172) -> ()
                          }
                          frame #1 {
                            n1307 = TDMS Close(11:w2173) -> (0:w2174:errorcluster)  [unwired: 1 in, 1 out]
                            n1308 = local write "data file error"(w2174) -> ()
                          }
                          frame #2 {
                            n1309 = stacked-sequence {
                              tunnel: "LAB02-2" -> [w2177 w2179]
                              frame #0 {
                                n1310 = call "sub vi - defrag tdms v1.vi"("panel id"=w2177) -> ("error out"=w2176:errorcluster)  [unwired: 10 in]
                                n1311 = local write "data file error"(w2176) -> ()
                              }
                              frame #1 {
                                n1312 = call "Save data file to network drive v1.vi"("panel id"=w2179) -> ("network file save error"=w2178:errorcluster)  [unwired: 9 in, 1 out]
                                n1313 = local write "data file error"(w2178) -> ()
                              }
                            }
                          }
                        }
                      }
                    }
                  }
                }
              }
              frame #4 {
                # "LAB03-1"
                n1314 = local read "run lab03-1"() -> (w2180:bool)
                n1315 = case shown="True" w2180 {
                  frame False {
                  }
                  frame True {
                    n1316 = local read "DISP LAB03-1"() -> (w2187:T4)
                    n1317 = local read "TDMS LAB03-1"() -> (w2186:refnum<k34>)
                    n1318 = Unbundle(w2187) -> ("CYCLE"=w2183:dbl, "STATUS"=w2188:string)  [unwired: 1 out]
                    n1319 = Not Equal?(x=w2188, y="RUN") -> (x != y?=w2182:bool)
                    n1320 = Greater?(x=w2183, y=2.0) -> (0:w2184:bool)
                    n1321 = And(x=w2184, y=w2182) -> (x .and. y?=w2181:bool)
                    n1322 = case shown="True" w2181 {
                      tunnel: w2187 -> [_ w2191]
                      tunnel: w2186 -> [_ w2190]
                      frame False {
                      }
                      frame True {
                        n1323 = stacked-sequence {
                          tunnel: w2191 -> [w2194 _ _]
                          tunnel: w2190 -> [_ w2196 _]
                          frame #0 {
                            w2192 = FALSE
                            n1324 = local write "mail control"("END") -> ()
                            n1325 = Bundle(cluster=w2194) -> (w2195:T4)  [unwired: 3 in]
                            n1326 = local write "O/I  LAB03-1"(w2192) -> ()
                            n1327 = local write "run lab03-1"(w2192) -> ()
                            n1328 = local write "RUN LAB03-1"(w2192) -> ()
                            n1329 = local write "DISP LAB03-1"(w2195) -> ()
                          }
                          frame #1 {
                            n1330 = TDMS Close(11:w2196) -> (0:w2197:errorcluster)  [unwired: 1 in, 1 out]
                            n1331 = local write "data file error"(w2197) -> ()
                          }
                          frame #2 {
                            n1332 = stacked-sequence {
                              tunnel: "LAB03-1" -> [w2200 w2202]
                              frame #0 {
                                n1333 = call "sub vi - defrag tdms v1.vi"("panel id"=w2200) -> ("error out"=w2199:errorcluster)  [unwired: 10 in]
                                n1334 = local write "data file error"(w2199) -> ()
                              }
                              frame #1 {
                                n1335 = call "Save data file to network drive v1.vi"("panel id"=w2202) -> ("network file save error"=w2201:errorcluster)  [unwired: 9 in, 1 out]
                                n1336 = local write "data file error"(w2201) -> ()
                              }
                            }
                          }
                        }
                      }
                    }
                  }
                }
              }
              frame #5 {
                # "LAB03-2"
                n1337 = local read "run lab03-2"() -> (w2203:bool)
                n1338 = case shown="True" w2203 {
                  frame False {
                  }
                  frame True {
                    n1339 = local read "DISP LAB03-2"() -> (w2210:T4)
                    n1340 = Unbundle(w2210) -> ("CYCLE"=w2206:dbl, "STATUS"=w2211:string)  [unwired: 1 out]
                    n1341 = local read "TDMS LAB03-2"() -> (w2209:refnum<k34>)
                    n1342 = Not Equal?(x=w2211, y="RUN") -> (x != y?=w2205:bool)
                    n1343 = Greater?(x=w2206, y=2.0) -> (0:w2207:bool)
                    n1344 = And(x=w2207, y=w2205) -> (x .and. y?=w2204:bool)
                    n1345 = case shown="True" w2204 {
                      tunnel: w2210 -> [_ w2214]
                      tunnel: w2209 -> [_ w2213]
                      frame False {
                      }
                      frame True {
                        n1346 = stacked-sequence {
                          tunnel: w2214 -> [w2217 _ _]
                          tunnel: w2213 -> [_ w2219 _]
                          frame #0 {
                            w2215 = FALSE
                            n1347 = local write "mail control"("END") -> ()
                            n1348 = Bundle(cluster=w2217) -> (w2218:T4)  [unwired: 3 in]
                            n1349 = local write "RUN LAB03-2"(w2215) -> ()
                            n1350 = local write "O/I  LAB03-2"(w2215) -> ()
                            n1351 = local write "DISP LAB03-2"(w2218) -> ()
                            n1352 = local write "run lab03-2"(w2215) -> ()
                          }
                          frame #1 {
                            n1353 = TDMS Close(11:w2219) -> (0:w2220:errorcluster)  [unwired: 1 in, 1 out]
                            n1354 = local write "data file error"(w2220) -> ()
                          }
                          frame #2 {
                            n1355 = stacked-sequence {
                              tunnel: "LAB03-2" -> [w2223 w2225]
                              frame #0 {
                                n1356 = call "sub vi - defrag tdms v1.vi"("panel id"=w2223) -> ("error out"=w2222:errorcluster)  [unwired: 10 in]
                                n1357 = local write "data file error"(w2222) -> ()
                              }
                              frame #1 {
                                n1358 = call "Save data file to network drive v1.vi"("panel id"=w2225) -> ("network file save error"=w2224:errorcluster)  [unwired: 9 in, 1 out]
                                n1359 = local write "data file error"(w2224) -> ()
                              }
                            }
                          }
                        }
                      }
                    }
                  }
                }
              }
              frame #6 {
                # "LAB04-1"
                n1360 = local read "run lab04-1"() -> (w2226:bool)
                n1361 = case shown="True" w2226 {
                  frame False {
                  }
                  frame True {
                    n1362 = local read "DISP LAB04-1"() -> (w2233:T4)
                    n1363 = Unbundle(w2233) -> ("CYCLE"=w2229:dbl, "STATUS"=w2234:string)  [unwired: 1 out]
                    n1364 = local read "TDMS LAB04-1"() -> (w2232:refnum<k34>)
                    n1365 = Not Equal?(x=w2234, y="RUN") -> (x != y?=w2228:bool)
                    n1366 = Greater?(x=w2229, y=2.0) -> (0:w2230:bool)
                    n1367 = And(x=w2230, y=w2228) -> (x .and. y?=w2227:bool)
                    n1368 = case shown="True" w2227 {
                      tunnel: w2233 -> [_ w2237]
                      tunnel: w2232 -> [_ w2236]
                      frame False {
                      }
                      frame True {
                        n1369 = stacked-sequence {
                          tunnel: w2237 -> [w2240 _ _]
                          tunnel: w2236 -> [_ w2242 _]
                          frame #0 {
                            w2238 = FALSE
                            n1370 = local write "mail control"("END") -> ()
                            n1371 = Bundle(cluster=w2240) -> (w2241:T4)  [unwired: 3 in]
                            n1372 = local write "RUN LAB04-1"(w2238) -> ()
                            n1373 = local write "O/I  LAB04-1"(w2238) -> ()
                            n1374 = local write "run lab04-1"(w2238) -> ()
                            n1375 = local write "DISP LAB04-1"(w2241) -> ()
                          }
                          frame #1 {
                            n1376 = TDMS Close(11:w2242) -> (0:w2243:errorcluster)  [unwired: 1 in, 1 out]
                            n1377 = local write "data file error"(w2243) -> ()
                          }
                          frame #2 {
                            n1378 = stacked-sequence {
                              tunnel: "LAB04-1" -> [w2246 w2248]
                              frame #0 {
                                n1379 = call "sub vi - defrag tdms v1.vi"("panel id"=w2246) -> ("error out"=w2245:errorcluster)  [unwired: 10 in]
                                n1380 = local write "data file error"(w2245) -> ()
                              }
                              frame #1 {
                                n1381 = call "Save data file to network drive v1.vi"("panel id"=w2248) -> ("network file save error"=w2247:errorcluster)  [unwired: 9 in, 1 out]
                                n1382 = local write "data file error"(w2247) -> ()
                              }
                            }
                          }
                        }
                      }
                    }
                  }
                }
              }
              frame #7 {
                # "LAB04-2"
                n1383 = local read "run lab04-2"() -> (w2249:bool)
                n1384 = case shown="True" w2249 {
                  frame False {
                  }
                  frame True {
                    n1385 = local read "DISP LAB04-2"() -> (w2256:T4)
                    n1386 = Unbundle(w2256) -> ("CYCLE"=w2252:dbl, "STATUS"=w2257:string)  [unwired: 1 out]
                    n1387 = Not Equal?(x=w2257, y="RUN") -> (x != y?=w2251:bool)
                    n1388 = local read "TDMS LAB04-2"() -> (w2255:refnum<k34>)
                    n1389 = Greater?(x=w2252, y=2.0) -> (0:w2253:bool)
                    n1390 = And(x=w2253, y=w2251) -> (x .and. y?=w2250:bool)
                    n1391 = case shown="True" w2250 {
                      tunnel: w2256 -> [_ w2260]
                      tunnel: w2255 -> [_ w2259]
                      frame False {
                      }
                      frame True {
                        n1392 = stacked-sequence {
                          tunnel: w2260 -> [w2263 _ _]
                          tunnel: w2259 -> [_ w2265 _]
                          frame #0 {
                            w2261 = FALSE
                            n1393 = local write "mail control"("END") -> ()
                            n1394 = Bundle(cluster=w2263) -> (w2264:T4)  [unwired: 3 in]
                            n1395 = local write "O/I  LAB04-2"(w2261) -> ()
                            n1396 = local write "RUN LAB04-2"(w2261) -> ()
                            n1397 = local write "run lab04-2"(w2261) -> ()
                            n1398 = local write "DISP LAB04-2"(w2264) -> ()
                          }
                          frame #1 {
                            n1399 = TDMS Close(11:w2265) -> (0:w2266:errorcluster)  [unwired: 1 in, 1 out]
                            n1400 = local write "data file error"(w2266) -> ()
                          }
                          frame #2 {
                            n1401 = stacked-sequence {
                              tunnel: "LAB04-2" -> [w2269 w2271]
                              frame #0 {
                                n1402 = call "sub vi - defrag tdms v1.vi"("panel id"=w2269) -> ("error out"=w2268:errorcluster)  [unwired: 10 in]
                                n1403 = local write "data file error"(w2268) -> ()
                              }
                              frame #1 {
                                n1404 = call "Save data file to network drive v1.vi"("panel id"=w2271) -> ("network file save error"=w2270:errorcluster)  [unwired: 9 in, 1 out]
                                n1405 = local write "data file error"(w2270) -> ()
                              }
                            }
                          }
                        }
                      }
                    }
                  }
                }
              }
              frame #8 {
                # "LAB05-1"
                n1406 = local read "run lab05-1"() -> (w2272:bool)
                n1407 = case shown="True" w2272 {
                  frame False {
                  }
                  frame True {
                    n1408 = local read "DISP LAB05-1"() -> (w2279:T4)
                    n1409 = Unbundle(w2279) -> ("CYCLE"=w2275:dbl, "STATUS"=w2280:string)  [unwired: 1 out]
                    n1410 = Not Equal?(x=w2280, y="RUN") -> (x != y?=w2274:bool)
                    n1411 = local read "TDMS LAB05-1"() -> (w2278:refnum<k34>)
                    n1412 = Greater?(x=w2275, y=2.0) -> (0:w2276:bool)
                    n1413 = And(x=w2276, y=w2274) -> (x .and. y?=w2273:bool)
                    n1414 = case shown="True" w2273 {
                      tunnel: w2279 -> [_ w2283]
                      tunnel: w2278 -> [_ w2282]
                      frame False {
                      }
                      frame True {
                        n1415 = stacked-sequence {
                          tunnel: w2283 -> [w2286 _ _]
                          tunnel: w2282 -> [_ w2288 _]
                          frame #0 {
                            w2284 = FALSE
                            n1416 = local write "mail control"("END") -> ()
                            n1417 = Bundle(cluster=w2286) -> (w2287:T4)  [unwired: 3 in]
                            n1418 = local write "O/I  LAB05-1"(w2284) -> ()
                            n1419 = local write "RUN LAB05-1"(w2284) -> ()
                            n1420 = local write "run lab05-1"(w2284) -> ()
                            n1421 = local write "DISP LAB05-1"(w2287) -> ()
                          }
                          frame #1 {
                            n1422 = TDMS Close(11:w2288) -> (0:w2289:errorcluster)  [unwired: 1 in, 1 out]
                            n1423 = local write "data file error"(w2289) -> ()
                          }
                          frame #2 {
                            n1424 = stacked-sequence {
                              tunnel: "LAB05-1" -> [w2292 w2294]
                              frame #0 {
                                n1425 = call "sub vi - defrag tdms v1.vi"("panel id"=w2292) -> ("error out"=w2291:errorcluster)  [unwired: 10 in]
                                n1426 = local write "data file error"(w2291) -> ()
                              }
                              frame #1 {
                                n1427 = call "Save data file to network drive v1.vi"("panel id"=w2294) -> ("network file save error"=w2293:errorcluster)  [unwired: 9 in, 1 out]
                                n1428 = local write "data file error"(w2293) -> ()
                              }
                            }
                          }
                        }
                      }
                    }
                  }
                }
              }
              frame #9 {
                # "LAB05-2"
                n1429 = local read "run lab05-2"() -> (w2295:bool)
                n1430 = case shown="True" w2295 {
                  frame False {
                  }
                  frame True {
                    n1431 = local read "DISP LAB05-2"() -> (w2302:T4)
                    n1432 = Unbundle(w2302) -> ("CYCLE"=w2298:dbl, "STATUS"=w2303:string)  [unwired: 1 out]
                    n1433 = Not Equal?(x=w2303, y="RUN") -> (x != y?=w2297:bool)
                    n1434 = local read "TDMS LAB05-2"() -> (w2301:refnum<k34>)
                    n1435 = Greater?(x=w2298, y=2.0) -> (0:w2299:bool)
                    n1436 = And(x=w2299, y=w2297) -> (x .and. y?=w2296:bool)
                    n1437 = case shown="True" w2296 {
                      tunnel: w2302 -> [_ w2306]
                      tunnel: w2301 -> [_ w2305]
                      frame False {
                      }
                      frame True {
                        n1438 = stacked-sequence {
                          tunnel: w2306 -> [w2309 _ _]
                          tunnel: w2305 -> [_ w2311 _]
                          frame #0 {
                            w2307 = FALSE
                            n1439 = local write "mail control"("END") -> ()
                            n1440 = Bundle(cluster=w2309) -> (w2310:T4)  [unwired: 3 in]
                            n1441 = local write "RUN LAB05-2"(w2307) -> ()
                            n1442 = local write "O/I  LAB05-2"(w2307) -> ()
                            n1443 = local write "run lab05-2"(w2307) -> ()
                            n1444 = local write "DISP LAB05-2"(w2310) -> ()
                          }
                          frame #1 {
                            n1445 = TDMS Close(11:w2311) -> (0:w2312:errorcluster)  [unwired: 1 in, 1 out]
                            n1446 = local write "data file error"(w2312) -> ()
                          }
                          frame #2 {
                            n1447 = stacked-sequence {
                              tunnel: "LAB05-2" -> [w2315 w2317]
                              frame #0 {
                                n1448 = call "sub vi - defrag tdms v1.vi"("panel id"=w2315) -> ("error out"=w2314:errorcluster)  [unwired: 10 in]
                                n1449 = local write "data file error"(w2314) -> ()
                              }
                              frame #1 {
                                n1450 = call "Save data file to network drive v1.vi"("panel id"=w2317) -> ("network file save error"=w2316:errorcluster)  [unwired: 9 in, 1 out]
                                n1451 = local write "data file error"(w2316) -> ()
                              }
                            }
                          }
                        }
                      }
                    }
                  }
                }
              }
            }
            n1452 = local read "Network Directory"() -> (w2073:path)
            n1453 = global write "Global 1.vi" "Network Drive"(w2073) -> ()
          }
          frame #7 {
            # "disable functions"
            n1454 = stacked-sequence {
              tunnel: w2327 -> [w2341 _ w2397]
              tunnel: w2326 -> [w2336 _ w2396]
              tunnel: w2325 -> [w2335 _ w2395]
              tunnel: w2324 -> [w2333 _ w2394]
              tunnel: w2323 -> [w2334 _ w2393]
              tunnel: w2322 -> [_ w2358 w2392]
              tunnel: w2321 -> [_ w2359 w2391]
              tunnel: w2320 -> [_ w2360 w2390]
              tunnel: w2319 -> [_ w2361 w2389]
              tunnel: w2318 -> [_ w2362 w2388]
              frame #0 {
                n1455 = Select(t=2, s=w2333, f=0) -> (s? t:f=w2329:i32)
                n1456 = Select(t=2, s=w2335, f=0) -> (s? t:f=w2330:i32)
                n1457 = Select(t=2, s=w2334, f=0) -> (s? t:f=w2328:i32)
                n1458 = Select(t=2, s=w2341, f=0) -> (s? t:f=w2332:i32)
                n1459 = Select(t=2, s=w2336, f=0) -> (s? t:f=w2331:i32)
                n1460 = property on="SELECT LAB02-2" class="RadioBtnsControl (strict)"("DisabledEnum"=w2329) -> ()  [unwired: 2 in, 2 out]
                n1461 = property on="SELECT LAB02-1" class="RadioBtnsControl (strict)"("DisabledEnum"=w2330) -> ()  [unwired: 2 in, 2 out]
                n1462 = property on="SELECT LAB03-1" class="RadioBtnsControl (strict)"("DisabledEnum"=w2328) -> ()  [unwired: 2 in, 2 out]
                n1463 = property on="SELECT LAB01-1" class="RadioBtnsControl (strict)"("DisabledEnum"=w2332) -> ()  [unwired: 2 in, 2 out]
                n1464 = property on="SELECT LAB01-2" class="RadioBtnsControl (strict)"("DisabledEnum"=w2331) -> ()  [unwired: 2 in, 2 out]
                n1465 = Not(x=w2341) -> (.not. x?=w2342:bool)
                n1466 = property on="RESULT LAB01-1" class="Bool (strict)"("Visible"=w2342) -> ()  [unwired: 2 in, 2 out]
                n1467 = Not(x=w2336) -> (.not. x?=w2340:bool)
                n1468 = Not(x=w2335) -> (.not. x?=w2339:bool)
                n1469 = Not(x=w2333) -> (.not. x?=w2338:bool)
                n1470 = property on="RESULT LAB01-2" class="Bool (strict)"("Visible"=w2340) -> ()  [unwired: 2 in, 2 out]
                n1471 = Not(x=w2334) -> (.not. x?=w2337:bool)
                n1472 = property on="RESULT LAB02-1" class="Bool (strict)"("Visible"=w2339) -> ()  [unwired: 2 in, 2 out]
                n1473 = property on="RESULT LAB02-2" class="Bool (strict)"("Visible"=w2338) -> ()  [unwired: 2 in, 2 out]
                n1474 = property on="RESULT LAB03-1" class="Bool (strict)"("Visible"=w2337) -> ()  [unwired: 2 in, 2 out]
                n1475 = property on="SET LAB01-1" class="Clust (strict)"("DisabledEnum"=w2332) -> ()  [unwired: 2 in, 2 out]
                n1476 = property on="SET LAB01-2" class="Clust (strict)"("DisabledEnum"=w2331) -> ()  [unwired: 2 in, 2 out]
                n1477 = property on="SET LAB02-1" class="Clust (strict)"("DisabledEnum"=w2330) -> ()  [unwired: 2 in, 2 out]
                n1478 = property on="SET LAB02-2" class="Clust (strict)"("DisabledEnum"=w2329) -> ()  [unwired: 2 in, 2 out]
                n1479 = property on="SET LAB03-1" class="Clust (strict)"("DisabledEnum"=w2328) -> ()  [unwired: 2 in, 2 out]
                n1480 = property on="O/I  LAB01-1" class="Bool (strict)"("DisabledEnum"=w2332) -> ()  [unwired: 2 in, 2 out]
                n1481 = property on="O/I  LAB01-2" class="Bool (strict)"("DisabledEnum"=w2331) -> ()  [unwired: 2 in, 2 out]
                n1482 = property on="O/I  LAB02-1" class="Bool (strict)"("DisabledEnum"=w2330) -> ()  [unwired: 2 in, 2 out]
                n1483 = property on="O/I  LAB02-2" class="Bool (strict)"("DisabledEnum"=w2329) -> ()  [unwired: 2 in, 2 out]
                n1484 = property on="O/I  LAB03-1" class="Bool (strict)"("DisabledEnum"=w2328) -> ()  [unwired: 2 in, 2 out]
              }
              frame #1 {
                n1485 = Select(t=2, s=w2362, f=0) -> (s? t:f=w2353:i32)
                n1486 = Select(t=2, s=w2361, f=0) -> (s? t:f=w2354:i32)
                n1487 = Select(t=2, s=w2358, f=0) -> (s? t:f=w2357:i32)
                n1488 = Select(t=2, s=w2359, f=0) -> (s? t:f=w2356:i32)
                n1489 = Select(t=2, s=w2360, f=0) -> (s? t:f=w2355:i32)
                n1490 = property on="SELECT LAB05-2" class="RadioBtnsControl (strict)"("DisabledEnum"=w2353) -> ()  [unwired: 2 in, 2 out]
                n1491 = property on="SELECT LAB05-1" class="RadioBtnsControl (strict)"("DisabledEnum"=w2354) -> ()  [unwired: 2 in, 2 out]
                n1492 = property on="SELECT LAB03-2" class="RadioBtnsControl (strict)"("DisabledEnum"=w2357) -> ()  [unwired: 2 in, 2 out]
                n1493 = property on="SELECT LAB04-1" class="RadioBtnsControl (strict)"("DisabledEnum"=w2356) -> ()  [unwired: 2 in, 2 out]
                n1494 = property on="SELECT LAB04-2" class="RadioBtnsControl (strict)"("DisabledEnum"=w2355) -> ()  [unwired: 2 in, 2 out]
                n1495 = property on="SET LAB05-2" class="Clust (strict)"("DisabledEnum"=w2353) -> ()  [unwired: 2 in, 2 out]
                n1496 = property on="SET LAB05-1" class="Clust (strict)"("DisabledEnum"=w2354) -> ()  [unwired: 2 in, 2 out]
                n1497 = property on="SET LAB03-2" class="Clust (strict)"("DisabledEnum"=w2357) -> ()  [unwired: 2 in, 2 out]
                n1498 = property on="SET LAB04-1" class="Clust (strict)"("DisabledEnum"=w2356) -> ()  [unwired: 2 in, 2 out]
                n1499 = property on="SET LAB04-2" class="Clust (strict)"("DisabledEnum"=w2355) -> ()  [unwired: 2 in, 2 out]
                n1500 = property on="O/I  LAB05-2" class="Bool (strict)"("DisabledEnum"=w2353) -> ()  [unwired: 2 in, 2 out]
                n1501 = property on="O/I  LAB05-1" class="Bool (strict)"("DisabledEnum"=w2354) -> ()  [unwired: 2 in, 2 out]
                n1502 = property on="O/I  LAB04-1" class="Bool (strict)"("DisabledEnum"=w2356) -> ()  [unwired: 2 in, 2 out]
                n1503 = property on="O/I  LAB04-2" class="Bool (strict)"("DisabledEnum"=w2355) -> ()  [unwired: 2 in, 2 out]
                n1504 = property on="O/I  LAB03-2" class="Bool (strict)"("DisabledEnum"=w2357) -> ()  [unwired: 2 in, 2 out]
                n1505 = Not(x=w2362) -> (.not. x?=w2363:bool)
                n1506 = Not(x=w2361) -> (.not. x?=w2364:bool)
                n1507 = Not(x=w2360) -> (.not. x?=w2365:bool)
                n1508 = property on="RESULT LAB05-2" class="Bool (strict)"("Visible"=w2363) -> ()  [unwired: 2 in, 2 out]
                n1509 = property on="RESULT LAB05-1" class="Bool (strict)"("Visible"=w2364) -> ()  [unwired: 2 in, 2 out]
                n1510 = Not(x=w2359) -> (.not. x?=w2366:bool)
                n1511 = property on="RESULT LAB04-2" class="Bool (strict)"("Visible"=w2365) -> ()  [unwired: 2 in, 2 out]
                n1512 = Not(x=w2358) -> (.not. x?=w2367:bool)
                n1513 = property on="RESULT LAB04-1" class="Bool (strict)"("Visible"=w2366) -> ()  [unwired: 2 in, 2 out]
                n1514 = property on="RESULT LAB03-2" class="Bool (strict)"("Visible"=w2367) -> ()  [unwired: 2 in, 2 out]
              }
              frame #2 {
                # "disable calibrate if any test running"
                n1515 = Or(x=w2389, y=w2388) -> (x .or. y?=w2382:bool)
                n1516 = Or(x=w2391, y=w2390) -> (x .or. y?=w2384:bool)
                n1517 = Or(x=w2395, y=w2394) -> (x .or. y?=w2386:bool)
                n1518 = Or(x=w2393, y=w2392) -> (x .or. y?=w2385:bool)
                n1519 = Or(x=w2397, y=w2396) -> (x .or. y?=w2387:bool)
                n1520 = Or(x=w2385, y=w2384) -> (x .or. y?=w2383:bool)
                n1521 = Or(x=w2387, y=w2386) -> (x .or. y?=w2381:bool)
                n1522 = Or(x=w2383, y=w2382) -> (x .or. y?=w2380:bool)
                n1523 = Or(x=w2381, y=w2380) -> (x .or. y?=w2379:bool)
                n1524 = case shown="False" w2379 {
                  tunnel: [0 2] -> w2378
                  frame False {
                  }
                  frame True {
                  }
                }
                n1525 = property on="TO (string):" class="Str"("DisabledEnum"=w2378) -> ()  [unwired: 2 in, 2 out]
                n1526 = property on="Network Directory" class="Path"("DisabledEnum"=w2378) -> ()  [unwired: 2 in, 2 out]
                n1527 = property on="MAIL SETTINGS" class="Clust (strict)"("DisabledEnum"=w2378) -> ()  [unwired: 2 in, 2 out]
                n1528 = property on="CALIBRATE" class="Bool (strict)"("DisabledEnum"=w2378) -> ()  [unwired: 2 in, 2 out]
                n1529 = property on="SHOW ADMIN PAGE" class="Bool (strict)"("DisabledEnum"=w2378) -> ()  [unwired: 2 in, 2 out]
              }
            }
          }
          frame #8 {
            # "drive jigs"
            n1530 = stacked-sequence {
              frame #0 {
                # "jig on"
                n1531 = local read "jig cycle"() -> (w2400:dbl)
                n1532 = Equal?(x=w2400, y=0) -> (x = y?=w2402:bool)
                n1533 = case shown="True" w2402 {
                  frame False {
                  }
                  frame True {
                    n1534 = local read "RUN LAB01-1"() -> (w2403:bool)
                    n1535 = local read "RUN LAB01-2"() -> (w2404:bool)
                    n1536 = local read "RUN LAB03-1"() -> (w2410:bool)
                    n1537 = local read "RUN LAB03-2"() -> (w2409:bool)
                    n1538 = local read "RUN LAB02-1"() -> (w2412:bool)
                    n1539 = local read "RUN LAB02-2"() -> (w2411:bool)
                    n1540 = local read "RUN LAB04-1"() -> (w2408:bool)
                    n1541 = local read "RUN LAB04-2"() -> (w2407:bool)
                    n1542 = local read "RUN LAB05-1"() -> (w2406:bool)
                    n1543 = local read "RUN LAB05-2"() -> (w2405:bool)
                    n1544 = local write "JIG LAB05-1"(w2406) -> ()
                    n1545 = local write "JIG LAB05-2"(w2405) -> ()
                    n1546 = local write "JIG LAB04-2"(w2407) -> ()
                    n1547 = local write "JIG LAB02-1"(w2412) -> ()
                    n1548 = local write "JIG LAB03-1"(w2410) -> ()
                    n1549 = local write "JIG LAB04-1"(w2408) -> ()
                    n1550 = local write "JIG LAB03-2"(w2409) -> ()
                    n1551 = local write "JIG LAB02-2"(w2411) -> ()
                    n1552 = local write "JIG LAB01-1"(w2403) -> ()
                    n1553 = local write "JIG LAB01-2"(w2404) -> ()
                  }
                }
              }
              frame #1 {
                # "jig off"
                n1554 = local read "jig cycle"() -> (w2415:dbl)
                n1555 = local read "on loops"() -> (w2414:dbl)
                n1556 = Equal?(x=w2415, y=w2414) -> (x = y?=w2413:bool)
                n1557 = case shown="True" w2413 {
                  frame False {
                  }
                  frame True {
                    w2466 = FALSE
                    w2467 = TRUE
                    w2465 = 2
                    n1558 = local read "SELECT LAB05-2"() -> (w2456:T3)
                    n1559 = local read "SELECT LAB04-2"() -> (w2458:T3)
                    n1560 = local read "SELECT LAB04-1"() -> (w2459:T3)
                    n1561 = local read "SELECT LAB05-1"() -> (w2457:T3)
                    n1562 = local read "SELECT LAB03-2"() -> (w2460:T3)
                    n1563 = local read "SELECT LAB02-1"() -> (w2463:T3)
                    n1564 = local read "SELECT LAB03-1"() -> (w2461:T3)
                    n1565 = local read "SELECT LAB02-2"() -> (w2462:T3)
                    n1566 = local read "SELECT LAB01-2"() -> (w2464:T3)
                    n1567 = local read "RUN LAB05-1"() -> (w2426:bool)
                    n1568 = local read "RUN LAB05-2"() -> (w2425:bool)
                    n1569 = local read "RUN LAB04-2"() -> (w2427:bool)
                    n1570 = local read "RUN LAB04-1"() -> (w2428:bool)
                    n1571 = local read "RUN LAB01-1"() -> (w2444:bool)
                    n1572 = local read "RUN LAB01-2"() -> (w2433:bool)
                    n1573 = local read "RUN LAB03-2"() -> (w2429:bool)
                    n1574 = local read "SELECT LAB01-1"() -> (w2468:T3)
                    n1575 = local read "RUN LAB03-1"() -> (w2430:bool)
                    n1576 = local read "RUN LAB02-1"() -> (w2432:bool)
                    n1577 = local read "RUN LAB02-2"() -> (w2431:bool)
                    n1578 = Equal?(x=w2465, y=w2461) -> (x = y?=w2439:bool)
                    n1579 = Equal?(x=w2465, y=w2460) -> (x = y?=w2438:bool)
                    n1580 = Equal?(x=w2465, y=w2459) -> (x = y?=w2437:bool)
                    n1581 = Equal?(x=w2465, y=w2458) -> (x = y?=w2436:bool)
                    n1582 = Equal?(x=w2465, y=w2457) -> (x = y?=w2435:bool)
                    n1583 = Equal?(x=w2465, y=w2456) -> (x = y?=w2434:bool)
                    n1584 = Equal?(x=w2465, y=w2468) -> (x = y?=w2445:bool)
                    n1585 = Equal?(x=w2465, y=w2463) -> (x = y?=w2441:bool)
                    n1586 = Equal?(x=w2465, y=w2462) -> (x = y?=w2440:bool)
                    n1587 = Equal?(x=w2465, y=w2464) -> (x = y?=w2442:bool)
                    n1588 = And(x=w2436, y=w2427) -> (x .and. y?=w2418:bool)
                    n1589 = And(x=w2439, y=w2430) -> (x .and. y?=w2421:bool)
                    n1590 = And(x=w2437, y=w2428) -> (x .and. y?=w2419:bool)
                    n1591 = And(x=w2434, y=w2425) -> (x .and. y?=w2416:bool)
                    n1592 = And(x=w2440, y=w2431) -> (x .and. y?=w2422:bool)
                    n1593 = And(x=w2438, y=w2429) -> (x .and. y?=w2420:bool)
                    n1594 = And(x=w2435, y=w2426) -> (x .and. y?=w2417:bool)
                    n1595 = And(x=w2442, y=w2433) -> (x .and. y?=w2424:bool)
                    n1596 = And(x=w2445, y=w2444) -> (x .and. y?=w2443:bool)
                    n1597 = And(x=w2441, y=w2432) -> (x .and. y?=w2423:bool)
                    n1598 = Select(t=w2467, s=w2443, f=w2466) -> (s? t:f=w2446:bool)
                    n1599 = Select(t=w2467, s=w2424, f=w2466) -> (s? t:f=w2447:bool)
                    n1600 = Select(t=w2467, s=w2423, f=w2466) -> (s? t:f=w2448:bool)
                    n1601 = Select(t=w2467, s=w2422, f=w2466) -> (s? t:f=w2449:bool)
                    n1602 = Select(t=w2467, s=w2421, f=w2466) -> (s? t:f=w2450:bool)
                    n1603 = Select(t=w2467, s=w2420, f=w2466) -> (s? t:f=w2451:bool)
                    n1604 = Select(t=w2467, s=w2419, f=w2466) -> (s? t:f=w2452:bool)
                    n1605 = Select(t=w2467, s=w2418, f=w2466) -> (s? t:f=w2453:bool)
                    n1606 = Select(t=w2467, s=w2417, f=w2466) -> (s? t:f=w2454:bool)
                    n1607 = Select(t=w2467, s=w2416, f=w2466) -> (s? t:f=w2455:bool)
                    n1608 = local write "JIG LAB03-2"(w2451) -> ()
                    n1609 = local write "JIG LAB02-1"(w2448) -> ()
                    n1610 = local write "JIG LAB02-2"(w2449) -> ()
                    n1611 = local write "JIG LAB01-2"(w2447) -> ()
                    n1612 = local write "JIG LAB03-1"(w2450) -> ()
                    n1613 = local write "JIG LAB01-1"(w2446) -> ()
                    n1614 = local write "JIG LAB05-2"(w2455) -> ()
                    n1615 = local write "JIG LAB04-1"(w2452) -> ()
                    n1616 = local write "JIG LAB05-1"(w2454) -> ()
                    n1617 = local write "JIG LAB04-2"(w2453) -> ()
                  }
                }
              }
            }
          }
          frame #9 {
            # "drive digital output"
            n1618 = local read "O/I  LAB05-2"() -> (w2474:bool)
            n1619 = local read "O/I  LAB05-1"() -> (w2476:bool)
            n1620 = local read "JIG LAB05-2"() -> (w2473:bool)
            n1621 = local read "O/I  LAB04-2"() -> (w2478:bool)
            n1622 = local read "JIG LAB05-1"() -> (w2475:bool)
            n1623 = local read "JIG LAB04-2"() -> (w2477:bool)
            n1624 = local read "O/I  LAB03-1"() -> (w2483:bool)
            n1625 = local read "O/I  LAB04-1"() -> (w2479:bool)
            n1626 = local read "O/I  LAB02-1"() -> (w2487:bool)
            n1627 = local read "O/I  LAB02-2"() -> (w2485:bool)
            n1628 = local read "O/I  LAB03-2"() -> (w2481:bool)
            n1629 = local read "JIG LAB04-1"() -> (w2472:bool)
            n1630 = local read "JIG LAB03-2"() -> (w2480:bool)
            n1631 = local read "O/I  LAB01-2"() -> (w2489:bool)
            n1632 = local read "JIG LAB02-1"() -> (w2486:bool)
            n1633 = local read "JIG LAB02-2"() -> (w2484:bool)
            n1634 = local read "JIG LAB03-1"() -> (w2482:bool)
            n1635 = local read "O/I  LAB01-1"() -> (w2491:bool)
            n1636 = local read "JIG LAB01-2"() -> (w2488:bool)
            n1637 = local read "JIG LAB01-1"() -> (w2490:bool)
            n1638 = Build Array(w2478, w2477, w2476, w2475, w2474, w2473) -> (w2469:bool[])
            n1639 = Build Array(w2484, w2483, w2482, w2481, w2480, w2479, w2472) -> (w2470:bool[])
            n1640 = Build Array(w2491, w2490, w2489, w2488, w2487, w2486, w2485) -> (w2471:bool[])
            n1641 = call "sub vi - Drive Relays All v6.vi"("Array #2"=w2469, "Array #1"=w2470, "Array #0"=w2471) -> ()  [unwired: 8 in, 1 out]
          }
          frame #10 {
            # "get temperature values"
            n1642 = stacked-sequence {
              frame #0 {
                n1643 = local read "jig cycle"() -> (w2492:dbl)
                n1644 = local read "on loops"() -> (w2495:dbl)
                n1645 = local read "jig cycle"() -> (w2497:dbl)
                n1646 = Add(x=w2495, y=2) -> (x+y=w2496:dbl)
                n1647 = Equal?(x=w2497, y=0) -> (x = y?=w2498:bool)
                n1648 = Equal?(x=w2492, y=w2496) -> (x = y?=w2493:bool)
                n1649 = case shown="True" w2498 {
                  frame False {
                  }
                  frame True {
                    w2510 = FALSE
                    w2511 = TRUE
                    n1650 = local write "TEMP update"(TRUE) -> ()
                    n1651 = call "sub vi - GET ALL TEMP v3.vi"("LA01-EN"=w2511, "LA02-EN"=w2511, "LA03-EN"=w2511, "LA04-EN"=w2510, "LA05-EN"=w2510, "Gen Cal Value"=1.0) -> ("LA01 TEMP"=w2509:T19, "LA02 TEMP"=w2507:T19, "LA03 TEMP"=w2506:T19)  [unwired: 4 in, 3 out]
                    n1652 = local write "LAB03 TEMP"(w2506) -> ()
                    n1653 = local write "LAB02 TEMP"(w2507) -> ()
                    n1654 = local write "LAB01 TEMP"(w2509) -> ()
                  }
                }
                n1655 = case shown="True" w2493 {
                  frame False {
                  }
                  frame True {
                    w2503 = TRUE
                    w2504 = FALSE
                    n1656 = local write "TEMP update"(TRUE) -> ()
                    n1657 = call "sub vi - GET ALL TEMP v3.vi"("LA01-EN"=w2504, "LA02-EN"=w2504, "LA03-EN"=w2504, "LA04-EN"=w2503, "LA05-EN"=w2503, "Gen Cal Value"=1.0) -> ("LA04 TEMP"=w2501:T19, "LA05 TEMP"=w2500:T19)  [unwired: 4 in, 4 out]
                    n1658 = local write "LAB04 TEMP"(w2501) -> ()
                    n1659 = local write "LAB05 TEMP"(w2500) -> ()
                  }
                }
              }
              frame #1 {
                n1660 = local read "CAL LAB01"() -> (w2529:T7)
                n1661 = local read "LAB01 TEMP"() -> (w2530:T10)
                n1662 = Unbundle By Name(w2530) -> ("T1 Live"=w2520:dbl, "T1 Neut"=w2519:dbl, "T2 Live"=w2518:dbl, "T2 Neut"=w2517:dbl)  [unwired: 2 out]
                n1663 = Unbundle By Name(w2529) -> ("1 (TL) cal"=w2516:dbl, "1 (TN) cal"=w2515:dbl, "2 (TL) cal"=w2514:dbl, "2 (TN) cal"=w2513:dbl)  [unwired: 6 out]
                n1664 = Multiply(x=w2520, y=w2516) -> (x*y=w2526:dbl)
                n1665 = Multiply(x=w2519, y=w2515) -> (x*y=w2525:dbl)
                n1666 = Multiply(x=w2518, y=w2514) -> (x*y=w2522:dbl)
                n1667 = Multiply(x=w2517, y=w2513) -> (x*y=w2521:dbl)
                n1668 = local read "SIG LAB01-2"() -> (w2524:T2)
                n1669 = local read "SIG LAB01-1"() -> (w2528:T2)
                n1670 = Bundle By Name(cluster=w2528, "Tmp Live"=w2526, "Tmp Neut"=w2525) -> (w2527:T2)
                n1671 = Bundle By Name(cluster=w2524, "Tmp Live"=w2522, "Tmp Neut"=w2521) -> (w2523:T2)
                n1672 = local write "SIG LAB01-1"(w2527) -> ()
                n1673 = local write "SIG LAB01-2"(w2523) -> ()
              }
              frame #2 {
                n1674 = local read "CAL LAB02"() -> (w2547:T8)
                n1675 = local read "LAB02 TEMP"() -> (w2548:T10)
                n1676 = Unbundle By Name(w2548) -> ("T1 Live"=w2538:dbl, "T1 Neut"=w2537:dbl, "T2 Live"=w2536:dbl, "T2 Neut"=w2535:dbl)  [unwired: 2 out]
                n1677 = Unbundle By Name(w2547) -> ("1 (TL) cal"=w2534:dbl, "1 (TN) cal"=w2533:dbl, "2 (TL) cal"=w2532:dbl, "2 (TN) cal"=w2531:dbl)  [unwired: 6 out]
                n1678 = Multiply(x=w2538, y=w2534) -> (x*y=w2544:dbl)
                n1679 = Multiply(x=w2537, y=w2533) -> (x*y=w2543:dbl)
                n1680 = Multiply(x=w2536, y=w2532) -> (x*y=w2540:dbl)
                n1681 = Multiply(x=w2535, y=w2531) -> (x*y=w2539:dbl)
                n1682 = local read "SIG LAB02-2"() -> (w2542:T2)
                n1683 = local read "SIG LAB02-1"() -> (w2546:T2)
                n1684 = Bundle By Name(cluster=w2546, "Tmp Live"=w2544, "Tmp Neut"=w2543) -> (w2545:T2)
                n1685 = Bundle By Name(cluster=w2542, "Tmp Live"=w2540, "Tmp Neut"=w2539) -> (w2541:T2)
                n1686 = local write "SIG LAB02-1"(w2545) -> ()
                n1687 = local write "SIG LAB02-2"(w2541) -> ()
              }
              frame #3 {
                n1688 = local read "CAL LAB03"() -> (w2565:T7)
                n1689 = local read "LAB03 TEMP"() -> (w2566:T10)
                n1690 = Unbundle By Name(w2566) -> ("T1 Live"=w2556:dbl, "T1 Neut"=w2555:dbl, "T2 Live"=w2554:dbl, "T2 Neut"=w2553:dbl)  [unwired: 2 out]
                n1691 = Unbundle By Name(w2565) -> ("1 (TL) cal"=w2552:dbl, "1 (TN) cal"=w2551:dbl, "2 (TL) cal"=w2550:dbl, "2 (TN) cal"=w2549:dbl)  [unwired: 6 out]
                n1692 = Multiply(x=w2556, y=w2552) -> (x*y=w2562:dbl)
                n1693 = Multiply(x=w2555, y=w2551) -> (x*y=w2561:dbl)
                n1694 = Multiply(x=w2554, y=w2550) -> (x*y=w2558:dbl)
                n1695 = Multiply(x=w2553, y=w2549) -> (x*y=w2557:dbl)
                n1696 = local read "SIG LAB03-2"() -> (w2560:T2)
                n1697 = local read "SIG LAB03-1"() -> (w2564:T2)
                n1698 = Bundle By Name(cluster=w2564, "Tmp Live"=w2562, "Tmp Neut"=w2561) -> (w2563:T2)
                n1699 = Bundle By Name(cluster=w2560, "Tmp Live"=w2558, "Tmp Neut"=w2557) -> (w2559:T2)
                n1700 = local write "SIG LAB03-1"(w2563) -> ()
                n1701 = local write "SIG LAB03-2"(w2559) -> ()
              }
              frame #4 {
                n1702 = local read "CAL LAB04"() -> (w2583:T7)
                n1703 = local read "LAB04 TEMP"() -> (w2584:T10)
                n1704 = Unbundle By Name(w2584) -> ("T1 Live"=w2574:dbl, "T1 Neut"=w2573:dbl, "T2 Live"=w2572:dbl, "T2 Neut"=w2571:dbl)  [unwired: 2 out]
                n1705 = Unbundle By Name(w2583) -> ("1 (TL) cal"=w2570:dbl, "1 (TN) cal"=w2569:dbl, "2 (TL) cal"=w2568:dbl, "2 (TN) cal"=w2567:dbl)  [unwired: 6 out]
                n1706 = Multiply(x=w2574, y=w2570) -> (x*y=w2580:dbl)
                n1707 = Multiply(x=w2573, y=w2569) -> (x*y=w2579:dbl)
                n1708 = Multiply(x=w2572, y=w2568) -> (x*y=w2576:dbl)
                n1709 = Multiply(x=w2571, y=w2567) -> (x*y=w2575:dbl)
                n1710 = local read "SIG LAB04-2"() -> (w2578:T2)
                n1711 = local read "SIG LAB04-1"() -> (w2582:T2)
                n1712 = Bundle By Name(cluster=w2582, "Tmp Live"=w2580, "Tmp Neut"=w2579) -> (w2581:T2)
                n1713 = Bundle By Name(cluster=w2578, "Tmp Live"=w2576, "Tmp Neut"=w2575) -> (w2577:T2)
                n1714 = local write "SIG LAB04-1"(w2581) -> ()
                n1715 = local write "SIG LAB04-2"(w2577) -> ()
              }
              frame #5 {
                n1716 = local read "CAL LAB05"() -> (w2601:T7)
                n1717 = local read "LAB05 TEMP"() -> (w2602:T10)
                n1718 = Unbundle By Name(w2602) -> ("T1 Live"=w2592:dbl, "T1 Neut"=w2591:dbl, "T2 Live"=w2590:dbl, "T2 Neut"=w2589:dbl)  [unwired: 2 out]
                n1719 = Unbundle By Name(w2601) -> ("1 (TL) cal"=w2588:dbl, "1 (TN) cal"=w2587:dbl, "2 (TL) cal"=w2586:dbl, "2 (TN) cal"=w2585:dbl)  [unwired: 6 out]
                n1720 = Multiply(x=w2592, y=w2588) -> (x*y=w2598:dbl)
                n1721 = Multiply(x=w2591, y=w2587) -> (x*y=w2597:dbl)
                n1722 = Multiply(x=w2590, y=w2586) -> (x*y=w2594:dbl)
                n1723 = Multiply(x=w2589, y=w2585) -> (x*y=w2593:dbl)
                n1724 = local read "SIG LAB05-2"() -> (w2596:T2)
                n1725 = local read "SIG LAB05-1"() -> (w2600:T2)
                n1726 = Bundle By Name(cluster=w2600, "Tmp Live"=w2598, "Tmp Neut"=w2597) -> (w2599:T2)
                n1727 = Bundle By Name(cluster=w2596, "Tmp Live"=w2594, "Tmp Neut"=w2593) -> (w2595:T2)
                n1728 = local write "SIG LAB05-1"(w2599) -> ()
                n1729 = local write "SIG LAB05-2"(w2595) -> ()
              }
            }
          }
          frame #11 {
            # "get analog values"
            n1730 = local read "on loops"() -> (w2609:dbl)
            n1731 = local read "jig cycle"() -> (w2606:dbl)
            n1732 = Add(x=w2609, y=1) -> (x+y=w2607:dbl)
            n1733 = Equal?(x=w2606, y=1) -> (x = y?=w2604:bool)
            n1734 = Equal?(x=w2606, y=w2607) -> (x = y?=w2605:bool)
            n1735 = Or(x=w2604, y=w2605) -> (x .or. y?=w2603:bool)
            n1736 = case shown="True" w2603 {
              frame False {
              }
              frame True {
                n1737 = call "sub vi - Read Analog All v8.vi"() -> ("Analog loop time"=w2617:dbl, "array GRAPH"=w2616:dynamicdata[], "LAB01"=w2615:T20, "LAB02"=w2614:T21, "LAB03"=w2613:T22, "LAB04"=w2612:T23, "array ERROR"=w2618:errorcluster[], "LAB05"=w2611:T24)  [unwired: 8 in]
                n1738 = stacked-sequence {
                  tunnel: w2618 -> [w2621 _ _ _ _ _]
                  tunnel: w2617 -> [w2620 _ _ _ _ _]
                  tunnel: w2616 -> [w2619 _ _ _ _ _]
                  tunnel: w2615 -> [_ w2666 _ _ _ _]
                  tunnel: w2614 -> [_ _ w2667 _ _ _]
                  tunnel: w2613 -> [_ _ _ w2692 _ _]
                  tunnel: w2612 -> [_ _ _ _ w2715 _]
                  tunnel: w2611 -> [_ _ _ _ _ w2740]
                  frame #0 {
                    n1739 = local write "AI update"(TRUE) -> ()
                    n1740 = Index Array(array=w2619, index=6) -> (element=→"LAB04-1 (GRAPH)":dynamicdata)
                    n1741 = Index Array(array=w2619, index=7) -> (element=→"LAB04-2 (GRAPH)":dynamicdata)
                    n1742 = Index Array(array=w2619, index=9) -> (element=→"LAB05-2 (GRAPH)":dynamicdata)
                    n1743 = Index Array(array=w2619, index=8) -> (element=→"LAB05-1 (GRAPH)":dynamicdata)
                    n1744 = Index Array(array=w2619, index=5) -> (element=→"LAB03-2 (GRAPH)":dynamicdata)
                    n1745 = Index Array(array=w2619, index=0) -> (element=→"LAB01-1 (GRAPH)":dynamicdata)
                    n1746 = Index Array(array=w2619, index=1) -> (element=→"LAB01-2 (GRAPH)":dynamicdata)
                    n1747 = Index Array(array=w2619, index=2) -> (element=→"LAB02-1 (GRAPH)":dynamicdata)
                    n1748 = Index Array(array=w2619, index=3) -> (element=→"LAB02-2 (GRAPH)":dynamicdata)
                    n1749 = Index Array(array=w2619, index=4) -> (element=→"LAB03-1 (GRAPH)":dynamicdata)
                    "AI loop time" <- w2620
                    "Analog Error Array" <- w2621
                  }
                  frame #1 {
                    n1750 = local read "CAL LAB01"() -> (w2665:T7)
                    n1751 = Unbundle By Name(w2666) -> ("LAB01-1 (A)"=w2664:dbl, "LAB01-1 (V)"=w2663:dbl, "LAB01-1 (PF)"=w2662:dbl, "LAB01-2 (A)"=w2661:dbl, "LAB01-2 (V)"=w2660:dbl, "LAB01-2 (PF)"=w2659:dbl)
                    n1752 = Unbundle By Name(w2665) -> ("1  (A) cal"=w2658:dbl, "1 (V) cal"=w2657:dbl, "1 (PF) cal"=w2656:dbl, "2 (A) cal"=w2655:dbl, "2 (V) cal"=w2654:dbl, "2 (PF) cal"=w2653:dbl)  [unwired: 4 out]
                    n1753 = Multiply(x=w2664, y=w2658) -> (x*y=w2651:dbl)
                    n1754 = Multiply(x=w2663, y=w2657) -> (x*y=w2650:dbl)
                    n1755 = Multiply(x=w2662, y=w2656) -> (x*y=w2649:dbl)
                    n1756 = Multiply(x=w2661, y=w2655) -> (x*y=w2645:dbl)
                    n1757 = Multiply(x=w2660, y=w2654) -> (x*y=w2644:dbl)
                    n1758 = Multiply(x=w2659, y=w2653) -> (x*y=w2643:dbl)
                    n1759 = local read "SIG LAB01-1"() -> (w2652:T2)
                    n1760 = local read "SIG LAB01-2"() -> (w2647:T2)
                    n1761 = Bundle By Name(cluster=w2652, "AMPS"=w2651, "VOLTS"=w2650, "PF"=w2649) -> (w2648:T2)
                    n1762 = Bundle By Name(cluster=w2647, "AMPS"=w2645, "VOLTS"=w2644, "PF"=w2643) -> (w2646:T2)
                    n1763 = local write "SIG LAB01-2"(w2646) -> ()
                    n1764 = local write "SIG LAB01-1"(w2648) -> ()
                  }
                  frame #2 {
                    n1765 = local read "CAL LAB02"() -> (w2690:T8)
                    n1766 = Unbundle By Name(w2667) -> ("LAB02-1 (A)"=w2689:dbl, "LAB02-1 (V)"=w2688:dbl, "LAB02-1 (PF)"=w2687:dbl, "LAB02-2 (A)"=w2686:dbl, "LAB02-2 (V)"=w2685:dbl, "LAB02-2 (PF)"=w2684:dbl)
                    n1767 = Unbundle By Name(w2690) -> ("1 (A) cal"=w2683:dbl, "1 (V) cal"=w2682:dbl, "1 (PF) cal"=w2681:dbl, "2 (A) cal"=w2680:dbl, "2 (V) cal"=w2679:dbl, "2 (PF) cal"=w2678:dbl)  [unwired: 4 out]
                    n1768 = Multiply(x=w2689, y=w2683) -> (x*y=w2676:dbl)
                    n1769 = Multiply(x=w2688, y=w2682) -> (x*y=w2675:dbl)
                    n1770 = Multiply(x=w2687, y=w2681) -> (x*y=w2674:dbl)
                    n1771 = Multiply(x=w2686, y=w2680) -> (x*y=w2670:dbl)
                    n1772 = Multiply(x=w2685, y=w2679) -> (x*y=w2669:dbl)
                    n1773 = Multiply(x=w2684, y=w2678) -> (x*y=w2668:dbl)
                    n1774 = local read "SIG LAB02-1"() -> (w2677:T2)
                    n1775 = local read "SIG LAB02-2"() -> (w2672:T2)
                    n1776 = Bundle By Name(cluster=w2677, "AMPS"=w2676, "VOLTS"=w2675, "PF"=w2674) -> (w2673:T2)
                    n1777 = Bundle By Name(cluster=w2672, "AMPS"=w2670, "VOLTS"=w2669, "PF"=w2668) -> (w2671:T2)
                    n1778 = local write "SIG LAB02-2"(w2671) -> ()
                    n1779 = local write "SIG LAB02-1"(w2673) -> ()
                  }
                  frame #3 {
                    n1780 = local read "CAL LAB03"() -> (w2714:T7)
                    n1781 = Unbundle By Name(w2692) -> ("LAB03-1 (A)"=w2713:dbl, "LAB03-1 (V)"=w2712:dbl, "LAB03-1 (PF)"=w2711:dbl, "LAB03-2 (A)"=w2710:dbl, "LAB03-2 (V)"=w2709:dbl, "LAB03-2 (PF)"=w2708:dbl)
                    n1782 = Unbundle By Name(w2714) -> ("1  (A) cal"=w2707:dbl, "1 (V) cal"=w2706:dbl, "1 (PF) cal"=w2705:dbl, "2 (A) cal"=w2704:dbl, "2 (V) cal"=w2703:dbl, "2 (PF) cal"=w2702:dbl)  [unwired: 4 out]
                    n1783 = Multiply(x=w2713, y=w2707) -> (x*y=w2700:dbl)
                    n1784 = Multiply(x=w2712, y=w2706) -> (x*y=w2691:dbl)
                    n1785 = Multiply(x=w2711, y=w2705) -> (x*y=w2699:dbl)
                    n1786 = Multiply(x=w2710, y=w2704) -> (x*y=w2695:dbl)
                    n1787 = Multiply(x=w2709, y=w2703) -> (x*y=w2694:dbl)
                    n1788 = Multiply(x=w2708, y=w2702) -> (x*y=w2693:dbl)
                    n1789 = local read "SIG LAB03-1"() -> (w2701:T2)
                    n1790 = local read "SIG LAB03-2"() -> (w2697:T2)
                    n1791 = Bundle By Name(cluster=w2701, "AMPS"=w2700, "VOLTS"=w2691, "PF"=w2699) -> (w2698:T2)
                    n1792 = Bundle By Name(cluster=w2697, "AMPS"=w2695, "VOLTS"=w2694, "PF"=w2693) -> (w2696:T2)
                    n1793 = local write "SIG LAB03-2"(w2696) -> ()
                    n1794 = local write "SIG LAB03-1"(w2698) -> ()
                  }
                  frame #4 {
                    n1795 = local read "CAL LAB04"() -> (w2738:T7)
                    n1796 = Unbundle By Name(w2715) -> ("LAB04-1 (A)"=w2737:dbl, "LAB04-1 (V)"=w2736:dbl, "LAB04-1 (PF)"=w2735:dbl, "LAB04-2 (A)"=w2734:dbl, "LAB04-2 (V)"=w2733:dbl, "LAB04-2 (PF)"=w2732:dbl)
                    n1797 = Unbundle By Name(w2738) -> ("1  (A) cal"=w2731:dbl, "1 (V) cal"=w2730:dbl, "1 (PF) cal"=w2729:dbl, "2 (A) cal"=w2728:dbl, "2 (V) cal"=w2727:dbl, "2 (PF) cal"=w2726:dbl)  [unwired: 4 out]
                    n1798 = Multiply(x=w2737, y=w2731) -> (x*y=w2724:dbl)
                    n1799 = Multiply(x=w2736, y=w2730) -> (x*y=w2723:dbl)
                    n1800 = Multiply(x=w2735, y=w2729) -> (x*y=w2722:dbl)
                    n1801 = Multiply(x=w2734, y=w2728) -> (x*y=w2718:dbl)
                    n1802 = Multiply(x=w2733, y=w2727) -> (x*y=w2717:dbl)
                    n1803 = Multiply(x=w2732, y=w2726) -> (x*y=w2716:dbl)
                    n1804 = local read "SIG LAB04-1"() -> (w2725:T2)
                    n1805 = local read "SIG LAB04-2"() -> (w2720:T2)
                    n1806 = Bundle By Name(cluster=w2725, "AMPS"=w2724, "VOLTS"=w2723, "PF"=w2722) -> (w2721:T2)
                    n1807 = Bundle By Name(cluster=w2720, "AMPS"=w2718, "VOLTS"=w2717, "PF"=w2716) -> (w2719:T2)
                    n1808 = local write "SIG LAB04-2"(w2719) -> ()
                    n1809 = local write "SIG LAB04-1"(w2721) -> ()
                  }
                  frame #5 {
                    n1810 = local read "CAL LAB05"() -> (w2762:T7)
                    n1811 = Unbundle By Name(w2740) -> ("LAB05-1 (A)"=w2761:dbl, "LAB05-1 (V)"=w2739:dbl, "LAB05-1 (PF)"=w2760:dbl, "LAB05-2 (A)"=w2759:dbl, "LAB05-2 (V)"=w2758:dbl, "LAB05-2 (PF)"=w2757:dbl)
                    n1812 = Unbundle By Name(w2762) -> ("1  (A) cal"=w2756:dbl, "1 (V) cal"=w2755:dbl, "1 (PF) cal"=w2754:dbl, "2 (A) cal"=w2753:dbl, "2 (V) cal"=w2752:dbl, "2 (PF) cal"=w2751:dbl)  [unwired: 4 out]
                    n1813 = Multiply(x=w2761, y=w2756) -> (x*y=w2749:dbl)
                    n1814 = Multiply(x=w2739, y=w2755) -> (x*y=w2748:dbl)
                    n1815 = Multiply(x=w2760, y=w2754) -> (x*y=w2747:dbl)
                    n1816 = Multiply(x=w2759, y=w2753) -> (x*y=w2743:dbl)
                    n1817 = Multiply(x=w2758, y=w2752) -> (x*y=w2742:dbl)
                    n1818 = Multiply(x=w2757, y=w2751) -> (x*y=w2741:dbl)
                    n1819 = local read "SIG LAB05-1"() -> (w2750:T2)
                    n1820 = local read "SIG LAB05-2"() -> (w2745:T2)
                    n1821 = Bundle By Name(cluster=w2750, "AMPS"=w2749, "VOLTS"=w2748, "PF"=w2747) -> (w2746:T2)
                    n1822 = Bundle By Name(cluster=w2745, "AMPS"=w2743, "VOLTS"=w2742, "PF"=w2741) -> (w2744:T2)
                    n1823 = local write "SIG LAB05-2"(w2744) -> ()
                    n1824 = local write "SIG LAB05-1"(w2746) -> ()
                  }
                }
              }
            }
          }
          frame #12 {
            # "save test data to file"
            n1825 = local read "on loops"() -> (w2779:dbl)
            n1826 = local read "jig cycle"() -> (w2776:dbl)
            n1827 = Add(x=w2779, y=2) -> (x+y=w2777:dbl)
            n1828 = Equal?(x=w2776, y=1) -> (x = y?=w2774:bool)
            n1829 = Equal?(x=w2776, y=w2777) -> (x = y?=w2775:bool)
            n1830 = Or(x=w2774, y=w2775) -> (x .or. y?=w2773:bool)
            n1831 = case shown="True" w2773 {
              tunnel: w2772 -> [_ w2790]
              tunnel: w2771 -> [_ w2789]
              tunnel: w2770 -> [_ w2788]
              tunnel: w2769 -> [_ w2787]
              tunnel: w2768 -> [_ w2786]
              tunnel: w2767 -> [_ w2785]
              tunnel: w2766 -> [_ w2784]
              tunnel: w2765 -> [_ w2783]
              tunnel: w2764 -> [_ w2782]
              tunnel: w2763 -> [_ w2781]
              frame False {
              }
              frame True {
                n1832 = stacked-sequence {
                  tunnel: w2790 -> [w2791 _ _ _ _ _ _ _ _ _]
                  tunnel: w2789 -> [_ w2836 _ _ _ _ _ _ _ _]
                  tunnel: w2788 -> [_ _ w2881 _ _ _ _ _ _ _]
                  tunnel: w2787 -> [_ _ _ w2926 _ _ _ _ _ _]
                  tunnel: w2786 -> [_ _ _ _ w2971 _ _ _ _ _]
                  tunnel: w2785 -> [_ _ _ _ _ w3016 _ _ _ _]
                  tunnel: w2784 -> [_ _ _ _ _ _ w3061 _ _ _]
                  tunnel: w2783 -> [_ _ _ _ _ _ _ w3106 _ _]
                  tunnel: w2782 -> [_ _ _ _ _ _ _ _ w3151 _]
                  tunnel: w2781 -> [_ _ _ _ _ _ _ _ _ w3196]
                  frame #0 {
                    # "LAB01-1"
                    n1833 = case shown="True" w2791 {
                      frame False {
                      }
                      frame True {
                        n1834 = local read "DISP LAB01-1"() -> (w2792:T4)
                        n1835 = local read "SIG LAB01-1"() -> (w2793:T2)
                        n1836 = local read "TDMS LAB01-1"() -> (w2835:refnum<k34>)
                        n1837 = Build Array("TEMP Neut") -> (w2801:string[])
                        n1838 = Build Array("CYCLE") -> (w2796:string[])
                        n1839 = Build Array("TEMP Live") -> (w2806:string[])
                        n1840 = Build Array("PF") -> (w2811:string[])
                        n1841 = Build Array("AMPS") -> (w2832:string[])
                        n1842 = Build Array("VOLTS") -> (w2823:string[])
                        n1843 = Unbundle(w2793) -> ("AMPS"=w2831:dbl, "VOLTS"=w2820:dbl, "PF"=w2819:dbl, "Tmp Live"=w2818:dbl, "Tmp Neut"=w2821:dbl)
                        n1844 = Unbundle(w2792) -> ("CYCLE"=w2816:dbl)  [unwired: 2 out]
                        n1845 = Build Array(w2820) -> (w2817:dbl[])
                        n1846 = Build Array(w2819) -> (w2810:dbl[])
                        n1847 = Build Array(w2818) -> (w2805:dbl[])
                        n1848 = Build Array(w2821) -> (w2800:dbl[])
                        n1849 = Build Array(w2831) -> (w2830:dbl[])
                        n1850 = Build Array(w2816) -> (w2795:dbl[])
                        n1851 = TDMS Write(0:w2835, 5:"LAB01-1 TEST VALUES", 7:w2832, 9:w2830) -> (4:w2825:refnum<k34>, 6:w2824:string, 15:w2812:errorcluster)  [unwired: 2 in, 1 out]
                        n1852 = TDMS Write(0:w2825, 5:w2824, 7:w2823, 9:w2817, 11:w2812) -> (4:w2815:refnum<k34>, 6:w2814:string, 15:w2813:errorcluster)  [unwired: 1 in, 1 out]
                        n1853 = TDMS Write(0:w2815, 5:w2814, 7:w2811, 9:w2810, 11:w2813) -> (4:w2809:refnum<k34>, 6:w2808:string, 15:w2807:errorcluster)  [unwired: 1 in, 1 out]
                        n1854 = TDMS Write(0:w2809, 5:w2808, 7:w2806, 9:w2805, 11:w2807) -> (4:w2804:refnum<k34>, 6:w2803:string, 15:w2802:errorcluster)  [unwired: 1 in, 1 out]
                        n1855 = TDMS Write(0:w2804, 5:w2803, 7:w2801, 9:w2800, 11:w2802) -> (4:w2799:refnum<k34>, 6:w2798:string, 15:w2797:errorcluster)  [unwired: 1 in, 1 out]
                        n1856 = TDMS Write(0:w2799, 5:w2798, 7:w2796, 9:w2795, 11:w2797) -> (15:w2794:errorcluster)  [unwired: 1 in, 3 out]
                        n1857 = local write "data file error"(w2794) -> ()
                      }
                    }
                  }
                  frame #1 {
                    # "LAB01-2"
                    n1858 = case shown="True" w2836 {
                      frame False {
                      }
                      frame True {
                        n1859 = local read "DISP LAB01-2"() -> (w2878:T4)
                        n1860 = local read "SIG LAB01-2"() -> (w2879:T2)
                        n1861 = local read "TDMS LAB01-2"() -> (w2880:refnum<k34>)
                        n1862 = Build Array("TEMP Neut") -> (w2844:string[])
                        n1863 = Build Array("CYCLE") -> (w2839:string[])
                        n1864 = Build Array("TEMP Live") -> (w2849:string[])
                        n1865 = Build Array("PF") -> (w2854:string[])
                        n1866 = Build Array("AMPS") -> (w2875:string[])
                        n1867 = Build Array("VOLTS") -> (w2866:string[])
                        n1868 = Unbundle(w2879) -> ("AMPS"=w2874:dbl, "VOLTS"=w2863:dbl, "PF"=w2862:dbl, "Tmp Live"=w2861:dbl, "Tmp Neut"=w2864:dbl)
                        n1869 = Unbundle(w2878) -> ("CYCLE"=w2859:dbl)  [unwired: 2 out]
                        n1870 = Build Array(w2863) -> (w2860:dbl[])
                        n1871 = Build Array(w2862) -> (w2853:dbl[])
                        n1872 = Build Array(w2861) -> (w2848:dbl[])
                        n1873 = Build Array(w2864) -> (w2843:dbl[])
                        n1874 = Build Array(w2874) -> (w2873:dbl[])
                        n1875 = Build Array(w2859) -> (w2838:dbl[])
                        n1876 = TDMS Write(0:w2880, 5:"LAB01-2 TEST VALUES", 7:w2875, 9:w2873) -> (4:w2868:refnum<k34>, 6:w2867:string, 15:w2855:errorcluster)  [unwired: 2 in, 1 out]
                        n1877 = TDMS Write(0:w2868, 5:w2867, 7:w2866, 9:w2860, 11:w2855) -> (4:w2858:refnum<k34>, 6:w2857:string, 15:w2856:errorcluster)  [unwired: 1 in, 1 out]
                        n1878 = TDMS Write(0:w2858, 5:w2857, 7:w2854, 9:w2853, 11:w2856) -> (4:w2852:refnum<k34>, 6:w2851:string, 15:w2850:errorcluster)  [unwired: 1 in, 1 out]
                        n1879 = TDMS Write(0:w2852, 5:w2851, 7:w2849, 9:w2848, 11:w2850) -> (4:w2847:refnum<k34>, 6:w2846:string, 15:w2845:errorcluster)  [unwired: 1 in, 1 out]
                        n1880 = TDMS Write(0:w2847, 5:w2846, 7:w2844, 9:w2843, 11:w2845) -> (4:w2842:refnum<k34>, 6:w2841:string, 15:w2840:errorcluster)  [unwired: 1 in, 1 out]
                        n1881 = TDMS Write(0:w2842, 5:w2841, 7:w2839, 9:w2838, 11:w2840) -> (15:w2837:errorcluster)  [unwired: 1 in, 3 out]
                        n1882 = local write "data file error"(w2837) -> ()
                      }
                    }
                  }
                  frame #2 {
                    # "LAB02-1"
                    n1883 = case shown="True" w2881 {
                      frame False {
                      }
                      frame True {
                        n1884 = local read "DISP LAB02-1"() -> (w2923:T4)
                        n1885 = local read "SIG LAB02-1"() -> (w2924:T2)
                        n1886 = local read "TDMS LAB02-1"() -> (w2925:refnum<k34>)
                        n1887 = Build Array("TEMP Neut") -> (w2889:string[])
                        n1888 = Build Array("CYCLE") -> (w2884:string[])
                        n1889 = Build Array("TEMP Live") -> (w2894:string[])
                        n1890 = Build Array("PF") -> (w2899:string[])
                        n1891 = Build Array("AMPS") -> (w2920:string[])
                        n1892 = Build Array("VOLTS") -> (w2911:string[])
                        n1893 = Unbundle(w2924) -> ("AMPS"=w2919:dbl, "VOLTS"=w2908:dbl, "PF"=w2907:dbl, "Tmp Live"=w2906:dbl, "Tmp Neut"=w2909:dbl)
                        n1894 = Unbundle(w2923) -> ("CYCLE"=w2904:dbl)  [unwired: 2 out]
                        n1895 = Build Array(w2908) -> (w2905:dbl[])
                        n1896 = Build Array(w2907) -> (w2898:dbl[])
                        n1897 = Build Array(w2906) -> (w2893:dbl[])
                        n1898 = Build Array(w2909) -> (w2888:dbl[])
                        n1899 = Build Array(w2919) -> (w2918:dbl[])
                        n1900 = Build Array(w2904) -> (w2883:dbl[])
                        n1901 = TDMS Write(0:w2925, 5:"LAB02-1 TEST VALUES", 7:w2920, 9:w2918) -> (4:w2913:refnum<k34>, 6:w2912:string, 15:w2900:errorcluster)  [unwired: 2 in, 1 out]
                        n1902 = TDMS Write(0:w2913, 5:w2912, 7:w2911, 9:w2905, 11:w2900) -> (4:w2903:refnum<k34>, 6:w2902:string, 15:w2901:errorcluster)  [unwired: 1 in, 1 out]
                        n1903 = TDMS Write(0:w2903, 5:w2902, 7:w2899, 9:w2898, 11:w2901) -> (4:w2897:refnum<k34>, 6:w2896:string, 15:w2895:errorcluster)  [unwired: 1 in, 1 out]
                        n1904 = TDMS Write(0:w2897, 5:w2896, 7:w2894, 9:w2893, 11:w2895) -> (4:w2892:refnum<k34>, 6:w2891:string, 15:w2890:errorcluster)  [unwired: 1 in, 1 out]
                        n1905 = TDMS Write(0:w2892, 5:w2891, 7:w2889, 9:w2888, 11:w2890) -> (4:w2887:refnum<k34>, 6:w2886:string, 15:w2885:errorcluster)  [unwired: 1 in, 1 out]
                        n1906 = TDMS Write(0:w2887, 5:w2886, 7:w2884, 9:w2883, 11:w2885) -> (15:w2882:errorcluster)  [unwired: 1 in, 3 out]
                        n1907 = local write "data file error"(w2882) -> ()
                      }
                    }
                  }
                  frame #3 {
                    # "LAB02-2"
                    n1908 = case shown="True" w2926 {
                      frame False {
                      }
                      frame True {
                        n1909 = local read "DISP LAB02-2"() -> (w2968:T4)
                        n1910 = local read "SIG LAB02-2"() -> (w2969:T2)
                        n1911 = local read "TDMS LAB02-2"() -> (w2970:refnum<k34>)
                        n1912 = Build Array("TEMP Neut") -> (w2934:string[])
                        n1913 = Build Array("CYCLE") -> (w2929:string[])
                        n1914 = Build Array("TEMP Live") -> (w2939:string[])
                        n1915 = Build Array("PF") -> (w2944:string[])
                        n1916 = Build Array("AMPS") -> (w2965:string[])
                        n1917 = Build Array("VOLTS") -> (w2956:string[])
                        n1918 = Unbundle(w2969) -> ("AMPS"=w2964:dbl, "VOLTS"=w2953:dbl, "PF"=w2952:dbl, "Tmp Live"=w2951:dbl, "Tmp Neut"=w2954:dbl)
                        n1919 = Unbundle(w2968) -> ("CYCLE"=w2949:dbl)  [unwired: 2 out]
                        n1920 = Build Array(w2953) -> (w2950:dbl[])
                        n1921 = Build Array(w2952) -> (w2943:dbl[])
                        n1922 = Build Array(w2951) -> (w2938:dbl[])
                        n1923 = Build Array(w2954) -> (w2933:dbl[])
                        n1924 = Build Array(w2964) -> (w2963:dbl[])
                        n1925 = Build Array(w2949) -> (w2928:dbl[])
                        n1926 = TDMS Write(0:w2970, 5:"LAB02-2 TEST VALUES", 7:w2965, 9:w2963) -> (4:w2958:refnum<k34>, 6:w2957:string, 15:w2945:errorcluster)  [unwired: 2 in, 1 out]
                        n1927 = TDMS Write(0:w2958, 5:w2957, 7:w2956, 9:w2950, 11:w2945) -> (4:w2948:refnum<k34>, 6:w2947:string, 15:w2946:errorcluster)  [unwired: 1 in, 1 out]
                        n1928 = TDMS Write(0:w2948, 5:w2947, 7:w2944, 9:w2943, 11:w2946) -> (4:w2942:refnum<k34>, 6:w2941:string, 15:w2940:errorcluster)  [unwired: 1 in, 1 out]
                        n1929 = TDMS Write(0:w2942, 5:w2941, 7:w2939, 9:w2938, 11:w2940) -> (4:w2937:refnum<k34>, 6:w2936:string, 15:w2935:errorcluster)  [unwired: 1 in, 1 out]
                        n1930 = TDMS Write(0:w2937, 5:w2936, 7:w2934, 9:w2933, 11:w2935) -> (4:w2932:refnum<k34>, 6:w2931:string, 15:w2930:errorcluster)  [unwired: 1 in, 1 out]
                        n1931 = TDMS Write(0:w2932, 5:w2931, 7:w2929, 9:w2928, 11:w2930) -> (15:w2927:errorcluster)  [unwired: 1 in, 3 out]
                        n1932 = local write "data file error"(w2927) -> ()
                      }
                    }
                  }
                  frame #4 {
                    # "LAB03-1"
                    n1933 = case shown="True" w2971 {
                      frame False {
                      }
                      frame True {
                        n1934 = local read "DISP LAB03-1"() -> (w3013:T4)
                        n1935 = local read "SIG LAB03-1"() -> (w3014:T2)
                        n1936 = local read "TDMS LAB03-1"() -> (w3015:refnum<k34>)
                        n1937 = Build Array("TEMP Neut") -> (w2979:string[])
                        n1938 = Build Array("CYCLE") -> (w2974:string[])
                        n1939 = Build Array("TEMP Live") -> (w2984:string[])
                        n1940 = Build Array("PF") -> (w2989:string[])
                        n1941 = Build Array("AMPS") -> (w3010:string[])
                        n1942 = Build Array("VOLTS") -> (w3001:string[])
                        n1943 = Unbundle(w3014) -> ("AMPS"=w3009:dbl, "VOLTS"=w2998:dbl, "PF"=w2997:dbl, "Tmp Live"=w2996:dbl, "Tmp Neut"=w2999:dbl)
                        n1944 = Unbundle(w3013) -> ("CYCLE"=w2994:dbl)  [unwired: 2 out]
                        n1945 = Build Array(w2998) -> (w2995:dbl[])
                        n1946 = Build Array(w2997) -> (w2988:dbl[])
                        n1947 = Build Array(w2996) -> (w2983:dbl[])
                        n1948 = Build Array(w2999) -> (w2978:dbl[])
                        n1949 = Build Array(w3009) -> (w3008:dbl[])
                        n1950 = Build Array(w2994) -> (w2973:dbl[])
                        n1951 = TDMS Write(0:w3015, 5:"LAB03-1 TEST VALUES", 7:w3010, 9:w3008) -> (4:w3003:refnum<k34>, 6:w3002:string, 15:w2990:errorcluster)  [unwired: 2 in, 1 out]
                        n1952 = TDMS Write(0:w3003, 5:w3002, 7:w3001, 9:w2995, 11:w2990) -> (4:w2993:refnum<k34>, 6:w2992:string, 15:w2991:errorcluster)  [unwired: 1 in, 1 out]
                        n1953 = TDMS Write(0:w2993, 5:w2992, 7:w2989, 9:w2988, 11:w2991) -> (4:w2987:refnum<k34>, 6:w2986:string, 15:w2985:errorcluster)  [unwired: 1 in, 1 out]
                        n1954 = TDMS Write(0:w2987, 5:w2986, 7:w2984, 9:w2983, 11:w2985) -> (4:w2982:refnum<k34>, 6:w2981:string, 15:w2980:errorcluster)  [unwired: 1 in, 1 out]
                        n1955 = TDMS Write(0:w2982, 5:w2981, 7:w2979, 9:w2978, 11:w2980) -> (4:w2977:refnum<k34>, 6:w2976:string, 15:w2975:errorcluster)  [unwired: 1 in, 1 out]
                        n1956 = TDMS Write(0:w2977, 5:w2976, 7:w2974, 9:w2973, 11:w2975) -> (15:w2972:errorcluster)  [unwired: 1 in, 3 out]
                        n1957 = local write "data file error"(w2972) -> ()
                      }
                    }
                  }
                  frame #5 {
                    # "LAB03-2"
                    n1958 = case shown="True" w3016 {
                      frame False {
                      }
                      frame True {
                        n1959 = local read "DISP LAB03-2"() -> (w3058:T4)
                        n1960 = local read "SIG LAB03-2"() -> (w3059:T2)
                        n1961 = local read "TDMS LAB03-2"() -> (w3060:refnum<k34>)
                        n1962 = Build Array("TEMP Neut") -> (w3024:string[])
                        n1963 = Build Array("CYCLE") -> (w3019:string[])
                        n1964 = Build Array("TEMP Live") -> (w3029:string[])
                        n1965 = Build Array("PF") -> (w3034:string[])
                        n1966 = Build Array("AMPS") -> (w3055:string[])
                        n1967 = Build Array("VOLTS") -> (w3046:string[])
                        n1968 = Unbundle(w3059) -> ("AMPS"=w3054:dbl, "VOLTS"=w3043:dbl, "PF"=w3042:dbl, "Tmp Live"=w3041:dbl, "Tmp Neut"=w3044:dbl)
                        n1969 = Unbundle(w3058) -> ("CYCLE"=w3039:dbl)  [unwired: 2 out]
                        n1970 = Build Array(w3043) -> (w3040:dbl[])
                        n1971 = Build Array(w3042) -> (w3033:dbl[])
                        n1972 = Build Array(w3041) -> (w3028:dbl[])
                        n1973 = Build Array(w3044) -> (w3023:dbl[])
                        n1974 = Build Array(w3054) -> (w3053:dbl[])
                        n1975 = Build Array(w3039) -> (w3018:dbl[])
                        n1976 = TDMS Write(0:w3060, 5:"LAB03-2 TEST VALUES", 7:w3055, 9:w3053) -> (4:w3048:refnum<k34>, 6:w3047:string, 15:w3035:errorcluster)  [unwired: 2 in, 1 out]
                        n1977 = TDMS Write(0:w3048, 5:w3047, 7:w3046, 9:w3040, 11:w3035) -> (4:w3038:refnum<k34>, 6:w3037:string, 15:w3036:errorcluster)  [unwired: 1 in, 1 out]
                        n1978 = TDMS Write(0:w3038, 5:w3037, 7:w3034, 9:w3033, 11:w3036) -> (4:w3032:refnum<k34>, 6:w3031:string, 15:w3030:errorcluster)  [unwired: 1 in, 1 out]
                        n1979 = TDMS Write(0:w3032, 5:w3031, 7:w3029, 9:w3028, 11:w3030) -> (4:w3027:refnum<k34>, 6:w3026:string, 15:w3025:errorcluster)  [unwired: 1 in, 1 out]
                        n1980 = TDMS Write(0:w3027, 5:w3026, 7:w3024, 9:w3023, 11:w3025) -> (4:w3022:refnum<k34>, 6:w3021:string, 15:w3020:errorcluster)  [unwired: 1 in, 1 out]
                        n1981 = TDMS Write(0:w3022, 5:w3021, 7:w3019, 9:w3018, 11:w3020) -> (15:w3017:errorcluster)  [unwired: 1 in, 3 out]
                        n1982 = local write "data file error"(w3017) -> ()
                      }
                    }
                  }
                  frame #6 {
                    # "LAB04-1"
                    n1983 = case shown="True" w3061 {
                      frame False {
                      }
                      frame True {
                        n1984 = local read "DISP LAB04-1"() -> (w3103:T4)
                        n1985 = local read "SIG LAB04-1"() -> (w3104:T2)
                        n1986 = local read "TDMS LAB04-1"() -> (w3105:refnum<k34>)
                        n1987 = Build Array("TEMP Neut") -> (w3069:string[])
                        n1988 = Build Array("CYCLE") -> (w3064:string[])
                        n1989 = Build Array("TEMP Live") -> (w3074:string[])
                        n1990 = Build Array("PF") -> (w3079:string[])
                        n1991 = Build Array("AMPS") -> (w3100:string[])
                        n1992 = Build Array("VOLTS") -> (w3091:string[])
                        n1993 = Unbundle(w3104) -> ("AMPS"=w3099:dbl, "VOLTS"=w3088:dbl, "PF"=w3087:dbl, "Tmp Live"=w3086:dbl, "Tmp Neut"=w3089:dbl)
                        n1994 = Unbundle(w3103) -> ("CYCLE"=w3084:dbl)  [unwired: 2 out]
                        n1995 = Build Array(w3088) -> (w3085:dbl[])
                        n1996 = Build Array(w3087) -> (w3078:dbl[])
                        n1997 = Build Array(w3086) -> (w3073:dbl[])
                        n1998 = Build Array(w3089) -> (w3068:dbl[])
                        n1999 = Build Array(w3099) -> (w3098:dbl[])
                        n2000 = Build Array(w3084) -> (w3063:dbl[])
                        n2001 = TDMS Write(0:w3105, 5:"LAB04-1 TEST VALUES", 7:w3100, 9:w3098) -> (4:w3093:refnum<k34>, 6:w3092:string, 15:w3080:errorcluster)  [unwired: 2 in, 1 out]
                        n2002 = TDMS Write(0:w3093, 5:w3092, 7:w3091, 9:w3085, 11:w3080) -> (4:w3083:refnum<k34>, 6:w3082:string, 15:w3081:errorcluster)  [unwired: 1 in, 1 out]
                        n2003 = TDMS Write(0:w3083, 5:w3082, 7:w3079, 9:w3078, 11:w3081) -> (4:w3077:refnum<k34>, 6:w3076:string, 15:w3075:errorcluster)  [unwired: 1 in, 1 out]
                        n2004 = TDMS Write(0:w3077, 5:w3076, 7:w3074, 9:w3073, 11:w3075) -> (4:w3072:refnum<k34>, 6:w3071:string, 15:w3070:errorcluster)  [unwired: 1 in, 1 out]
                        n2005 = TDMS Write(0:w3072, 5:w3071, 7:w3069, 9:w3068, 11:w3070) -> (4:w3067:refnum<k34>, 6:w3066:string, 15:w3065:errorcluster)  [unwired: 1 in, 1 out]
                        n2006 = TDMS Write(0:w3067, 5:w3066, 7:w3064, 9:w3063, 11:w3065) -> (15:w3062:errorcluster)  [unwired: 1 in, 3 out]
                        n2007 = local write "data file error"(w3062) -> ()
                      }
                    }
                  }
                  frame #7 {
                    # "LAB04-2"
                    n2008 = case shown="True" w3106 {
                      frame False {
                      }
                      frame True {
                        n2009 = local read "DISP LAB04-2"() -> (w3148:T4)
                        n2010 = local read "SIG LAB04-2"() -> (w3149:T2)
                        n2011 = local read "TDMS LAB04-2"() -> (w3150:refnum<k34>)
                        n2012 = Build Array("TEMP Neut") -> (w3114:string[])
                        n2013 = Build Array("CYCLE") -> (w3109:string[])
                        n2014 = Build Array("TEMP Live") -> (w3119:string[])
                        n2015 = Build Array("PF") -> (w3124:string[])
                        n2016 = Build Array("AMPS") -> (w3145:string[])
                        n2017 = Build Array("VOLTS") -> (w3136:string[])
                        n2018 = Unbundle(w3149) -> ("AMPS"=w3144:dbl, "VOLTS"=w3133:dbl, "PF"=w3132:dbl, "Tmp Live"=w3131:dbl, "Tmp Neut"=w3134:dbl)
                        n2019 = Unbundle(w3148) -> ("CYCLE"=w3129:dbl)  [unwired: 2 out]
                        n2020 = Build Array(w3133) -> (w3130:dbl[])
                        n2021 = Build Array(w3132) -> (w3123:dbl[])
                        n2022 = Build Array(w3131) -> (w3118:dbl[])
                        n2023 = Build Array(w3134) -> (w3113:dbl[])
                        n2024 = Build Array(w3144) -> (w3143:dbl[])
                        n2025 = Build Array(w3129) -> (w3108:dbl[])
                        n2026 = TDMS Write(0:w3150, 5:"LAB04-2 TEST VALUES", 7:w3145, 9:w3143) -> (4:w3138:refnum<k34>, 6:w3137:string, 15:w3125:errorcluster)  [unwired: 2 in, 1 out]
                        n2027 = TDMS Write(0:w3138, 5:w3137, 7:w3136, 9:w3130, 11:w3125) -> (4:w3128:refnum<k34>, 6:w3127:string, 15:w3126:errorcluster)  [unwired: 1 in, 1 out]
                        n2028 = TDMS Write(0:w3128, 5:w3127, 7:w3124, 9:w3123, 11:w3126) -> (4:w3122:refnum<k34>, 6:w3121:string, 15:w3120:errorcluster)  [unwired: 1 in, 1 out]
                        n2029 = TDMS Write(0:w3122, 5:w3121, 7:w3119, 9:w3118, 11:w3120) -> (4:w3117:refnum<k34>, 6:w3116:string, 15:w3115:errorcluster)  [unwired: 1 in, 1 out]
                        n2030 = TDMS Write(0:w3117, 5:w3116, 7:w3114, 9:w3113, 11:w3115) -> (4:w3112:refnum<k34>, 6:w3111:string, 15:w3110:errorcluster)  [unwired: 1 in, 1 out]
                        n2031 = TDMS Write(0:w3112, 5:w3111, 7:w3109, 9:w3108, 11:w3110) -> (15:w3107:errorcluster)  [unwired: 1 in, 3 out]
                        n2032 = local write "data file error"(w3107) -> ()
                      }
                    }
                  }
                  frame #8 {
                    # "LAB05-1"
                    n2033 = case shown="True" w3151 {
                      frame False {
                      }
                      frame True {
                        n2034 = local read "DISP LAB05-1"() -> (w3193:T4)
                        n2035 = local read "SIG LAB05-1"() -> (w3194:T2)
                        n2036 = local read "TDMS LAB05-1"() -> (w3195:refnum<k34>)
                        n2037 = Build Array("TEMP Neut") -> (w3159:string[])
                        n2038 = Build Array("CYCLE") -> (w3154:string[])
                        n2039 = Build Array("TEMP Live") -> (w3164:string[])
                        n2040 = Build Array("PF") -> (w3169:string[])
                        n2041 = Build Array("AMPS") -> (w3190:string[])
                        n2042 = Build Array("VOLTS") -> (w3181:string[])
                        n2043 = Unbundle(w3194) -> ("AMPS"=w3189:dbl, "VOLTS"=w3178:dbl, "PF"=w3177:dbl, "Tmp Live"=w3176:dbl, "Tmp Neut"=w3179:dbl)
                        n2044 = Unbundle(w3193) -> ("CYCLE"=w3174:dbl)  [unwired: 2 out]
                        n2045 = Build Array(w3178) -> (w3175:dbl[])
                        n2046 = Build Array(w3177) -> (w3168:dbl[])
                        n2047 = Build Array(w3176) -> (w3163:dbl[])
                        n2048 = Build Array(w3179) -> (w3158:dbl[])
                        n2049 = Build Array(w3189) -> (w3188:dbl[])
                        n2050 = Build Array(w3174) -> (w3153:dbl[])
                        n2051 = TDMS Write(0:w3195, 5:"LAB05-1 TEST VALUES", 7:w3190, 9:w3188) -> (4:w3183:refnum<k34>, 6:w3182:string, 15:w3170:errorcluster)  [unwired: 2 in, 1 out]
                        n2052 = TDMS Write(0:w3183, 5:w3182, 7:w3181, 9:w3175, 11:w3170) -> (4:w3173:refnum<k34>, 6:w3172:string, 15:w3171:errorcluster)  [unwired: 1 in, 1 out]
                        n2053 = TDMS Write(0:w3173, 5:w3172, 7:w3169, 9:w3168, 11:w3171) -> (4:w3167:refnum<k34>, 6:w3166:string, 15:w3165:errorcluster)  [unwired: 1 in, 1 out]
                        n2054 = TDMS Write(0:w3167, 5:w3166, 7:w3164, 9:w3163, 11:w3165) -> (4:w3162:refnum<k34>, 6:w3161:string, 15:w3160:errorcluster)  [unwired: 1 in, 1 out]
                        n2055 = TDMS Write(0:w3162, 5:w3161, 7:w3159, 9:w3158, 11:w3160) -> (4:w3157:refnum<k34>, 6:w3156:string, 15:w3155:errorcluster)  [unwired: 1 in, 1 out]
                        n2056 = TDMS Write(0:w3157, 5:w3156, 7:w3154, 9:w3153, 11:w3155) -> (15:w3152:errorcluster)  [unwired: 1 in, 3 out]
                        n2057 = local write "data file error"(w3152) -> ()
                      }
                    }
                  }
                  frame #9 {
                    # "LAB05-2"
                    n2058 = case shown="True" w3196 {
                      frame False {
                      }
                      frame True {
                        n2059 = local read "DISP LAB05-2"() -> (w3238:T4)
                        n2060 = local read "SIG LAB05-2"() -> (w3239:T2)
                        n2061 = local read "TDMS LAB05-2"() -> (w3240:refnum<k34>)
                        n2062 = Build Array("TEMP Neut") -> (w3204:string[])
                        n2063 = Build Array("CYCLE") -> (w3199:string[])
                        n2064 = Build Array("TEMP Live") -> (w3209:string[])
                        n2065 = Build Array("PF") -> (w3214:string[])
                        n2066 = Build Array("AMPS") -> (w3235:string[])
                        n2067 = Build Array("VOLTS") -> (w3226:string[])
                        n2068 = Unbundle(w3239) -> ("AMPS"=w3234:dbl, "VOLTS"=w3223:dbl, "PF"=w3222:dbl, "Tmp Live"=w3221:dbl, "Tmp Neut"=w3224:dbl)
                        n2069 = Unbundle(w3238) -> ("CYCLE"=w3219:dbl)  [unwired: 2 out]
                        n2070 = Build Array(w3223) -> (w3220:dbl[])
                        n2071 = Build Array(w3222) -> (w3213:dbl[])
                        n2072 = Build Array(w3221) -> (w3208:dbl[])
                        n2073 = Build Array(w3224) -> (w3203:dbl[])
                        n2074 = Build Array(w3234) -> (w3233:dbl[])
                        n2075 = Build Array(w3219) -> (w3198:dbl[])
                        n2076 = TDMS Write(0:w3240, 5:"LAB05-2 TEST VALUES", 7:w3235, 9:w3233) -> (4:w3228:refnum<k34>, 6:w3227:string, 15:w3215:errorcluster)  [unwired: 2 in, 1 out]
                        n2077 = TDMS Write(0:w3228, 5:w3227, 7:w3226, 9:w3220, 11:w3215) -> (4:w3218:refnum<k34>, 6:w3217:string, 15:w3216:errorcluster)  [unwired: 1 in, 1 out]
                        n2078 = TDMS Write(0:w3218, 5:w3217, 7:w3214, 9:w3213, 11:w3216) -> (4:w3212:refnum<k34>, 6:w3211:string, 15:w3210:errorcluster)  [unwired: 1 in, 1 out]
                        n2079 = TDMS Write(0:w3212, 5:w3211, 7:w3209, 9:w3208, 11:w3210) -> (4:w3207:refnum<k34>, 6:w3206:string, 15:w3205:errorcluster)  [unwired: 1 in, 1 out]
                        n2080 = TDMS Write(0:w3207, 5:w3206, 7:w3204, 9:w3203, 11:w3205) -> (4:w3202:refnum<k34>, 6:w3201:string, 15:w3200:errorcluster)  [unwired: 1 in, 1 out]
                        n2081 = TDMS Write(0:w3202, 5:w3201, 7:w3199, 9:w3198, 11:w3200) -> (15:w3197:errorcluster)  [unwired: 1 in, 3 out]
                        n2082 = local write "data file error"(w3197) -> ()
                      }
                    }
                  }
                }
              }
            }
          }
          frame #13 {
            # "check for amps fail"
            # "check for cycle test & temperature rise fail conditions"
            n2083 = local read "on loops"() -> (w3266:dbl)
            n2084 = local read "jig cycle"() -> (w3263:dbl)
            n2085 = local read "jig cycle"() -> (w3268:dbl)
            n2086 = Add(x=w3266, y=3.0) -> (x+y=w3264:dbl)
            n2087 = Equal?(x=w3263, y=w3264) -> (x = y?=w3259:bool)
            n2088 = Equal?(x=w3268, y=1.0) -> (x = y?=w3261:bool)
            n2089 = stacked-sequence {
              tunnel: w3262 -> [w3271 _ _ _ _ _ _ _ _ _]
              tunnel: w3261 -> [w3272 w3292 w3312 w3332 w3352 w3372 w3392 w3412 w3432 w3452]
              tunnel: w3260 -> [w3269 _ _ _ _ _ _ _ _ _]
              tunnel: w3259 -> [w3270 w3291 w3311 w3331 w3351 w3371 w3391 w3411 w3431 w3451]
              tunnel: w3258 -> [_ w3290 _ _ _ _ _ _ _ _]
              tunnel: w3257 -> [_ w3289 _ _ _ _ _ _ _ _]
              tunnel: w3256 -> [_ _ w3310 _ _ _ _ _ _ _]
              tunnel: w3255 -> [_ _ w3309 _ _ _ _ _ _ _]
              tunnel: w3254 -> [_ _ _ w3330 _ _ _ _ _ _]
              tunnel: w3253 -> [_ _ _ w3329 _ _ _ _ _ _]
              tunnel: w3252 -> [_ _ _ _ w3350 _ _ _ _ _]
              tunnel: w3251 -> [_ _ _ _ w3349 _ _ _ _ _]
              tunnel: w3250 -> [_ _ _ _ _ w3370 _ _ _ _]
              tunnel: w3249 -> [_ _ _ _ _ w3369 _ _ _ _]
              tunnel: w3248 -> [_ _ _ _ _ _ w3390 _ _ _]
              tunnel: w3247 -> [_ _ _ _ _ _ w3389 _ _ _]
              tunnel: w3246 -> [_ _ _ _ _ _ _ w3410 _ _]
              tunnel: w3245 -> [_ _ _ _ _ _ _ w3409 _ _]
              tunnel: w3244 -> [_ _ _ _ _ _ _ _ w3430 _]
              tunnel: w3243 -> [_ _ _ _ _ _ _ _ w3429 _]
              tunnel: w3242 -> [_ _ _ _ _ _ _ _ _ w3450]
              tunnel: w3241 -> [_ _ _ _ _ _ _ _ _ w3449]
              frame #0 {
                # "LAB01-1"
                n2090 = case shown="True" w3269 {
                  tunnel: w3272 -> [_ w3285]
                  tunnel: w3271 -> [_ w3282]
                  tunnel: w3270 -> [_ w3281]
                  frame False {
                  }
                  frame True {
                    n2091 = local read "TEMP START LAB01-1"() -> (w3287:cluster{"TL":dbl, "TN":dbl})
                    n2092 = local read "RESULT LAB01-1"() -> (w3275:bool)
                    n2093 = local read "FAIL LAB01-1"() -> (w3278:cluster{"LO":dbl, "HI":dbl})
                    n2094 = local read "TDMS LAB01-1"() -> (w3286:refnum<k34>)
                    n2095 = local read "SET LAB01-1"() -> (w3283:T5)
                    n2096 = local read "DISP LAB01-1"() -> (w3284:T4)
                    n2097 = local read "SIG LAB01-1"() -> (w3288:T2)
                    n2098 = Bundle("FAIL LAB01-1"=w3278, "SIG LAB01-1"=w3288, "TEMP START LAB01-1"=w3287, "DISP LAB01-1"=w3284, "SET LAB01-1"=w3283, "TDMS LAB01-1"=w3286) -> (w3273:T25)  [unwired: 1 in]
                    n2099 = call "sub vi - cycle&temp fail v6.vi"("Amps Lo?"=w3285, "Input Cluster"=w3273, "SELECT"=w3282, "Amps Hi?"=w3281, "Result In"=w3275) -> ("(FAIL) out"=w3277:cluster{"FAIL LO":dbl, "FAIL HI":dbl}, "(DISP) out"=w3280:T4, "T-RISE"=w3274:cluster{"T-RISE (L)":dbl, "T-RISE (N)":dbl}, "Result Out"=w3276:bool, "file error"=w3279:errorcluster)  [unwired: 10 in]
                    n2100 = local write "TEMP RISE LAB01-1"(w3274) -> ()
                    n2101 = local write "FAIL LAB01-1"(w3277) -> ()
                    n2102 = local write "DISP LAB01-1"(w3280) -> ()
                    n2103 = local write "RESULT LAB01-1"(w3276) -> ()
                    n2104 = local write "data file error"(w3279) -> ()
                  }
                }
              }
              frame #1 {
                # "LAB01-2"
                n2105 = case shown="True" w3290 {
                  tunnel: w3292 -> [_ w3305]
                  tunnel: w3289 -> [_ w3302]
                  tunnel: w3291 -> [_ w3301]
                  frame False {
                  }
                  frame True {
                    n2106 = local read "TEMP START LAB01-2"() -> (w3307:cluster{"TL":dbl, "TN":dbl})
                    n2107 = local read "FAIL LAB01-2"() -> (w3298:cluster{"LO":dbl, "HI":dbl})
                    n2108 = local read "TDMS LAB01-2"() -> (w3306:refnum<k34>)
                    n2109 = local read "SET LAB01-2"() -> (w3303:T5)
                    n2110 = local read "DISP LAB01-2"() -> (w3304:T4)
                    n2111 = local read "RESULT LAB01-2"() -> (w3295:bool)
                    n2112 = local read "SIG LAB01-2"() -> (w3308:T2)
                    n2113 = Bundle("FAIL LAB01-2"=w3298, "SIG LAB01-2"=w3308, "TEMP START LAB01-2"=w3307, "DISP LAB01-2"=w3304, "SET LAB01-2"=w3303, "TDMS LAB01-2"=w3306) -> (w3293:T26)  [unwired: 1 in]
                    n2114 = call "sub vi - cycle&temp fail v6.vi"("Amps Lo?"=w3305, "Input Cluster"=w3293, "SELECT"=w3302, "Amps Hi?"=w3301, "Result In"=w3295) -> ("(FAIL) out"=w3297:cluster{"FAIL LO":dbl, "FAIL HI":dbl}, "(DISP) out"=w3300:T4, "T-RISE"=w3294:cluster{"T-RISE (L)":dbl, "T-RISE (N)":dbl}, "Result Out"=w3296:bool, "file error"=w3299:errorcluster)  [unwired: 10 in]
                    n2115 = local write "TEMP RISE LAB01-2"(w3294) -> ()
                    n2116 = local write "FAIL LAB01-2"(w3297) -> ()
                    n2117 = local write "DISP LAB01-2"(w3300) -> ()
                    n2118 = local write "RESULT LAB01-2"(w3296) -> ()
                    n2119 = local write "data file error"(w3299) -> ()
                  }
                }
              }
              frame #2 {
                # "LAB02-1"
                n2120 = case shown="True" w3310 {
                  tunnel: w3312 -> [_ w3325]
                  tunnel: w3309 -> [_ w3322]
                  tunnel: w3311 -> [_ w3321]
                  frame False {
                  }
                  frame True {
                    n2121 = local read "TEMP START LAB02-1"() -> (w3327:cluster{"TL":dbl, "TN":dbl})
                    n2122 = local read "FAIL LAB02-1"() -> (w3318:cluster{"LO":dbl, "HI":dbl})
                    n2123 = local read "TDMS LAB02-1"() -> (w3326:refnum<k34>)
                    n2124 = local read "SET LAB02-1"() -> (w3323:T5)
                    n2125 = local read "DISP LAB02-1"() -> (w3324:T4)
                    n2126 = local read "SIG LAB02-1"() -> (w3328:T2)
                    n2127 = local read "RESULT LAB02-1"() -> (w3315:bool)
                    n2128 = Bundle("FAIL LAB02-1"=w3318, "SIG LAB02-1"=w3328, "TEMP START LAB02-1"=w3327, "DISP LAB02-1"=w3324, "SET LAB02-1"=w3323, "TDMS LAB02-1"=w3326) -> (w3313:T27)  [unwired: 1 in]
                    n2129 = call "sub vi - cycle&temp fail v6.vi"("Amps Lo?"=w3325, "Input Cluster"=w3313, "SELECT"=w3322, "Amps Hi?"=w3321, "Result In"=w3315) -> ("(FAIL) out"=w3317:cluster{"FAIL LO":dbl, "FAIL HI":dbl}, "(DISP) out"=w3320:T4, "T-RISE"=w3314:cluster{"T-RISE (L)":dbl, "T-RISE (N)":dbl}, "Result Out"=w3316:bool, "file error"=w3319:errorcluster)  [unwired: 10 in]
                    n2130 = local write "TEMP RISE LAB02-1"(w3314) -> ()
                    n2131 = local write "FAIL LAB02-1"(w3317) -> ()
                    n2132 = local write "DISP LAB02-1"(w3320) -> ()
                    n2133 = local write "RESULT LAB02-1"(w3316) -> ()
                    n2134 = local write "data file error"(w3319) -> ()
                  }
                }
              }
              frame #3 {
                # "LAB02-2"
                n2135 = case shown="True" w3330 {
                  tunnel: w3332 -> [_ w3345]
                  tunnel: w3329 -> [_ w3342]
                  tunnel: w3331 -> [_ w3341]
                  frame False {
                  }
                  frame True {
                    n2136 = local read "TEMP START LAB02-2"() -> (w3347:cluster{"TL":dbl, "TN":dbl})
                    n2137 = local read "FAIL LAB02-2"() -> (w3338:cluster{"LO":dbl, "HI":dbl})
                    n2138 = local read "TDMS LAB02-2"() -> (w3346:refnum<k34>)
                    n2139 = local read "SET LAB02-2"() -> (w3343:T5)
                    n2140 = local read "DISP LAB02-2"() -> (w3344:T4)
                    n2141 = local read "SIG LAB02-2"() -> (w3348:T2)
                    n2142 = local read "RESULT LAB02-2"() -> (w3335:bool)
                    n2143 = Bundle("FAIL LAB02-2"=w3338, "SIG LAB02-2"=w3348, "TEMP START LAB02-2"=w3347, "DISP LAB02-2"=w3344, "SET LAB02-2"=w3343, "TDMS LAB02-2"=w3346) -> (w3333:T28)  [unwired: 1 in]
                    n2144 = call "sub vi - cycle&temp fail v6.vi"("Amps Lo?"=w3345, "Input Cluster"=w3333, "SELECT"=w3342, "Amps Hi?"=w3341, "Result In"=w3335) -> ("(FAIL) out"=w3337:cluster{"FAIL LO":dbl, "FAIL HI":dbl}, "(DISP) out"=w3340:T4, "T-RISE"=w3334:cluster{"T-RISE (L)":dbl, "T-RISE (N)":dbl}, "Result Out"=w3336:bool, "file error"=w3339:errorcluster)  [unwired: 10 in]
                    n2145 = local write "TEMP RISE LAB02-2"(w3334) -> ()
                    n2146 = local write "FAIL LAB02-2"(w3337) -> ()
                    n2147 = local write "DISP LAB02-2"(w3340) -> ()
                    n2148 = local write "RESULT LAB02-2"(w3336) -> ()
                    n2149 = local write "data file error"(w3339) -> ()
                  }
                }
              }
              frame #4 {
                # "LAB03-1"
                n2150 = case shown="True" w3350 {
                  tunnel: w3352 -> [_ w3365]
                  tunnel: w3349 -> [_ w3362]
                  tunnel: w3351 -> [_ w3361]
                  frame False {
                  }
                  frame True {
                    n2151 = local read "TEMP START LAB03-1"() -> (w3367:cluster{"TL":dbl, "TN":dbl})
                    n2152 = local read "FAIL LAB03-1"() -> (w3358:cluster{"LO":dbl, "HI":dbl})
                    n2153 = local read "TDMS LAB03-1"() -> (w3366:refnum<k34>)
                    n2154 = local read "SET LAB03-1"() -> (w3363:T5)
                    n2155 = local read "DISP LAB03-1"() -> (w3364:T4)
                    n2156 = local read "SIG LAB03-1"() -> (w3368:T2)
                    n2157 = local read "RESULT LAB03-1"() -> (w3355:bool)
                    n2158 = Bundle("FAIL LAB03-1"=w3358, "SIG LAB03-1"=w3368, "TEMP START LAB03-1"=w3367, "DISP LAB03-1"=w3364, "SET LAB03-1"=w3363, "TDMS LAB03-1"=w3366) -> (w3353:T29)  [unwired: 1 in]
                    n2159 = call "sub vi - cycle&temp fail v6.vi"("Amps Lo?"=w3365, "Input Cluster"=w3353, "SELECT"=w3362, "Amps Hi?"=w3361, "Result In"=w3355) -> ("(FAIL) out"=w3357:cluster{"FAIL LO":dbl, "FAIL HI":dbl}, "(DISP) out"=w3360:T4, "T-RISE"=w3354:cluster{"T-RISE (L)":dbl, "T-RISE (N)":dbl}, "Result Out"=w3356:bool, "file error"=w3359:errorcluster)  [unwired: 10 in]
                    n2160 = local write "TEMP RISE LAB03-1"(w3354) -> ()
                    n2161 = local write "FAIL LAB03-1"(w3357) -> ()
                    n2162 = local write "DISP LAB03-1"(w3360) -> ()
                    n2163 = local write "RESULT LAB03-1"(w3356) -> ()
                    n2164 = local write "data file error"(w3359) -> ()
                  }
                }
              }
              frame #5 {
                # "LAB03-2"
                n2165 = case shown="True" w3370 {
                  tunnel: w3372 -> [_ w3385]
                  tunnel: w3369 -> [_ w3382]
                  tunnel: w3371 -> [_ w3381]
                  frame False {
                  }
                  frame True {
                    n2166 = local read "TEMP START LAB03-2"() -> (w3387:cluster{"TL":dbl, "TN":dbl})
                    n2167 = local read "FAIL LAB03-2"() -> (w3378:cluster{"LO":dbl, "HI":dbl})
                    n2168 = local read "TDMS LAB03-2"() -> (w3386:refnum<k34>)
                    n2169 = local read "SET LAB03-2"() -> (w3383:T5)
                    n2170 = local read "DISP LAB03-2"() -> (w3384:T4)
                    n2171 = local read "RESULT LAB03-2"() -> (w3375:bool)
                    n2172 = local read "SIG LAB03-2"() -> (w3388:T2)
                    n2173 = Bundle("FAIL LAB03-2"=w3378, "SIG LAB03-2"=w3388, "TEMP START LAB03-2"=w3387, "DISP LAB03-2"=w3384, "SET LAB03-2"=w3383, "TDMS LAB03-2"=w3386) -> (w3373:T30)  [unwired: 1 in]
                    n2174 = call "sub vi - cycle&temp fail v6.vi"("Amps Lo?"=w3385, "Input Cluster"=w3373, "SELECT"=w3382, "Amps Hi?"=w3381, "Result In"=w3375) -> ("(FAIL) out"=w3377:cluster{"FAIL LO":dbl, "FAIL HI":dbl}, "(DISP) out"=w3380:T4, "T-RISE"=w3374:cluster{"T-RISE (L)":dbl, "T-RISE (N)":dbl}, "Result Out"=w3376:bool, "file error"=w3379:errorcluster)  [unwired: 10 in]
                    n2175 = local write "FAIL LAB03-2"(w3377) -> ()
                    n2176 = local write "TEMP RISE LAB03-2"(w3374) -> ()
                    n2177 = local write "DISP LAB03-2"(w3380) -> ()
                    n2178 = local write "RESULT LAB03-2"(w3376) -> ()
                    n2179 = local write "data file error"(w3379) -> ()
                  }
                }
              }
              frame #6 {
                # "LAB04-1"
                n2180 = case shown="True" w3390 {
                  tunnel: w3392 -> [_ w3405]
                  tunnel: w3389 -> [_ w3402]
                  tunnel: w3391 -> [_ w3401]
                  frame False {
                  }
                  frame True {
                    n2181 = local read "TEMP START LAB04-1"() -> (w3407:cluster{"TL":dbl, "TN":dbl})
                    n2182 = local read "FAIL LAB04-1"() -> (w3398:cluster{"LO":dbl, "HI":dbl})
                    n2183 = local read "TDMS LAB04-1"() -> (w3406:refnum<k34>)
                    n2184 = local read "SET LAB04-1"() -> (w3403:T5)
                    n2185 = local read "DISP LAB04-1"() -> (w3404:T4)
                    n2186 = local read "SIG LAB04-1"() -> (w3408:T2)
                    n2187 = local read "RESULT LAB04-1"() -> (w3395:bool)
                    n2188 = Bundle("FAIL LAB04-1"=w3398, "SIG LAB04-1"=w3408, "TEMP START LAB04-1"=w3407, "DISP LAB04-1"=w3404, "SET LAB04-1"=w3403, "TDMS LAB04-1"=w3406) -> (w3393:T31)  [unwired: 1 in]
                    n2189 = call "sub vi - cycle&temp fail v6.vi"("Amps Lo?"=w3405, "Input Cluster"=w3393, "SELECT"=w3402, "Amps Hi?"=w3401, "Result In"=w3395) -> ("(FAIL) out"=w3397:cluster{"FAIL LO":dbl, "FAIL HI":dbl}, "(DISP) out"=w3400:T4, "T-RISE"=w3394:cluster{"T-RISE (L)":dbl, "T-RISE (N)":dbl}, "Result Out"=w3396:bool, "file error"=w3399:errorcluster)  [unwired: 10 in]
                    n2190 = local write "TEMP RISE LAB04-1"(w3394) -> ()
                    n2191 = local write "FAIL LAB04-1"(w3397) -> ()
                    n2192 = local write "DISP LAB04-1"(w3400) -> ()
                    n2193 = local write "RESULT LAB04-1"(w3396) -> ()
                    n2194 = local write "data file error"(w3399) -> ()
                  }
                }
              }
              frame #7 {
                # "LAB04-2"
                n2195 = case shown="True" w3410 {
                  tunnel: w3412 -> [_ w3425]
                  tunnel: w3409 -> [_ w3422]
                  tunnel: w3411 -> [_ w3421]
                  frame False {
                  }
                  frame True {
                    n2196 = local read "TEMP START LAB04-2"() -> (w3427:cluster{"TL":dbl, "TN":dbl})
                    n2197 = local read "FAIL LAB04-2"() -> (w3418:cluster{"LO":dbl, "HI":dbl})
                    n2198 = local read "TDMS LAB04-2"() -> (w3426:refnum<k34>)
                    n2199 = local read "SET LAB04-2"() -> (w3423:T5)
                    n2200 = local read "DISP LAB04-2"() -> (w3424:T4)
                    n2201 = local read "SIG LAB04-2"() -> (w3428:T2)
                    n2202 = local read "RESULT LAB04-2"() -> (w3415:bool)
                    n2203 = Bundle("FAIL LAB04-2"=w3418, "SIG LAB04-2"=w3428, "TEMP START LAB04-2"=w3427, "DISP LAB04-2"=w3424, "SET LAB04-2"=w3423, "TDMS LAB04-2"=w3426) -> (w3413:T32)  [unwired: 1 in]
                    n2204 = call "sub vi - cycle&temp fail v6.vi"("Amps Lo?"=w3425, "Input Cluster"=w3413, "SELECT"=w3422, "Amps Hi?"=w3421, "Result In"=w3415) -> ("(FAIL) out"=w3417:cluster{"FAIL LO":dbl, "FAIL HI":dbl}, "(DISP) out"=w3420:T4, "T-RISE"=w3414:cluster{"T-RISE (L)":dbl, "T-RISE (N)":dbl}, "Result Out"=w3416:bool, "file error"=w3419:errorcluster)  [unwired: 10 in]
                    n2205 = local write "TEMP RISE LAB04-2"(w3414) -> ()
                    n2206 = local write "FAIL LAB04-2"(w3417) -> ()
                    n2207 = local write "DISP LAB04-2"(w3420) -> ()
                    n2208 = local write "RESULT LAB04-2"(w3416) -> ()
                    n2209 = local write "data file error"(w3419) -> ()
                  }
                }
              }
              frame #8 {
                # "LAB05-1"
                n2210 = case shown="True" w3430 {
                  tunnel: w3432 -> [_ w3445]
                  tunnel: w3429 -> [_ w3442]
                  tunnel: w3431 -> [_ w3441]
                  frame False {
                  }
                  frame True {
                    n2211 = local read "TEMP START LAB05-1"() -> (w3447:cluster{"TL":dbl, "TN":dbl})
                    n2212 = local read "FAIL LAB05-1"() -> (w3438:cluster{"LO":dbl, "HI":dbl})
                    n2213 = local read "TDMS LAB05-1"() -> (w3446:refnum<k34>)
                    n2214 = local read "SET LAB05-1"() -> (w3443:T5)
                    n2215 = local read "DISP LAB05-1"() -> (w3444:T4)
                    n2216 = local read "SIG LAB05-1"() -> (w3448:T2)
                    n2217 = local read "RESULT LAB05-1"() -> (w3435:bool)
                    n2218 = Bundle("FAIL LAB05-1"=w3438, "SIG LAB05-1"=w3448, "TEMP START LAB05-1"=w3447, "DISP LAB05-1"=w3444, "SET LAB05-1"=w3443, "TDMS LAB05-1"=w3446) -> (w3433:T33)  [unwired: 1 in]
                    n2219 = call "sub vi - cycle&temp fail v6.vi"("Amps Lo?"=w3445, "Input Cluster"=w3433, "SELECT"=w3442, "Amps Hi?"=w3441, "Result In"=w3435) -> ("(FAIL) out"=w3437:cluster{"FAIL LO":dbl, "FAIL HI":dbl}, "(DISP) out"=w3440:T4, "T-RISE"=w3434:cluster{"T-RISE (L)":dbl, "T-RISE (N)":dbl}, "Result Out"=w3436:bool, "file error"=w3439:errorcluster)  [unwired: 10 in]
                    n2220 = local write "TEMP RISE LAB05-1"(w3434) -> ()
                    n2221 = local write "FAIL LAB05-1"(w3437) -> ()
                    n2222 = local write "DISP LAB05-1"(w3440) -> ()
                    n2223 = local write "RESULT LAB05-1"(w3436) -> ()
                    n2224 = local write "data file error"(w3439) -> ()
                  }
                }
              }
              frame #9 {
                # "LAB05-2"
                n2225 = case shown="True" w3450 {
                  tunnel: w3452 -> [_ w3465]
                  tunnel: w3449 -> [_ w3462]
                  tunnel: w3451 -> [_ w3461]
                  frame False {
                  }
                  frame True {
                    n2226 = local read "TEMP START LAB05-2"() -> (w3467:cluster{"TL":dbl, "TN":dbl})
                    n2227 = local read "FAIL LAB05-2"() -> (w3458:cluster{"LO":dbl, "HI":dbl})
                    n2228 = local read "TDMS LAB05-2"() -> (w3466:refnum<k34>)
                    n2229 = local read "SET LAB05-2"() -> (w3463:T5)
                    n2230 = local read "DISP LAB05-2"() -> (w3464:T4)
                    n2231 = local read "SIG LAB05-2"() -> (w3468:T2)
                    n2232 = local read "RESULT LAB05-2"() -> (w3455:bool)
                    n2233 = Bundle("FAIL LAB05-2"=w3458, "SIG LAB05-2"=w3468, "TEMP START LAB05-2"=w3467, "DISP LAB05-2"=w3464, "SET LAB05-2"=w3463, "TDMS LAB05-2"=w3466) -> (w3453:T34)  [unwired: 1 in]
                    n2234 = call "sub vi - cycle&temp fail v6.vi"("Amps Lo?"=w3465, "Input Cluster"=w3453, "SELECT"=w3462, "Amps Hi?"=w3461, "Result In"=w3455) -> ("(FAIL) out"=w3457:cluster{"FAIL LO":dbl, "FAIL HI":dbl}, "(DISP) out"=w3460:T4, "T-RISE"=w3454:cluster{"T-RISE (L)":dbl, "T-RISE (N)":dbl}, "Result Out"=w3456:bool, "file error"=w3459:errorcluster)  [unwired: 10 in]
                    n2235 = local write "TEMP RISE LAB05-2"(w3454) -> ()
                    n2236 = local write "FAIL LAB05-2"(w3457) -> ()
                    n2237 = local write "DISP LAB05-2"(w3460) -> ()
                    n2238 = local write "RESULT LAB05-2"(w3456) -> ()
                    n2239 = local write "data file error"(w3459) -> ()
                  }
                }
              }
            }
          }
          frame #14 {
            # "run calibration routine"
            n2240 = local read "CALIBRATE"() -> (w3469:bool)
            n2241 = case shown="True" w3469 {
              frame False {
              }
              frame True {
                n2242 = stacked-sequence {
                  seq-local: [w3470 _ _] -> [_ w3472 _]
                  frame #0 {
                    n2243 = call "CALIBRATION PASSWORD"() -> ("PASSWORD"=w3470:string)  [unwired: 17 in, 2 out]
                  }
                  frame #1 {
                    n2244 = Equal?(x=w3472, y="7777") -> (x = y?=w3471:bool)
                    n2245 = case shown="True" w3471 {
                      frame False {
                      }
                      frame True {
                        n2246 = stacked-sequence {
                          frame #0 {
                            n2247 = call "sub vi - calibration v1.vi"() -> ()  [unwired: 12 in]
                          }
                          frame #1 {
                            n2248 = call "sub vi - get calibration values v1.vi"() -> ("LAB01 (CAL)"=w3478:T7, "LAB02 (CAL)"=w3477:T8, "LAB03 (CAL)"=w3476:T7, "LAB04 (CAL)"=w3475:T7, "calibration file error out"=w3479:errorcluster, "LAB05 (CAL)"=w3474:T7)  [unwired: 10 in]
                            n2249 = local write "calibration file error out"(w3479) -> ()
                            n2250 = local write "CAL LAB04"(w3475) -> ()
                            n2251 = local write "CAL LAB05"(w3474) -> ()
                            n2252 = local write "CAL LAB01"(w3478) -> ()
                            n2253 = local write "CAL LAB02"(w3477) -> ()
                            n2254 = local write "CAL LAB03"(w3476) -> ()
                          }
                        }
                      }
                    }
                  }
                  frame #2 {
                    n2255 = local write "CALIBRATE"(FALSE) -> ()
                  }
                }
              }
            }
          }
          frame #15 {
            # "save certain settings to file"
            n2256 = String To Path(string="c:\\crabtree\\Set Up\\") -> (path=w3482:path)
            n2257 = Build Path(base path=w3482, name or relative path="settings.bin") -> (appended path=w3484:path)
            n2258 = Build Path(base path=w3482, name or relative path="mail.bin") -> (appended path=w3481:path)
            n2259 = Create Folder(path (use dialog)=w3482) -> (error out=w3487:errorcluster)  [unwired: 2 in, 2 out]
            n2260 = call <vilib>:"Clear Errors.vi"("error in (no error)"=w3487) -> ()  [unwired: 6 in, 1 out]
            n2261 = stacked-sequence {
              seq-local: [w3489 _] -> [_ w3502]
              tunnel: w3484 -> [_ w3503]
              tunnel: w3481 -> [_ w3501]
              frame #0 {
                n2262 = local read "C drive data root dir"() -> (w3488:path)
                n2263 = local read "Network Directory"() -> (w3494:path)
                n2264 = local read "SET LAB05-2"() -> (w3493:T5)
                n2265 = local read "SET LAB05-1"() -> (w3492:T5)
                n2266 = local read "SET LAB04-2"() -> (w3491:T5)
                n2267 = local read "SET LAB03-2"() -> (w3495:T5)
                n2268 = local read "SET LAB04-1"() -> (w3490:T5)
                n2269 = local read "SET LAB03-1"() -> (w3496:T5)
                n2270 = local read "SET LAB02-2"() -> (w3497:T5)
                n2271 = local read "SET LAB02-1"() -> (w3498:T5)
                n2272 = local read "SET LAB01-2"() -> (w3499:T5)
                n2273 = local read "SET LAB01-1"() -> (w3500:T5)
                n2274 = Bundle("SET LAB01-1"=w3500, "SET LAB01-2"=w3499, "SET LAB02-1"=w3498, "SET LAB02-2"=w3497, "SET LAB03-1"=w3496, "SET LAB03-2"=w3495, "SET LAB04-1"=w3490, "SET LAB04-2"=w3491, "SET LAB05-1"=w3492, "SET LAB05-2"=w3493, "Network Directory"=w3494, "C drive data root dir"=w3488) -> (w3489:T17)  [unwired: 1 in]
              }
              frame #1 {
                n2275 = event shown="[1] \"SET LAB01-1\", \"SET LAB01-2\", \"SET LAB02-1\", \"SET LAB02-2\", \"SET LAB03-1\", \"SET LAB03-2\", \"SET LAB04-1\", \"SET LAB04-2\", \"SET LAB05-1\", \"SET LAB05-2\", \"Network Directory\", \"C drive data root dir\": Value Change" {
                  selector: _ -> [_ _ _]
                  dyn-events: _ -> [_ _ _]
                  timeout: 10.0 -> [_ _ _]
                  tunnel: w3503 -> [_ w3505 _]
                  tunnel: w3502 -> [_ w3506 _]
                  tunnel: w3501 -> [_ _ w3517]
                  event Timeout {
                    n2276 = event-data() -> ()  [unwired: 1 in, 3 out]
                  }
                  event "SET LAB01-1", "SET LAB01-2", "SET LAB02-1", "SET LAB02-2", "SET LAB03-1", "SET LAB03-2", "SET LAB04-1", "SET LAB04-2", "SET LAB05-1", "SET LAB05-2", "Network Directory", "C drive data root dir": Value Change {
                    n2277 = event-data() -> ()  [unwired: 1 in, 6 out]
                    n2278 = Open/Create/Replace File(file path (use dialog)=w3505, operation (0:open)=T16."replace or create") -> (refnum out=w3511:refnum<file>, error out=w3510:errorcluster)  [unwired: 4 in, 1 out]
                    n2279 = Write to Binary File(file (use dialog)=w3511, data=w3506, error in=w3510) -> (refnum out=w3509:refnum<file>, error out=w3508:errorcluster)  [unwired: 3 in, 1 out]
                    n2280 = Close File(refnum=w3509, error in=w3508) -> (error out=w3507:errorcluster)  [unwired: 1 out]
                    n2281 = local write "data file error"(w3507) -> ()
                  }
                  event "MAIL SETTINGS.OUT SERVER ADDRESS", "MAIL SETTINGS.FROM ACCOUNT", "MAIL SETTINGS.USER NAME", "MAIL SETTINGS.PASSWORD", "Auto Mail Send", "TO (string):": Value Change {
                    n2282 = event-data() -> ()  [unwired: 1 in, 6 out]
                    n2283 = local read "MAIL SETTINGS"() -> (w3516:T6)
                    n2284 = local read "Auto Mail Send"() -> (w3514:bool)
                    n2285 = local read "TO (string):"() -> (w3513:string)
                    n2286 = Open/Create/Replace File(file path (use dialog)=w3517, operation (0:open)=T16."replace or create") -> (refnum out=w3522:refnum<file>, error out=w3521:errorcluster)  [unwired: 4 in, 1 out]
                    n2287 = Bundle("MAIL SETTINGS"=w3516, "Auto Mail Send"=w3514, "TO (string):"=w3513) -> (w3515:T35)  [unwired: 1 in]
                    n2288 = Write to Binary File(file (use dialog)=w3522, data=w3515, error in=w3521) -> (refnum out=w3520:refnum<file>, error out=w3519:errorcluster)  [unwired: 3 in, 1 out]
                    n2289 = Close File(refnum=w3520, error in=w3519) -> (error out=w3518:errorcluster)  [unwired: 1 out]
                    n2290 = local write "data file error"(w3518) -> ()
                  }
                }
              }
            }
          }
          frame #16 {
            # "mail control"
            n2291 = local read "MAIL SETTINGS"() -> (w3539:T6)
            n2292 = local read "Auto Mail Send"() -> (w3525:bool)
            n2293 = Unbundle(w3539) -> ("OUT SERVER ADDRESS"=w3538:string, "FROM ACCOUNT"=w3537:string, "TEST MAIL"=w3536:bool)  [unwired: 4 out]
            n2294 = stacked-sequence {
              tunnel: "TO (string):" -> [_ w3578]
              tunnel: w3539 -> [w3544 w3577]
              tunnel: w3538 -> [w3543 w3576]
              tunnel: w3537 -> [w3542 w3575]
              tunnel: w3536 -> [w3541 _]
              tunnel: w3525 -> [_ w3574]
              tunnel: w3535 -> [_ w3573]
              tunnel: w3534 -> [_ w3572]
              tunnel: w3533 -> [_ w3571]
              tunnel: w3532 -> [_ w3570]
              tunnel: w3531 -> [_ w3569]
              tunnel: w3530 -> [_ w3568]
              tunnel: w3529 -> [_ w3567]
              tunnel: w3528 -> [_ w3566]
              tunnel: w3527 -> [_ w3565]
              tunnel: w3526 -> [_ w3564]
              tunnel: "TO (string):" -> [w3540 _]
              frame #0 {
                # "mail test"
                n2295 = case shown="True" w3541 {
                  tunnel: w3544 -> [_ w3548]
                  tunnel: w3540 -> [_ w3547]
                  tunnel: w3543 -> [_ w3546]
                  tunnel: w3542 -> [_ w3545]
                  frame False {
                  }
                  frame True {
                    n2296 = stacked-sequence {
                      seq-local: [_ _ w3558 _] -> [_ _ _ w3559]
                      tunnel: w3548 -> [w3551 _ _ w3563]
                      tunnel: w3547 -> [_ _ w3556 _]
                      tunnel: w3546 -> [_ _ w3554 _]
                      tunnel: w3545 -> [_ _ w3555 _]
                      frame #0 {
                        n2297 = Bundle(cluster=w3551, "TEST MAIL STATUS"="TEST START") -> (w3549:T6)  [unwired: 6 in]
                        n2298 = local write "MAIL SETTINGS"(w3549) -> ()
                      }
                      frame #1 {
                        n2299 = Wait (ms)(milliseconds to wait=500) -> ()  [unwired: 1 out]
                      }
                      frame #2 {
                        n2300 = call "sub vi - send mail with attach v5.vi"("TO:"=w3556, "subject"="MAIL TEST FROM LAB PANEL", "from"=w3555, "out going server"=w3554, "message"="TEST MESSAGE") -> ("error out"=w3558:errorcluster)  [unwired: 10 in]
                      }
                      frame #3 {
                        n2301 = Bundle(cluster=w3563, "TEST MAIL"=FALSE, "TEST MAIL STATUS"="TEST END", "mail error"=w3559) -> (w3561:T6)  [unwired: 4 in]
                        n2302 = local write "MAIL SETTINGS"(w3561) -> ()
                      }
                    }
                  }
                }
              }
              frame #1 {
                # "mail report"
                n2303 = stacked-sequence {
                  seq-local: [_ w3643 _ _] -> [_ _ _ w3811]
                  seq-local: [_ _ w3724 _] -> [_ _ _ w3801]
                  seq-local: [w3588 _ _ _] -> [_ w3637 _ _]
                  seq-local: [w3587 _ _ _] -> [_ w3636 _ _]
                  seq-local: [w3585 _ _ _] -> [_ w3634 _ _]
                  seq-local: [w3586 _ _ _] -> [_ w3635 _ _]
                  seq-local: [w3584 _ _ _] -> [_ w3633 _ _]
                  seq-local: [w3583 _ _ _] -> [_ w3628 _ _]
                  seq-local: [w3582 _ _ _] -> [_ w3629 _ _]
                  seq-local: [w3581 _ _ _] -> [_ w3630 _ _]
                  seq-local: [w3580 _ _ _] -> [_ w3631 _ _]
                  seq-local: [w3579 _ _ _] -> [_ w3632 _ _]
                  tunnel: w3578 -> [_ _ _ w3812]
                  tunnel: w3577 -> [_ _ _ w3795]
                  tunnel: w3576 -> [_ _ _ w3809]
                  tunnel: w3575 -> [_ _ _ w3808]
                  tunnel: w3574 -> [w3619 _ _ w3803]
                  tunnel: w3573 -> [_ _ w3754 _]
                  tunnel: w3572 -> [_ _ w3751 _]
                  tunnel: w3571 -> [_ _ w3750 _]
                  tunnel: w3570 -> [_ _ w3749 _]
                  tunnel: w3569 -> [_ _ w3748 _]
                  tunnel: w3568 -> [_ _ w3747 _]
                  tunnel: w3567 -> [_ _ w3746 _]
                  tunnel: w3566 -> [_ _ w3745 _]
                  tunnel: w3565 -> [_ _ w3744 _]
                  tunnel: w3564 -> [_ _ w3743 _]
                  frame #0 {
                    n2304 = case shown="False" w3619 {
                      frame False {
                        n2305 = local write "mail control"("") -> ()
                      }
                      frame True {
                      }
                    }
                    n2306 = local read "SET LAB01-1"() -> (w3618:T5)
                    n2307 = local read "SET LAB01-2"() -> (w3617:T5)
                    n2308 = local read "SET LAB02-1"() -> (w3616:T5)
                    n2309 = local read "SET LAB02-2"() -> (w3615:T5)
                    n2310 = local read "SET LAB03-1"() -> (w3614:T5)
                    n2311 = local read "SET LAB04-1"() -> (w3612:T5)
                    n2312 = local read "SET LAB05-1"() -> (w3610:T5)
                    n2313 = local read "SET LAB03-2"() -> (w3613:T5)
                    n2314 = local read "SET LAB04-2"() -> (w3611:T5)
                    n2315 = local read "SET LAB05-2"() -> (w3609:T5)
                    n2316 = Unbundle(w3614) -> ("DESCRIPTION"=w3594:string)  [unwired: 4 out]
                    n2317 = Unbundle(w3613) -> ("DESCRIPTION"=w3593:string)  [unwired: 4 out]
                    n2318 = Unbundle(w3612) -> ("DESCRIPTION"=w3592:string)  [unwired: 4 out]
                    n2319 = Unbundle(w3609) -> ("DESCRIPTION"=w3589:string)  [unwired: 4 out]
                    n2320 = Unbundle(w3615) -> ("DESCRIPTION"=w3595:string)  [unwired: 4 out]
                    n2321 = Unbundle(w3611) -> ("DESCRIPTION"=w3591:string)  [unwired: 4 out]
                    n2322 = Unbundle(w3618) -> ("DESCRIPTION"=w3607:string)  [unwired: 4 out]
                    n2323 = Unbundle(w3616) -> ("DESCRIPTION"=w3596:string)  [unwired: 4 out]
                    n2324 = Unbundle(w3610) -> ("DESCRIPTION"=w3590:string)  [unwired: 4 out]
                    n2325 = Unbundle(w3617) -> ("DESCRIPTION"=w3597:string)  [unwired: 4 out]
                    n2326 = Concatenate Strings("[LAB05-1/", w3589) -> (w3579:string)
                    n2327 = Concatenate Strings("[LAB05-2/", w3590) -> (w3580:string)
                    n2328 = Concatenate Strings("[LAB04-2/", w3591) -> (w3581:string)
                    n2329 = Concatenate Strings("[LAB03-2/", w3593) -> (w3583:string)
                    n2330 = Concatenate Strings("[LAB04-1/", w3592) -> (w3582:string)
                    n2331 = Concatenate Strings("[LAB03-1/", w3594) -> (w3584:string)
                    n2332 = Concatenate Strings("[LAB01-2/", w3597) -> (w3587:string)
                    n2333 = Concatenate Strings("[LAB02-2/", w3595) -> (w3585:string)
                    n2334 = Concatenate Strings("[LAB01-1/", w3607) -> (w3588:string)
                    n2335 = Concatenate Strings("[LAB02-1/", w3596) -> (w3586:string)
                  }
                  frame #1 {
                    w3641 = "/"
                    w3642 = 2.0
                    n2336 = local read "DISP LAB01-2"() -> (w3722:T4)
                    n2337 = local read "DISP LAB01-1"() -> (w3723:T4)
                    n2338 = local read "DISP LAB02-1"() -> (w3721:T4)
                    n2339 = local read "DISP LAB03-2"() -> (w3718:T4)
                    n2340 = local read "DISP LAB02-2"() -> (w3720:T4)
                    n2341 = local read "DISP LAB03-1"() -> (w3719:T4)
                    n2342 = local read "DISP LAB04-2"() -> (w3716:T4)
                    n2343 = local read "DISP LAB04-1"() -> (w3717:T4)
                    n2344 = local read "DISP LAB05-1"() -> (w3715:T4)
                    n2345 = local read "DISP LAB05-2"() -> (w3714:T4)
                    n2346 = Unbundle(w3722) -> ("CYCLE"=w3706:dbl, "MINS"=w3705:dbl, "STATUS"=w3702:string)
                    n2347 = Unbundle(w3723) -> ("CYCLE"=w3711:dbl, "MINS"=w3710:dbl, "STATUS"=w3707:string)
                    n2348 = Unbundle(w3721) -> ("CYCLE"=w3699:dbl, "MINS"=w3698:dbl, "STATUS"=w3697:string)
                    n2349 = Unbundle(w3718) -> ("CYCLE"=w3686:dbl, "MINS"=w3685:dbl, "STATUS"=w3682:string)
                    n2350 = Unbundle(w3719) -> ("CYCLE"=w3691:dbl, "MINS"=w3690:dbl, "STATUS"=w3687:string)
                    n2351 = Unbundle(w3720) -> ("CYCLE"=w3696:dbl, "MINS"=w3695:dbl, "STATUS"=w3692:string)
                    n2352 = Unbundle(w3717) -> ("CYCLE"=w3681:dbl, "MINS"=w3680:dbl, "STATUS"=w3677:string)
                    n2353 = Unbundle(w3716) -> ("CYCLE"=w3676:dbl, "MINS"=w3675:dbl, "STATUS"=w3672:string)
                    n2354 = Unbundle(w3715) -> ("CYCLE"=w3671:dbl, "MINS"=w3670:dbl, "STATUS"=w3667:string)
                    n2355 = Unbundle(w3714) -> ("CYCLE"=w3713:dbl, "MINS"=w3712:dbl, "STATUS"=w3664:string)
                    n2356 = Number To Decimal String(number=w3699) -> (decimal integer string=w3701:string)  [unwired: 1 in]
                    n2357 = Number To Decimal String(number=w3696) -> (decimal integer string=w3694:string)  [unwired: 1 in]
                    n2358 = Number To Decimal String(number=w3691) -> (decimal integer string=w3689:string)  [unwired: 1 in]
                    n2359 = Number To Decimal String(number=w3706) -> (decimal integer string=w3704:string)  [unwired: 1 in]
                    n2360 = Number To Decimal String(number=w3686) -> (decimal integer string=w3684:string)  [unwired: 1 in]
                    n2361 = Number To Decimal String(number=w3711) -> (decimal integer string=w3709:string)  [unwired: 1 in]
                    n2362 = Number To Decimal String(number=w3713) -> (decimal integer string=w3666:string)  [unwired: 1 in]
                    n2363 = Number To Decimal String(number=w3681) -> (decimal integer string=w3679:string)  [unwired: 1 in]
                    n2364 = Number To Decimal String(number=w3676) -> (decimal integer string=w3674:string)  [unwired: 1 in]
                    n2365 = Number To Decimal String(number=w3671) -> (decimal integer string=w3669:string)  [unwired: 1 in]
                    n2366 = Number To Fractional String(number=w3698, precision (6)=w3642) -> (F-format string=w3700:string)  [unwired: 2 in]
                    n2367 = Number To Fractional String(number=w3685, precision (6)=w3642) -> (F-format string=w3683:string)  [unwired: 2 in]
                    n2368 = Number To Fractional String(number=w3695, precision (6)=w3642) -> (F-format string=w3693:string)  [unwired: 2 in]
                    n2369 = Number To Fractional String(number=w3690, precision (6)=w3642) -> (F-format string=w3688:string)  [unwired: 2 in]
                    n2370 = Number To Fractional String(number=w3675, precision (6)=w3642) -> (F-format string=w3673:string)  [unwired: 2 in]
                    n2371 = Number To Fractional String(number=w3680, precision (6)=w3642) -> (F-format string=w3678:string)  [unwired: 2 in]
                    n2372 = Number To Fractional String(number=w3705, precision (6)=w3642) -> (F-format string=w3703:string)  [unwired: 2 in]
                    n2373 = Number To Fractional String(number=w3670, precision (6)=w3642) -> (F-format string=w3668:string)  [unwired: 2 in]
                    n2374 = Number To Fractional String(number=w3710, precision (6)=w3642) -> (F-format string=w3708:string)  [unwired: 2 in]
                    n2375 = Number To Fractional String(number=w3712, precision (6)=w3642) -> (F-format string=w3665:string)  [unwired: 2 in]
                    n2376 = Concatenate Strings(w3641, w3684, w3641, w3683, w3641, w3682) -> (w3658:string)
                    n2377 = Concatenate Strings(w3641, w3679, w3641, w3678, w3641, w3677) -> (w3657:string)
                    n2378 = Concatenate Strings(w3641, w3674, w3641, w3673, w3641, w3672) -> (w3656:string)
                    n2379 = Concatenate Strings(w3641, w3669, w3641, w3668, w3641, w3667) -> (w3655:string)
                    n2380 = Concatenate Strings(w3641, w3666, w3641, w3665, w3641, w3664) -> (w3654:string)
                    n2381 = Concatenate Strings(w3641, w3709, w3641, w3708, w3641, w3707) -> (w3663:string)
                    n2382 = Concatenate Strings(w3641, w3689, w3641, w3688, w3641, w3687) -> (w3659:string)
                    n2383 = Concatenate Strings(w3641, w3704, w3641, w3703, w3641, w3702) -> (w3662:string)
                    n2384 = Concatenate Strings(w3641, w3701, w3641, w3700, w3641, w3697) -> (w3661:string)
                    n2385 = Concatenate Strings(w3641, w3694, w3641, w3693, w3641, w3692) -> (w3660:string)
                    n2386 = Concatenate Strings("]", "\r") -> (w3638:string)
                    n2387 = Concatenate Strings(w3633, w3659, w3638) -> (w3649:string)
                    n2388 = Concatenate Strings(w3635, w3661, w3638) -> (w3651:string)
                    n2389 = Concatenate Strings(w3634, w3660, w3638) -> (w3650:string)
                    n2390 = Concatenate Strings(w3630, w3656, w3638) -> (w3646:string)
                    n2391 = Concatenate Strings(w3631, w3655, w3638) -> (w3647:string)
                    n2392 = Concatenate Strings(w3629, w3657, w3638) -> (w3645:string)
                    n2393 = Concatenate Strings(w3628, w3658, w3638) -> (w3644:string)
                    n2394 = Concatenate Strings(w3632, w3654, w3638) -> (w3648:string)
                    n2395 = Concatenate Strings(w3636, w3662, w3638) -> (w3652:string)
                    n2396 = Concatenate Strings(w3637, w3663, w3638) -> (w3653:string)
                    n2397 = Concatenate Strings(w3653, w3652, w3651, w3650, w3649, w3644, w3645, w3646, w3647, w3648) -> (w3621:string)
                    n2398 = Concatenate Strings("[PANEL/", "DESC/", "CYCLES/", "MINS/", "STATUS]", "\r", w3621) -> (w3643:string)
                    "MAIL REPORT" <- w3643
                  }
                  frame #2 {
                    w3752 = "END"
                    n2399 = local read "mail control"() -> (w3753:string)
                    n2400 = case shown="False" w3748 {
                      tunnel: w3753 -> [w3777 _]
                      tunnel: w3752 -> [w3776 _]
                      tunnel: [w3775 FALSE] -> w3738
                      frame False {
                        n2401 = Equal?(x=w3777, y=w3776) -> (x = y?=w3775:bool)
                      }
                      frame True {
                      }
                    }
                    n2402 = case shown="False" w3754 {
                      tunnel: w3753 -> [w3793 _]
                      tunnel: w3752 -> [w3792 _]
                      tunnel: [w3791 FALSE] -> w3742
                      frame False {
                        n2403 = Equal?(x=w3793, y=w3792) -> (x = y?=w3791:bool)
                      }
                      frame True {
                      }
                    }
                    n2404 = case shown="False" w3751 {
                      tunnel: w3753 -> [w3789 _]
                      tunnel: w3752 -> [w3788 _]
                      tunnel: [w3787 FALSE] -> w3741
                      frame False {
                        n2405 = Equal?(x=w3789, y=w3788) -> (x = y?=w3787:bool)
                      }
                      frame True {
                      }
                    }
                    n2406 = case shown="False" w3749 {
                      tunnel: w3753 -> [w3781 _]
                      tunnel: w3752 -> [w3780 _]
                      tunnel: [w3779 FALSE] -> w3739
                      frame False {
                        n2407 = Equal?(x=w3781, y=w3780) -> (x = y?=w3779:bool)
                      }
                      frame True {
                      }
                    }
                    n2408 = case shown="False" w3750 {
                      tunnel: w3753 -> [w3785 _]
                      tunnel: w3752 -> [w3784 _]
                      tunnel: [w3783 FALSE] -> w3740
                      frame False {
                        n2409 = Equal?(x=w3785, y=w3784) -> (x = y?=w3783:bool)
                      }
                      frame True {
                      }
                    }
                    n2410 = Or(x=w3740, y=w3739) -> (x .or. y?=w3731:bool)
                    n2411 = Or(x=w3742, y=w3741) -> (x .or. y?=w3732:bool)
                    n2412 = Or(x=w3732, y=w3731) -> (x .or. y?=w3727:bool)
                    n2413 = case shown="False" w3744 {
                      tunnel: w3753 -> [w3761 _]
                      tunnel: w3752 -> [w3760 _]
                      tunnel: [w3759 FALSE] -> w3733
                      frame False {
                        n2414 = Equal?(x=w3761, y=w3760) -> (x = y?=w3759:bool)
                      }
                      frame True {
                      }
                    }
                    n2415 = case shown="False" w3743 {
                      tunnel: w3753 -> [w3757 _]
                      tunnel: w3752 -> [w3756 _]
                      tunnel: [w3755 FALSE] -> w3737
                      frame False {
                        n2416 = Equal?(x=w3757, y=w3756) -> (x = y?=w3755:bool)
                      }
                      frame True {
                      }
                    }
                    n2417 = case shown="False" w3745 {
                      tunnel: w3753 -> [w3765 _]
                      tunnel: w3752 -> [w3764 _]
                      tunnel: [w3763 FALSE] -> w3734
                      frame False {
                        n2418 = Equal?(x=w3765, y=w3764) -> (x = y?=w3763:bool)
                      }
                      frame True {
                      }
                    }
                    n2419 = case shown="False" w3747 {
                      tunnel: w3753 -> [w3773 _]
                      tunnel: w3752 -> [w3772 _]
                      tunnel: [w3771 FALSE] -> w3736
                      frame False {
                        n2420 = Equal?(x=w3773, y=w3772) -> (x = y?=w3771:bool)
                      }
                      frame True {
                      }
                    }
                    n2421 = case shown="False" w3746 {
                      tunnel: w3753 -> [w3769 _]
                      tunnel: w3752 -> [w3768 _]
                      tunnel: [w3767 FALSE] -> w3735
                      frame False {
                        n2422 = Equal?(x=w3769, y=w3768) -> (x = y?=w3767:bool)
                      }
                      frame True {
                      }
                    }
                    n2423 = Or(x=w3736, y=w3735) -> (x .or. y?=w3730:bool)
                    n2424 = Or(x=w3734, y=w3733) -> (x .or. y?=w3729:bool)
                    n2425 = Or(x=w3737, y=w3738) -> (x .or. y?=w3725:bool)
                    n2426 = Or(x=w3730, y=w3729) -> (x .or. y?=w3728:bool)
                    n2427 = Or(x=w3727, y=w3728) -> (x .or. y?=w3726:bool)
                    n2428 = Or(x=w3726, y=w3725) -> (x .or. y?=w3724:bool)
                  }
                  frame #3 {
                    n2429 = local read "on loops"() -> (w3807:dbl)
                    n2430 = local read "jig cycle"() -> (w3804:dbl)
                    n2431 = local read "Send Mail Now"() -> (w3798:bool)
                    n2432 = Add(x=w3807, y=3.0) -> (x+y=w3805:dbl)
                    n2433 = Equal?(x=w3804, y=w3805) -> (x = y?=w3799:bool)
                    n2434 = And(x=w3799, y=w3798) -> (x .and. y?=w3797:bool)
                    n2435 = And(x=w3803, y=w3799) -> (x .and. y?=w3802:bool)
                    n2436 = And(x=w3802, y=w3801) -> (x .and. y?=w3800:bool)
                    n2437 = Or(x=w3800, y=w3797) -> (x .or. y?=w3796:bool)
                    n2438 = case shown="True" w3796 {
                      tunnel: w3812 -> [_ w3818]
                      tunnel: w3811 -> [_ w3817]
                      tunnel: "Lab Panel Test Status" -> [_ w3816]
                      tunnel: w3809 -> [_ w3815]
                      tunnel: w3808 -> [_ w3814]
                      tunnel: w3795 -> [_ w3813]
                      frame False {
                      }
                      frame True {
                        n2439 = stacked-sequence {
                          tunnel: w3818 -> [w3826 _]
                          tunnel: w3817 -> [w3825 _]
                          tunnel: w3816 -> [w3824 _]
                          tunnel: w3815 -> [w3823 _]
                          tunnel: w3814 -> [w3822 _]
                          tunnel: w3813 -> [w3821 _]
                          frame #0 {
                            n2440 = call "sub vi - send mail with attach v5.vi"("TO:"=w3826, "subject"=w3824, "from"=w3822, "out going server"=w3823, "message"=w3825) -> ("error out"=w3820:errorcluster)  [unwired: 10 in]
                            n2441 = Bundle(cluster=w3821, "mail error"=w3820) -> (w3819:T6)  [unwired: 6 in]
                            n2442 = local write "MAIL SETTINGS"(w3819) -> ()
                          }
                          frame #1 {
                            n2443 = local write "mail control"("") -> ()
                            n2444 = local write "Send Mail Now"(FALSE) -> ()
                          }
                        }
                      }
                    }
                  }
                }
              }
            }
          }
        }
        n2445 = node-c288() -> ()  [unwired: 1 in, 1 out]
        "loops" <- w165
        "stop2" <- "stop"
      }
      n2446 = node-c288(w142) -> ()  [unwired: 1 out]
    }
  }
